vi "Main.vi"() -> ()   [LabVIEW 2013]
uses:
  MouseCarousel/Controls/TrainingProtocols.ctl
  MouseCarousel/States/DataAquisitionStates.ctl
  <vilib>/vision/Avi.llb/IMAQ AVI2 Refnum.ctl
  <vilib>/vision/Image Controls.llb/IMAQ Image.ctl
  MouseCarousel/Controls/sessionInfoAR.ctl
  MouseCarousel/Controls/dataInfo.ctl
  <vilib>/event_ctls.llb/eventsource.ctl
  Instruments/StepperController.lvclass
  D:/Labview Programs/PassiveRotationTask/trialData.ctl
  MouseCarousel/Checklists/SessionChecklist.ctl
  MouseCarousel/Checklists/OpenCarouselInitializationChecklist.ctl
  MouseCarousel/States/EventLoopStates.ctl
  MouseCarousel/States/MainProgramStates.ctl
  SecurityCamera/SecurityCameraStates.ctl
  PupilTracker/PupilTrackerStates.ctl
  RotationControl/StageLoggingStates.ctl
  MouseCarousel/States/RotationStageStates.ctl
  Utility/Load and Save Controls_LV2009.llb/RWC_Actions.ctl
  <vilib>/DAQmx/write.llb/DAQmx Write (Digital Bool 1Line 1Point).vi
  <vilib>/DAQmx/read.llb/DAQmx Read (Digital 2D U8 NChan NSamp).vi
  MouseCarousel/GlobalVariables.vi
  <vilib>/DAQmx/create/channels.llb/DAQmx Create Channel (DO-Digital Output).vi
  <vilib>/DAQmx/miscellaneous.llb/DAQmx Fill In Error Info.vi
  <vilib>/Utility/xml.llb/Write to XML File(string).vi
  <vilib>/DAQmx/create/channels.llb/DAQmx Create Channel (DI-Digital Input).vi
  <vilib>/DAQmx/configure/timing.llb/DAQmx Timing (Sample Clock).vi
  <vilib>/DAQmx/configure/task.llb/DAQmx Configure Logging (TDMS).vi
  <vilib>/Analysis/NI_AALBase.lvlib
  <vilib>/vision/NI_Vision_Development_Module.lvlib
  <resource>/objmgr/daqmx.rc
  <vilib>/DAQmx/configure/timing.llb/DAQmx Timing (Change Detection).vi
  <vilib>/DAQmx/configure/trigger.llb/DAQmx Start Trigger (Digital Edge).vi
  <vilib>/DAQmx/create/channels.llb/DAQmx Create Channel (AI-Voltage-Basic).vi
  <vilib>/DAQmx/read.llb/DAQmx Read (Counter U32 1Chan 1Samp).vi
  <vilib>/DAQmx/read.llb/DAQmx Read (Analog DBL 1Chan 1Samp).vi
  <vilib>/DAQmx/create/channels.llb/DAQmx Create Channel (CI-Position-Angular Encoder).vi
panel:
  in  "Show Mouse ROI":bool
  out "Security Camera":T1(plugin-control)
  in  "Select Mouse ROI":bool
  out "Lost Frames":bool
  out "Recording Security Video":bool caption="Recording"
  out "RecordingID":string
  out "Last Image number":u32
  out "mL Per Ms":dbl=1.25e-05
  out "trial data tdms fileref":refnum<k34>
  out "Last Count":u32
  out "Trial Distance":i32[][](array[numeric])
  in  "Is Setup Initialized":bool
  in  "Recording No":i32=1
  in  "Session Checklist":T2
  out "Trial Speeds":i32[][](array[numeric])
  in  "trialData":T3
  out "wall ref":bool
  out "Stage Moving?":bool caption="Moving?"
  out "Wall Moving?":bool caption="Moving?"
  in  "Reset":bool
  in  "Quit":bool
  in  "Print Screen":bool
  out "Stage Position":dbl caption="Position"
  out "StepperController.lvclass":refnum<class "StepperController.lvclass">
  out "Mask":T1
  out "Fitted Pupil Image 2":T1
  out "BIN Refnum - Body":refnum<file>
  out "FrameCount":dbl
  out "Refnum out (duplicate)":T1
  out "Recording Demo Video":bool=TRUE
  out "DemoVideo":T1(plugin-control)
  out "channel names":string[](array[string])=["Licks", "Beeps", "Water", "2P Frames", "LightOnOff", "Stage Position", "Stage Moving", "Wall Position", "Wall Moving", "Trial Counter", "Trial State", "Pupil Sample No"]
  out "Source":T4 items=["LabVIEW UI"=0, "ActiveX"=1, "User Event"=25]
  out "ImageSummaryPath":path
  out "Session Running":bool=TRUE
  out "Mouse entered arena":string
  out "Response Window":dbl
  out "security camera error":errorcluster
  in  "dataInfo":T5
  in  "Save Security Video":bool
  in  "Save Pupil Video":bool=TRUE
  in  "response window is open":bool=TRUE
  out "LostFrames":u32 caption="LostFrames Pupil Camera"
  out "Frame Rate Security Cam":dbl
  out "LostFrames Security Camera":u32
  out "arena_display":T1
  out "mouse":T1
  out "tmp_arena":T1
  out "tmp_mouse":T1
  out "arena":T1
  out "Paused Acquisition":bool=TRUE
  in  "ArenaState":T6={"Stage Position"=0.0, "Stage Moving?"=TRUE, "Wall Position"=0.0, "Wall Moving"=TRUE}
  in  "sessionInfo":T7
  out "GoogleDriveFolder":path
  out "RecordingFolder":path
  out "Log Stage Positions":bool=TRUE
  out "Stage Rotation Direction":bool caption="Moving?"
  in  "Block folder":path
  out "Processed Image":T1
  out "Cropped Image":T1
  out "Processed Image Display":T1
  out "Fitted Pupil Image":T1
  out "Stop Acquisition":bool=TRUE
  out "Vision Acquisition Error":errorcluster
  in  "Save Tracking Results":bool=TRUE
  out "Pupil Sample No":i32
  out "Last Image number SV":u32
  out "Mouse mask":T1
  out "AVI Refnum - Body":T8
  out "Trigger microscope":bool=TRUE
  out "2P TriggerLine":refnum<k21>
  out "SciScan RecordSignal":refnum<k21>
  out "Session Performance":i16[][](array[numeric])
  in  "PrevLickState":dbl format="%#_13g"
  out "tmpNCorrect":i32
  out "nCorrect":i32
  out "Correct?":bool
  out "Trial State":i32
  out "Recording Start Time":u32
  out "Saved Values":refnum<vi>[](array[refnum])
  out "tdms file performance":refnum<k34>
  out "Licked":bool=TRUE
  out "Response Timeout":bool=TRUE
  in  "Tab Control":T9(tab)
  out "Image Size":string
  out "Frames Lost":bool
  in  "Give Water 2":bool
  in  "Step+":bool
  in  "Step-":bool
  in  "Home":bool
  in  "Compress Avi":bool
  in  "Rotate Full":bool
  in  "Align Stage":bool
  in  "Start Protocol":bool
  in  "Selected Training Protocol":T10=enum."Rotations - Speed 45 deg/s"
  in  "Pause":bool
  in  "Open Checklist":bool
  in  "Abort Protocol":bool
  out "Image":T1(plugin-control)
  in  "Day":u16
  in  "Airpuff":bool
  in  "Mouse Entered":bool
  out "Lick Rates":i32[][](graph)
  out "Trial Performance":cluster{"D'prime":dbl, "pCorrect":dbl}(graph)
  out "Trial Outcomes":i16[](graph)
  out "Lick detection":cluster{dbl, dbl, dbl[][]}(graph)
  out "Trial Counter":i32
  out "NRewards":i32
  out "NGoTrials":i32
  out "% correct":dbl format="%#_2g"
  out "d'":dbl
  out "Last trial":i32=300
  out "SessionID":string
  in  "Give Water":bool
  in  "Lights On":bool
  in  "Mouse Number":i32
  out "Stage Position 2":T1(plugin-control)
  out "Pupil Info":T11(graph)
  out "Intertrial Interval":bool
  out "Time Delay":bool
  out "Response Window":bool
  out "Pre trial":bool
  out "Cue":bool
  out "Current trial":string caption="Trial Progression"
  out "mL given":dbl(slide) scale=0.0..1.0
  out "last response time (ms)":dbl
  out "Go Trial?":bool=TRUE
  out "NPunishments":i32
  in  "Experiment Name":string="PassiveRotationTask"
  in  "SS Crash Button":bool
  in  "MC Crash Button":bool
  out "stageStopPosition":dbl
  out "stageAcceleration":dbl
  out "Pupil marked":bool=TRUE
  out "Frame Rate Eyetracker":dbl caption="FPS"
  in  "xFactorStdThresholding":dbl=1.0 min=0.0 max=5.0 step=0.1
  in  "Automatic Threshold Update":bool
  out "Avg freq":dbl caption="Eyetracker - Mean \nprocessing frequency (Hz)" format="%0.2f"
  out "PupilCamera":T1(plugin-control)
  out "Tracking Pupil":bool
  out "Recording Pupil Video":bool=TRUE
  out "Processed":T1(plugin-control)
  in  "Manual Threshold":cluster{sgl, sgl}(slide)={196.0, 255.0} caption="Threshold Range" scale=0.0..255.0
  in  "Exposure Time":dbl(slide)=15144.329896907217 min=10.0 max=850000.0 scale=1000.0..16000.0
  in  "Gain":dbl(slide)=8.879999999999999 min=0.0 max=24.0 step=1.0 scale=0.0..24.0
  in  "Black Level":dbl(slide)=0.9896907216494839 min=-32.0 max=31.75 scale=-32.0..32.0
  in  "Track Pupil":bool
  in  "Rescan Image":bool
  in  "Acquisition Frame Rate":dbl=60.0 min=1.0 max=100000.0
  in  "Track Every Nth Frame":i32=2
  out "Auto Threshold":sgl[](array[numeric])
  out "Reset Lost Frames":bool
  in  "Select Pupil Area":bool
  in  "BtnStageSmallStep":bool
  in  "BtnWallSetHome":bool
  in  "BtnWallMoveHome":bool
  in  "Wall step size (deg)":dbl=90.0 min=-45.0 max=45.0 step=1.0
  in  "Wall Acceleration (deg2/s)":dbl=200.0 min=1.0 max=1000.0 step=1.0
  in  "Wall Speed (deg/s)":dbl=50.0 min=0.1 max=50.0 step=0.1
  in  "BtnWallStepCW":bool
  in  "BtnWallStepCCW":bool
  in  "BtnStage180CW":bool
  in  "BtnStage180CCW":bool
  in  "BtnStageMoveHome":bool
  in  "Stage step size (deg)":dbl=90.0
  in  "Stage Acceleration (deg2/s)":dbl=200.0
  in  "Stage Speed (deg/s)":dbl=50.0
  in  "BtnStageStepCW":bool
  in  "BtnStageStepCCW":bool
  in  "Move to ...":bool=TRUE
  in  "... Position":dbl
  out "Wall Position":dbl caption="Position" format="%#.2f"
  in  "BtnBothCW":bool
  in  "BtnBothCCW":bool
  in  "Save Trial Data":bool
  in  "Wall Speed Selection":dbl[](array[numeric])=[45.0, 90.0]
  in  "Stage Speed Selection":dbl[](array[numeric])=[45.0, 90.0, 135.0, 180.0]
  in  "DarkProbes":bool
  in  "Airpuff (ms)":u32=400
  in  "Always Puff":bool=TRUE
  in  "Intertrial interval (s)":i32=6
  in  "Punishment Period (s)":i32
  in  "Response Window (ms)":u32=2000
  in  "Go Trial Probability":dbl=0.5 min=0.0 max=1.0 step=0.1
  in  "nTrials":i32=100
  in  "Give water":bool
  in  "Delay (ms)":i32=500
  in  "LightsOnSession":bool=TRUE
  in  "Baseline Period (s)":i32=30
  in  "Wall-Stage delay (ms)":dbl=33.0
  in  "Wall max rotation":dbl=720.0
  in  "Wall physical step size (deg/step)":dbl=0.139
  in  "DAQmx step counter":tag="Dev1/ctr0"
  in  "DAQmx step terminal":tag="/Dev1/PFI8"
  in  "DAQmx step-dir line":tag="Dev1/port2/line1"
  in  "Save Pupil Video As...":enum16{"BIN", "PNG", "AVI"}(ring)
  in  "Save Security Video As...":enum16{"BIN", "AVI"}(ring)=enum."AVI"
  in  "DemoCamera Connected":bool caption="Demo Camera Connected"
  in  "Sampling - Labels,  Lines In":string[][](array[string])=[["Licks", "Dev1/port0/line3", "", ""], ["Airpuff", "Dev1/port0/line4", "", ""], ["Water", "Dev1/port0/line7", "", ""], ["2P Frames", "Dev1/port0/line2", "", ""], ["Light", "Dev1/port0/line0", "", ""], ["Wall Pos Reset", "Dev1/port0/line6", "Light", "Light"]]
  in  "Select Microscope":enum16{"Prairie", "SciScan"}(ring)=enum."SciScan"
  in  "Two Photon Connected":bool=TRUE caption="Two Photon Microscope"
  in  "Lick Port Connected":bool=TRUE caption="Lick Port"
  in  "Open Valve":bool
  in  "Sample Rate":dbl=5000.0 format="%#_13g"
  in  "Graph Update Rate (fps)":dbl=200.0 format="%#_13g"
  in  "Graph Length (s)":dbl=10.0 format="%#_13g"
  in  "Stage connected":bool=TRUE caption="Rotation Stage"
  in  "Calibrate Valve":bool
  in  "Valve opening time (ms)":u32=200
  in  "Number of drops to release":i32=100
  out "Valve opening time (last calibration) (ms)":u32
  out "Last Calibration Date":timestamp format="%<%H:%M:%S\n%x>T"
  out "mlPerDrop":dbl
  out "Start Data Logging":bool=TRUE
  out "Stop Data Logging":bool=TRUE
  out "Leave Acquisition Run State":T12=enum."Quit Data Acquisition"
  out "Logging Data":bool=TRUE
  in  "Security Camera Connected":bool=TRUE caption="Security Camera"
  in  "File Path for Mouse Mask":path=path "F:/RotationStageExperiments/MousePositionMask.bmp"
  in  "Select Rotation Stage":enum16{"PI", "Steinmeyer"}(ring)=enum."Steinmeyer"
  in  "Pupil Camera Connected":bool=TRUE caption="Pupil Camera"
  out "PIAxisID":string[](array[string])
  in  "Daily Summary Path":path=path "C:/Users/Eivind/Google Drive/Lab/Eivind Hennestad/Mouse Training/Round 5 - Training + imaging/DailySummaries"
  in  "Water Valve Line":tag="Dev1/port2/line3"
  in  "Airpuff Line":tag="Dev1/port2/line2"
  in  "Two-Photon trigger line":tag="Dev1/port2/line5"
  in  "SciScan Start/Stop":tag="Dev1/port1/line2"
  in  "Stage Position Limit":i32=720
  in  "Data Storage Folder":path=path "E:/NEW"
  out "Progress %":i32(slide) scale=0.0..100.0
  out "LickPerMin":i32[][](array[numeric])
  out "NLicks":i32[](array[numeric])
  in  "RoofLights":tag="Dev1/port1/line0"
  in  "Reward Punishment Ratio":u8=3
  in  "SaveDemoVideo":bool
  in  "Wall connected":bool=TRUE
  out "Stepper Prepared for Rotation":bool=TRUE
  out "Init Stepper Move":bool
  in  "Destretch Calibrate":bool
  in  "Release Air":bool
  out "Start Matlab Processing":bool
  out "Pandoras Box 2":bool
  out "Pressurized Air Supply  2":bool
  out "Encoder Splitter Power 2":bool
  in  "Startup Checklist":T13
  out "response time":u32
  out "Mouse Performance":i16[][](array[numeric])
  out "Correct Rejection":bool=TRUE
  out "Miss":bool=TRUE
  in  "Reward Green Light":bool=TRUE
  out "Reward Mode":enum16{"Reward on Cue", "Reward on Lick"}(ring)
  out "False Alarm":bool=TRUE
  out "Hit":bool=TRUE
  out "AllowReward":bool=TRUE
  out "Current Protocol":enum16{""}(ring)
  out "NDropsCalibration":i32
  out "Buffer Length":i32
  out "Samples to Read":i32
  in  "Exit Program":bool
  out "Response Times":dbl[](array[numeric])
  out "Waiting for lick":bool
  out "cue time":u32
  # "Training/Experiment"
  # "Session Info"
  # "Training Info"
  # "Hit"
  # "Correct Reject"
  # "Miss"
  # "False Alarm"
  # "Optimize Tracking"
  # "Set tracker to rescan entire image if pupil is not found within search area"
  # "Tracker Settings"
  # "Stage controls"
  # "NB! Is cable for roof light disconnected?"
  # "Wall controls"
  # "Move both"
  # "Training Parameters"
  # "Give water on \nevery go trial"
  # "Speed Modulation Sessions"
  # "Connection Settings"
  # "Equipment Selection"
  # "DAQ Connections"
  # "Settings"
  # "Acquisition"
  # "Graph Display"
  # "Data Storage Paths"
  # "Valve Calibration"
  # "Checklist Startup - Things to do before picking up mouse"
  # "Checklist Shutdown"
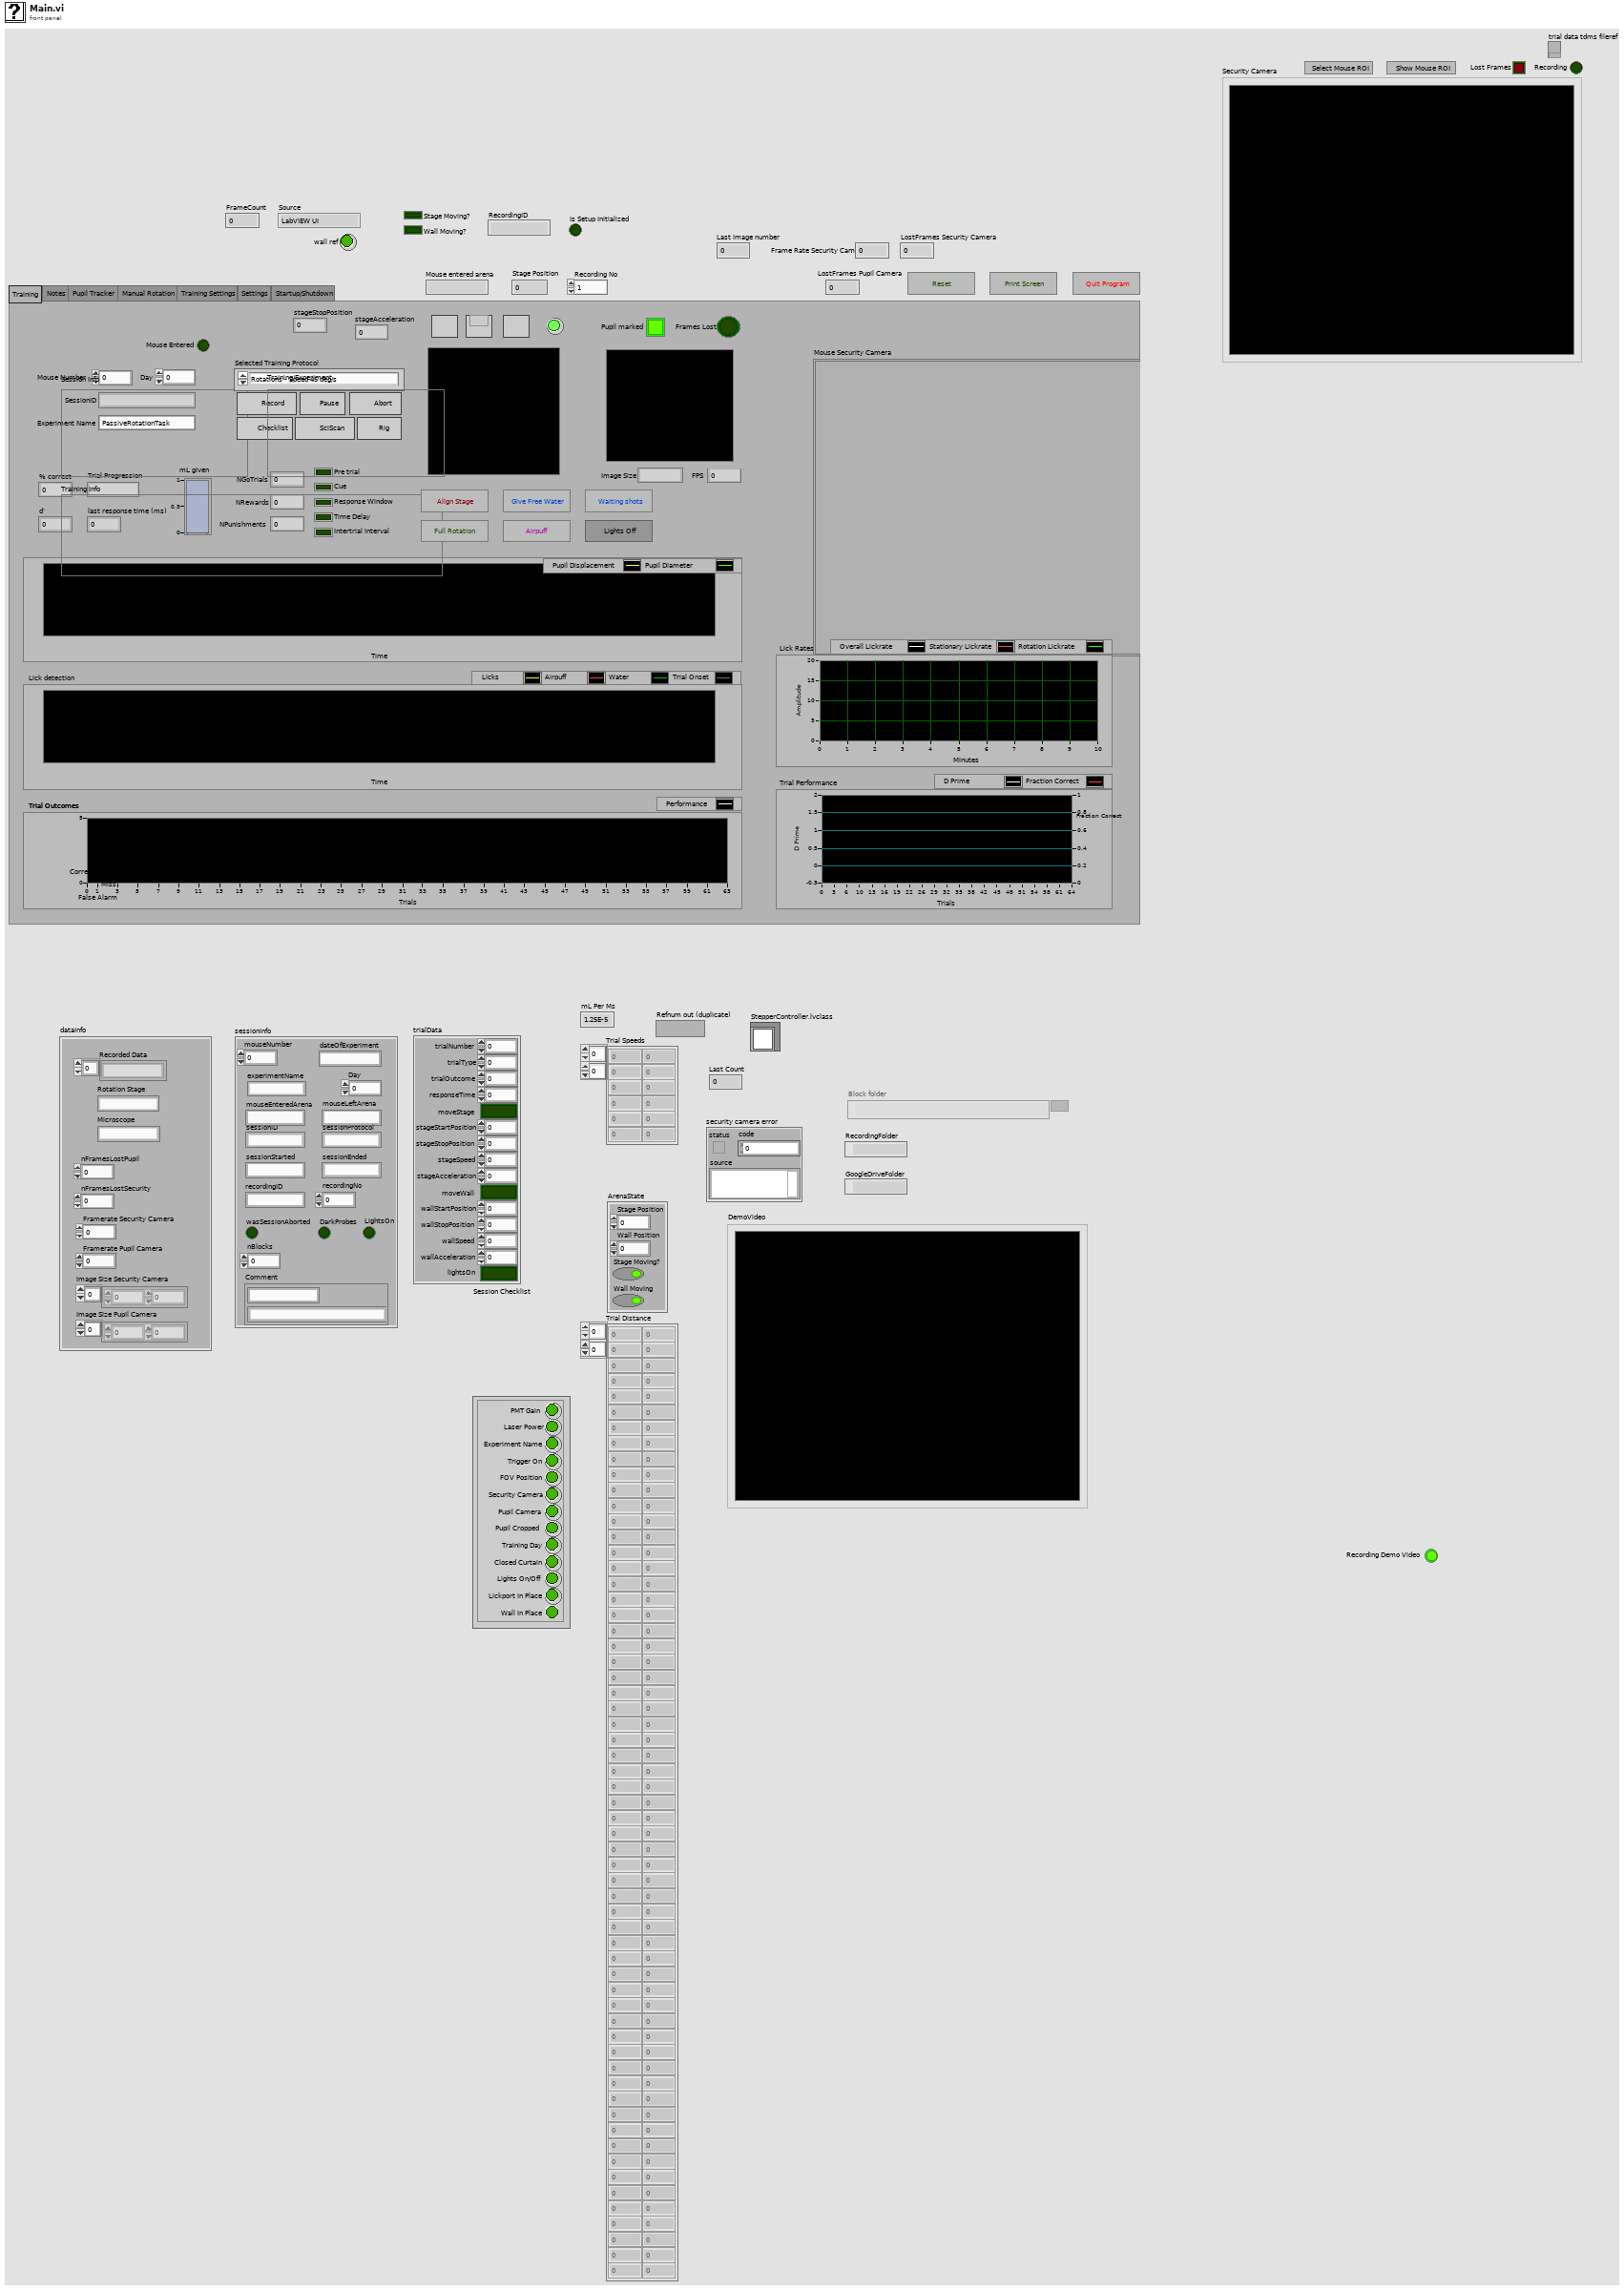
[diagram p1: front panel]
types:
  T1 = typedef "IMAQ Image.ctl" = refnum<image>
  T2 = typedef "SessionChecklist.ctl" = cluster{"PMT Gain":bool, "Laser Power":bool, "Experiment Name":bool, "Trigger On":bool, "FOV Position":bool, "Security Camera":bool, "Pupil Camera":bool, "Pupil Cropped":bool, "Training Day":bool, "Closed Curtain":bool, "Lights On/Off":bool, "Lickport In Place":bool, "Wall In Place":bool}
  T3 = typedef "trialData.ctl" = cluster{"trialNumber":i32, "trialType":i32, "trialOutcome":i32, "responseTime":i32, "moveStage":bool, "stageStartPosition":dbl, "stageStopPosition":dbl, "stageSpeed":dbl, "stageAcceleration":dbl, "moveWall":bool, "wallStartPosition":dbl, "wallStopPosition":dbl, "wallSpeed":dbl, "wallAcceleration":dbl, "lightsOn":bool}
  T4 = typedef "eventsource.ctl" = u32
  T5 = typedef "dataInfo.ctl" = cluster{"Recorded Data":string[], "Rotation Stage":string, "Microscope":string, "nFramesLostPupil":u32, "nFramesLostSecurity":u32, "Framerate Security Camera":dbl, "Framerate Pupil Camera":dbl, "Image Size Security Camera":i32[], "Image Size Pupil Camera":i32[]}
  T6 = cluster{"Stage Position":dbl, "Stage Moving?":bool, "Wall Position":dbl, "Wall Moving":bool}
  T7 = typedef "sessionInfoAR.ctl" = cluster{"mouseNumber":i32, "dateOfExperiment":string, "experimentName":string, "Day":u16, "mouseEnteredArena":string, "mouseLeftArena":string, "sessionID":string, "sessionProtocol":string, "sessionStarted":string, "sessionEnded":string, "recordingID":string, "recordingNo":i32, "wasSessionAborted":bool, "DarkProbes":bool, "LightsOn":bool, "nBlocks":i32, "Comment":cluster{"Title":string, "Comment":string}}
  T8 = typedef "IMAQ AVI2 Refnum.ctl" = refnum<k20>
  T9 = enum32{"Training", "Notes", "Pupil Tracker", "Manual Rotation", "Training Settings", "Settings", "Startup/Shutdown"}
  T10 = typedef "TrainingProtocols.ctl" = enum16{"Prerecording", "PRT Stage - 3Pos - 2Speeds", "PRT Wall - 3Pos - 2Speeds", "Rotations - Speed 45 deg/s", "Rotations - Speed 90 deg/s", "Wall Rotations - Speed 45deg/s", "Speed Modulation - Constant Duration", "Speed Modulation - Constant Distance", "Speed Modulation - Dark - Constant Distance", "Speed Modulation - Wall - Constant Distance", "Start-Stop", "Start-Stop-90", "4Accelerations", "Rotations - Random speeds", "Open Arena - Small Steps 2", "Open Arena - Small Steps", "Rotations - 240deg 60deg/s", "Free Water"}
  T11 = cluster{"Numeric":dbl, "Average of last N array elements":dbl}
  T12 = typedef "DataAquisitionStates.ctl" = enum16{"Init Data Acquisition", "Start Data Logging", "End Data Logging", "Run Data Acquisition", "Quit Data Acquisition"}
  T13 = typedef "OpenCarouselInitializationChecklist.ctl" = cluster{"Encoder Splitter Power":bool, "Pandoras Box":bool, "Water and Calibration":bool, "Vacuum Arena":bool, "Wall Power Supply":bool, "Wall Position Encoder":bool, "Stage Power Supply":bool}
  T14 = typedef "RotationStageStates.ctl" = enum16{"Connect Stage", "Get Stage Info", "Disconnect Stage"}
  T15 = typedef "StageLoggingStates.ctl" = enum16{"Initialize Arena State Logging", "Idle", "SteinmeyerV2", "Steinmeyer", "PI", "Logging Error"}
  T16 = typedef "PupilTrackerStates.ctl" = enum16{"Initialize Eyetracker", "Idle", "Run Acquisition", "Update Acquisition Parameters", "Camera Error", "Pupil Unmarked Error", "Quit Eyetracker"}
  T17 = typedef "SecurityCameraStates.ctl" = enum16{"Init Security Camera", "Idle", "Process Image", "Acquire Image", "Disconnect Camera", "Exit"}
  T18 = typedef "MainProgramStates.ctl" = enum16{"Init Main Program", "Load Modules", "Idle", "Reset Parameters", "Start Recording", "Init Training Protocol", "Baseline Period", "Trial Initialization", "Move Stage / Wall", "Cue", "Response Window", "Time Delay (Punishment)", "Intertrial Interval", "End Training Protocol", "End Recording", "Reset Session Data", "Pause", "Calibrate Water Valve", "Quit Main Program"}
  T19 = typedef "EventLoopStates.ctl" = enum16{"Init Event Loop", "Running", "Quit Event Loop"}
  T20 = typedef "Image Type" = u32
  T21 = cluster{"EOF Change Detection Task":refnum<k21>, "EOF Event":refnum<event-registration>}
  T22 = enum8{"Enabled", "Disabled", "Disabled and Grayed Out"}
  T23 = typedef "RWC_Actions.ctl" = enum16{"Read", "Write", "Read and Create"}
  T24 = enum16{"open", "open or create", "create or replace", "create", "open (read-only)"}
  T25 = enum16{"open", "replace", "create", "open or create", "replace or create", "replace or create with confirmation"}
  T26 = cluster{"Water Valve":refnum<k21>, "Airpuff":refnum<k21>, "Light Switch":refnum<k21>}
  T27 = enum32{"Invalid", "Standard", "Closed", "Hidden", "Minimized", "Maximized"}
  T28 = enum32{"Bad", "Idle", "Run top level", "Running"}
  T29 = typedef "IMAQ Rectangle" = cluster{"Left":i32, "Top":i32, "Right":i32, "Bottom":i32, "Rotation":dbl}
  T30 = cluster{"Numeric":dbl, "Average of last N array elements":dbl}[]
  T31 = typedef "TrackingParameters.ctl" = cluster{"Frame No":i32, "Circle time series":dbl[][], "Rectangle coordinates":i32[], "Annulus ROI":cluster{"ID":enum32{"External", "Internal"}, "Type":u32, i32[]}, "Initial Annulus":i32[], "Auto Threshold":sgl[], "Automatic Threshold Update":bool, "Initial Threshold":sgl[], "mFactorStd":dbl}
  T32 = cluster{"Pupil Displacement":dbl, "Average Pupil Diameter":dbl}
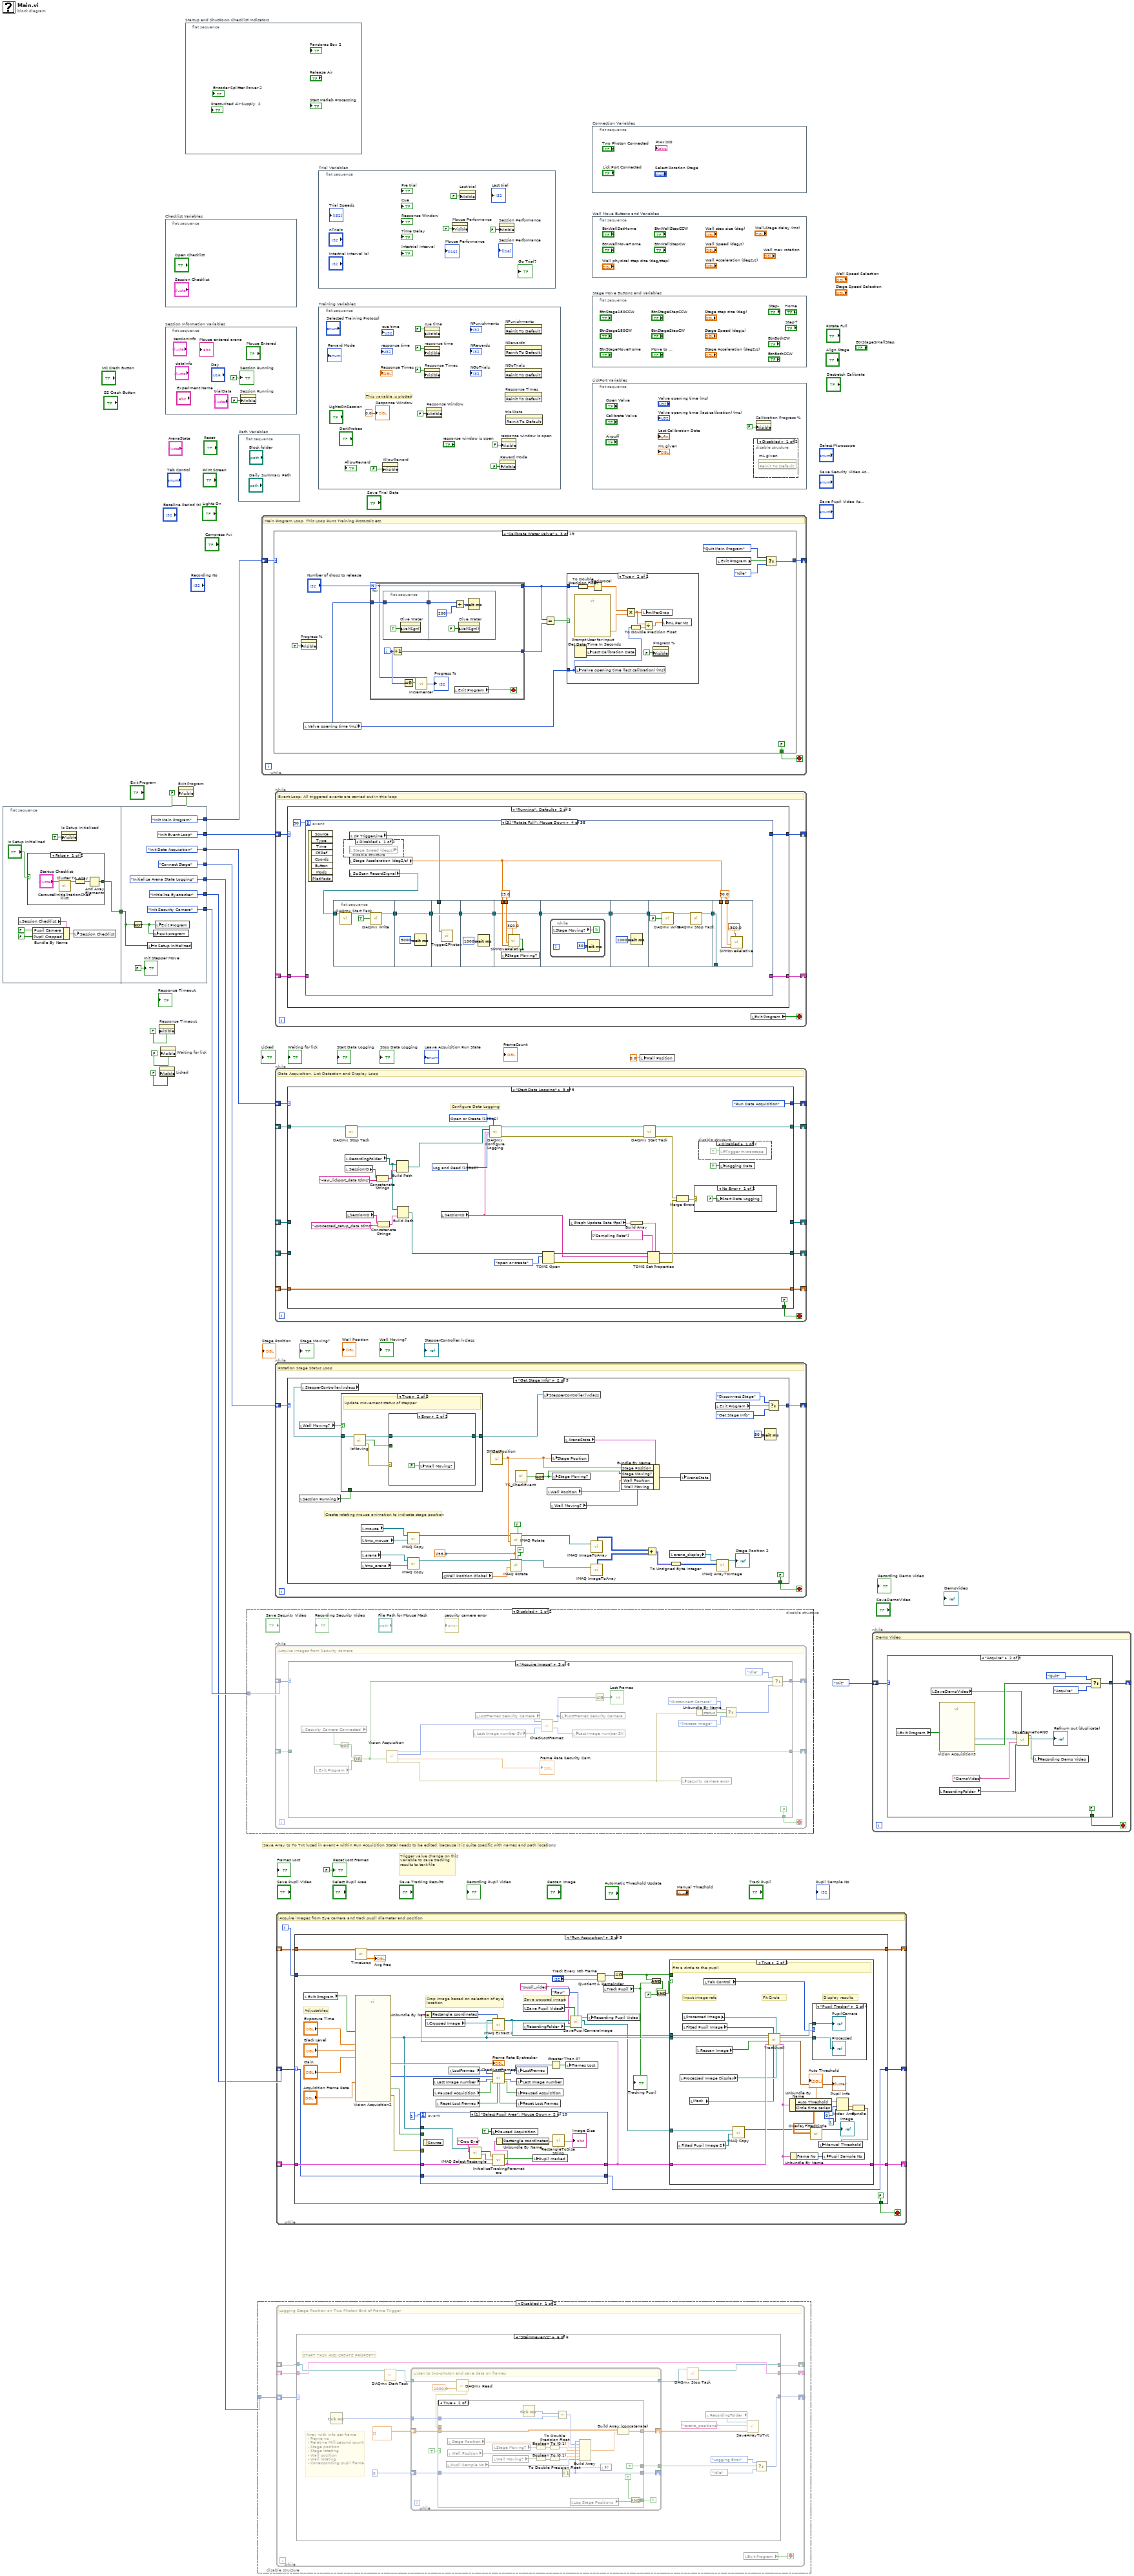
[diagram p0: block diagram]
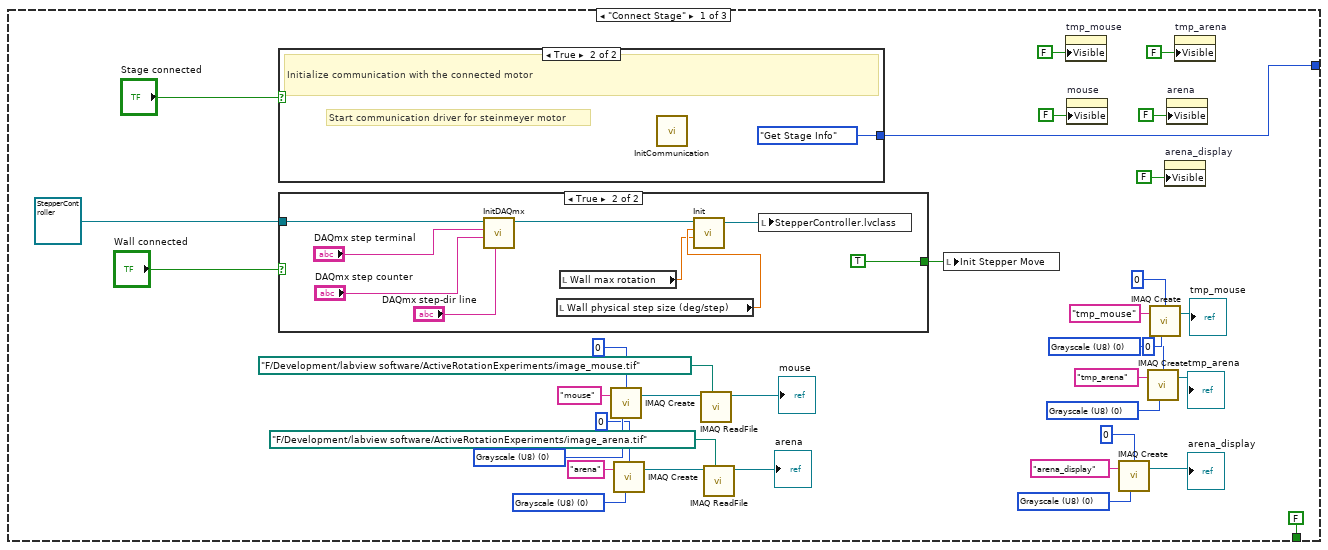
[diagram p2: hidden frame]
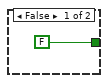
[diagram p3: hidden frame]
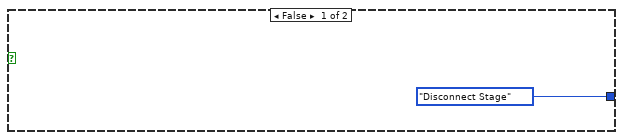
[diagram p4: hidden frame]
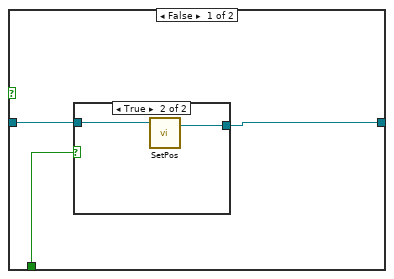
[diagram p5: hidden frame]
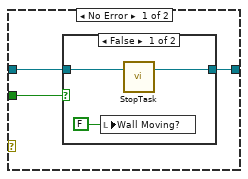
[diagram p7: hidden frame]
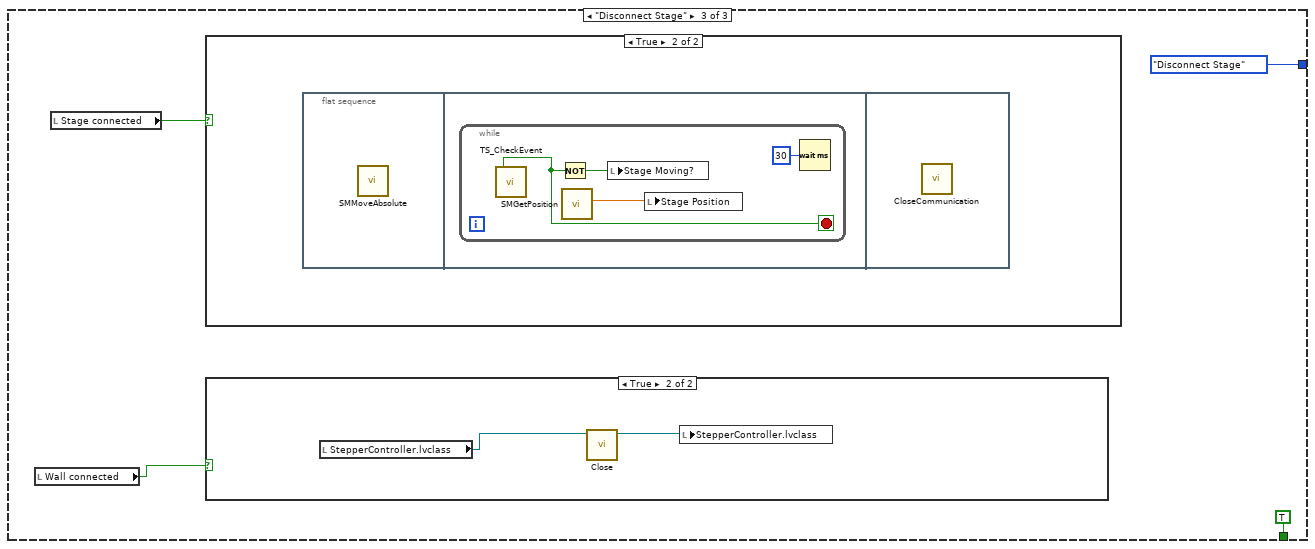
[diagram p9: hidden frame]
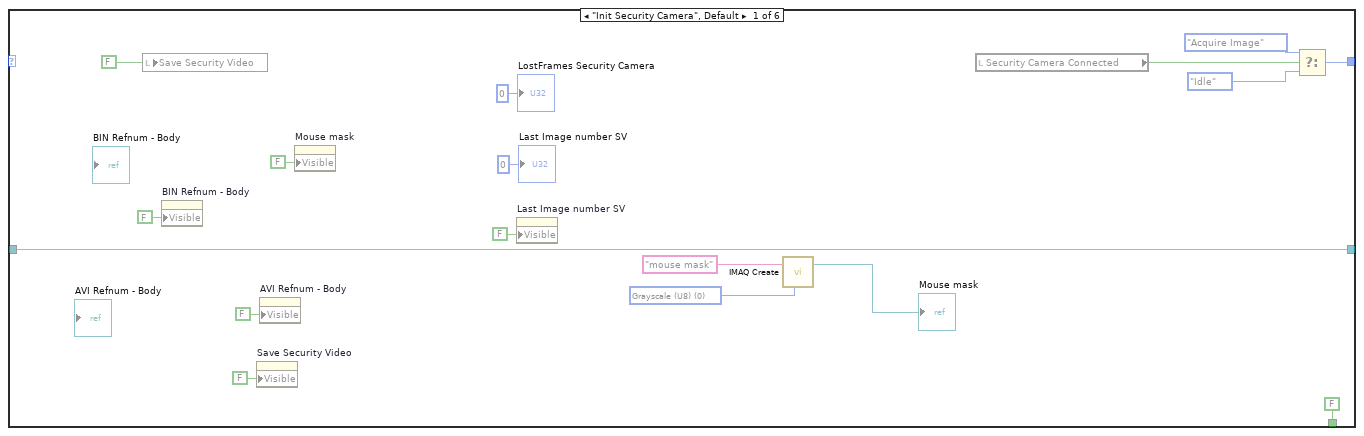
[diagram p12: hidden frame]
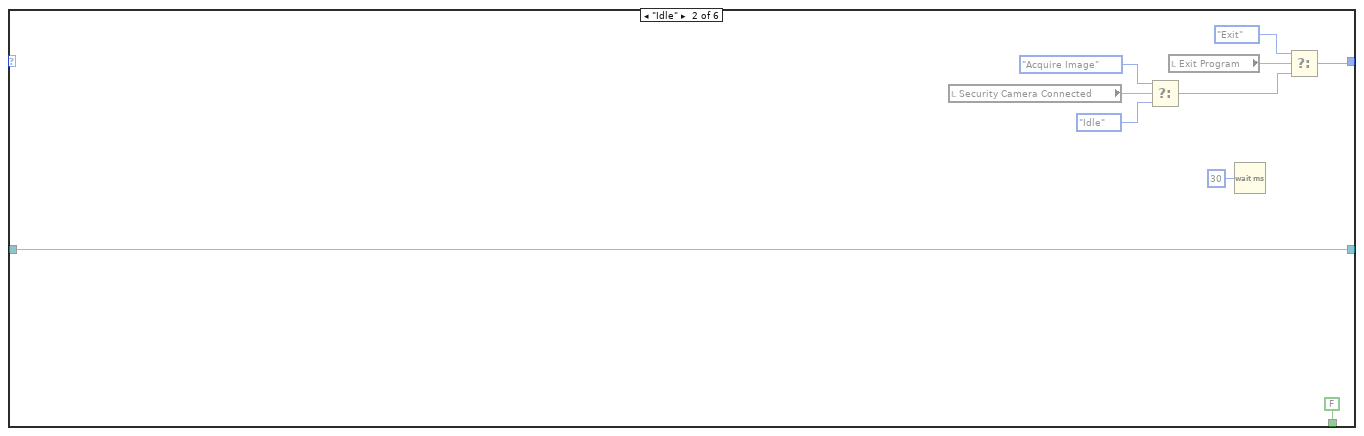
[diagram p13: hidden frame]
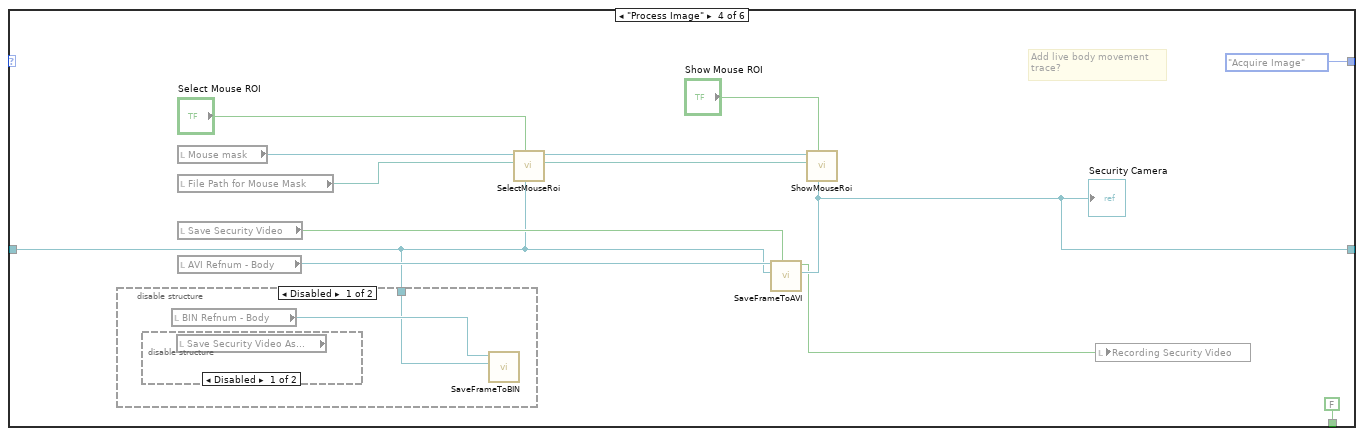
[diagram p14: hidden frame]
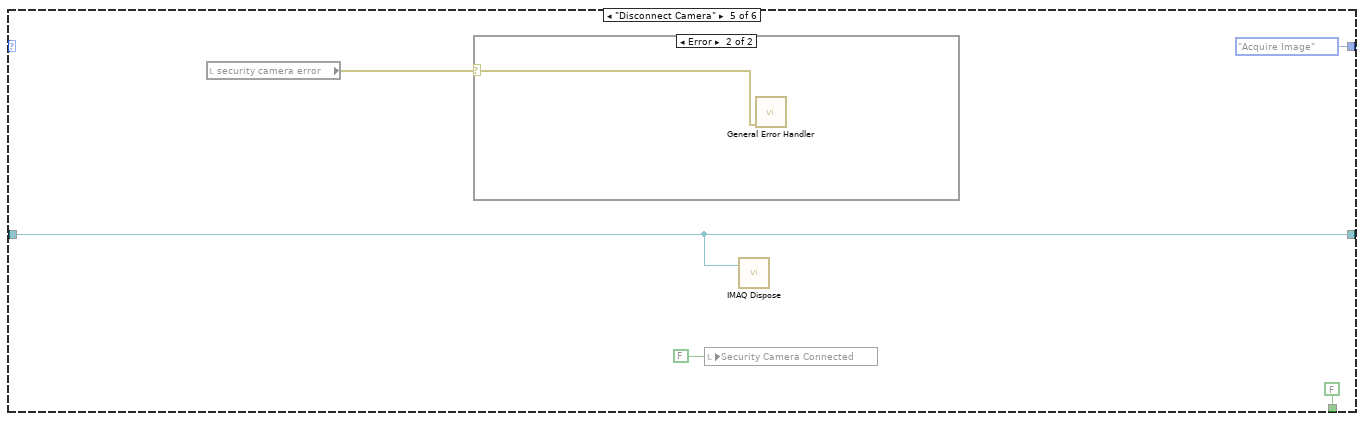
[diagram p17: hidden frame]
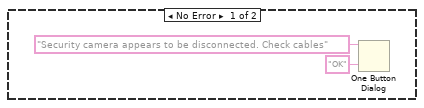
[diagram p18: hidden frame]
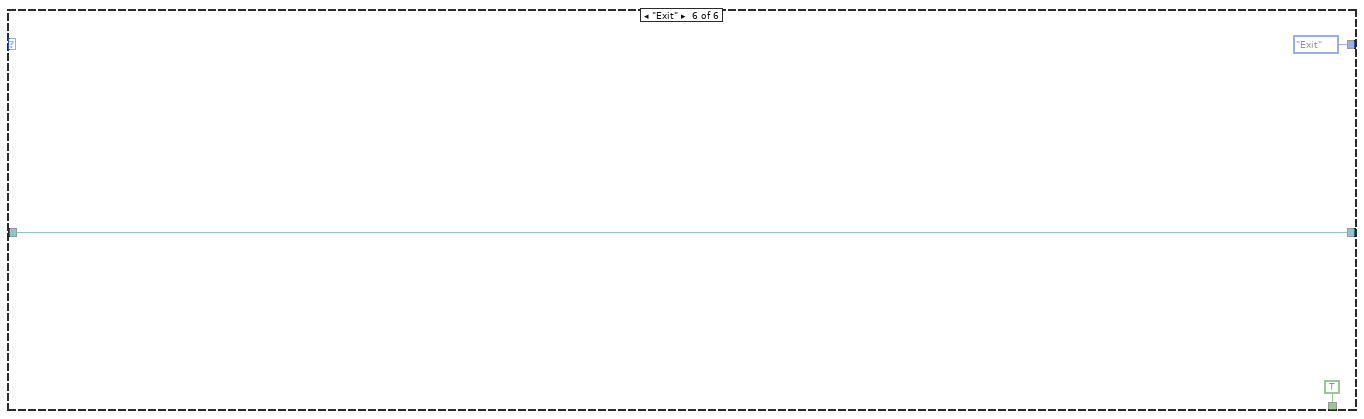
[diagram p19: hidden frame]
diagram:
  # "Save Array to To Txt (used in event 4 within Run Acquisition State) needs to be edited, because it is quite specific with names and path locations"
  # "Trigger value change on this variable to save tracking results to text file"
  n1 = flat-sequence {
    tunnel: [w21] -> w3
    tunnel: [EventLoopStates."Init Event Loop"] -> w15
    tunnel: [DataAquisitionStates."Init Data Acquisition"] -> w14
    tunnel: [MainProgramStates."Init Main Program"] -> w13
    tunnel: [SecurityCameraStates."Init Security Camera" ("States")] -> w8
    tunnel: [StageLoggingStates."Initialize Arena State Logging"] -> w7
    tunnel: [PupilTrackerStates."Initialize Eyetracker"] -> w6
    tunnel: w3 -> [w29]
    tunnel: [RotationStageStates."Connect Stage"] -> w2
    frame #0 {
      n2 = local read "Session Checklist"() -> (w19:T2)
      n3 = case shown="False" "Is Setup Initialized" {
        selector: "Is Setup Initialized" -> [_ w27]
        tunnel: [w25 w27] -> w21
        frame False {
          n4 = call "CarouselInitializationChecklist.vi"("Startup Checklist In"="Startup Checklist") -> ("Startup Checklist Out"=w23:T13)  [unwired: 10 in]
          n5 = Cluster To Array(cluster=w23) -> (array=w26:bool[])
          n6 = And Array Elements(Boolean array=w26) -> (logical AND=w25:bool)
        }
        frame True {
        }
      }
      n7 = Bundle By Name(cluster=w19, "Pupil Camera"=FALSE, "Pupil Cropped"=FALSE) -> (w18:T2)
      n8 = property on="Is Setup Initialized" class="Bool (strict)"("Visible"=TRUE) -> ()  [unwired: 2 in, 2 out]
      n9 = local write "Session Checklist"(w18) -> ()
    }
    frame #1 {
      n10 = Not(x=w29) -> (.not. x?=w28:bool)
      n11 = local write "Is Setup Initialized"(w29) -> ()
      n12 = global write "GlobalVariables.vi" "quit program"(w28) -> ()
      n13 = local write "Exit Program"(w28) -> ()
      "Init Stepper Move" <- FALSE ("Init Stepper Move")
    }
  }
  n14 = property on="Response Timeout" class="Bool (strict)"("Visible"=FALSE) -> ()  [unwired: 2 in, 2 out]
  n15 = property on="Licked" class="Bool (strict)"("Visible"=FALSE) -> ()  [unwired: 2 in, 2 out]
  n16 = property on="Waiting for lick" class="Bool (strict)"("Visible"=FALSE) -> ()  [unwired: 2 in, 2 out]
  n17 = flat-sequence "Checklist Variables" {
    frame #0 {
    }
  }
  n18 = flat-sequence "Session Information Variables" {
    frame #0 {
      n19 = property on="Session Running" class="Bool (strict)"("Visible"=FALSE) -> ()  [unwired: 2 in, 2 out]
      "Session Running" <- FALSE ("Session Running")
    }
  }
  n20 = property on="Exit Program" class="Bool (strict)"("Visible"=FALSE) -> ()  [unwired: 2 in, 2 out]
  n21 = flat-sequence "Startup and Shutdown Checklist Indicators" {
    frame #0 {
    }
  }
  n22 = flat-sequence "Path Variables" {
    frame #0 {
    }
  }
  n23 = disable-structure shown="Disabled" {
    disable-tunnel: w8 -> [w40 _]
    frame Disabled {
      n24 = while {
        shift-right: [w44] -> _
        shift-left: w40 -> [w45]
        shift-right: [w42] -> _
        shift-left: _ -> [w41]
        stop <- w43 stop-if-true
        # "Acquire images from Security camera"
        n25 = case shown="\"Acquire Image\"" w45 {
          tunnel: [w57 w66 w86 SecurityCameraStates."Acquire Image" ("States") SecurityCameraStates."Acquire Image" ("States") SecurityCameraStates."Exit" ("States")] -> w44
          tunnel: [FALSE FALSE FALSE FALSE FALSE TRUE] -> w43
          tunnel: [w49 w63 w77 w94 w106 w114] -> w42
          tunnel: w41 -> [w49 w63 _ w95 w106 w114]
          frame "Init Security Camera", Default {
            w52 = T20 0 items=["Grayscale (U8)", "Grayscale (I16)", "Grayscale (SGL)", "Complex (CSG)", "RGB (U32)", "HSL (U32)", "RGB (U64)", "Grayscale (U16)"] ("Image Type")
            n26 = local write "Save Security Video"(FALSE ("Save Block Video")) -> ()
            n27 = property on="BIN Refnum - Body" class="Ref (strict)"("Visible"=FALSE) -> ()  [unwired: 2 in, 2 out]
            n28 = property on="Save Security Video" class="Bool (strict)"("Visible"=FALSE) -> ()  [unwired: 2 in, 2 out]
            n29 = property on="AVI Refnum - Body" class="IMAQAVI (strict)"("Visible"=FALSE) -> ()  [unwired: 2 in, 2 out]
            n30 = property on="Mouse mask" class="IMAQImage (strict)"("Visible"=FALSE) -> ()  [unwired: 2 in, 2 out]
            n31 = property on="Last Image number SV" class="DigNum (strict)"("Visible"=FALSE) -> ()  [unwired: 2 in, 2 out]
            n32 = call "IMAQ Create"("Image Name"="mouse mask", "Image Type"=w52) -> ("New Image"=→"Mouse mask":T1)  [unwired: 3 in, 1 out]
            n33 = local read "Security Camera Connected"() -> (w46:bool)
            n34 = Select(t=SecurityCameraStates."Acquire Image" ("States"), s=w46, f=SecurityCameraStates."Idle" ("States")) -> (s? t:f=w57:T17)
            "LostFrames Security Camera" <- u32 0 ("LostFrames Security Camera")
            "Last Image number SV" <- u32 0 ("Last Image number SV")
          }
          frame "Idle" {
            n35 = local read "Security Camera Connected"() -> (w71:bool)
            n36 = Select(t=SecurityCameraStates."Acquire Image" ("States"), s=w71, f=SecurityCameraStates."Idle" ("States")) -> (s? t:f=w65:T17)
            n37 = local read "Exit Program"() -> (w67:bool)
            n38 = Wait (ms)(milliseconds to wait=u32 30) -> ()  [unwired: 1 out]
            n39 = Select(t=SecurityCameraStates."Exit" ("States"), s=w67, f=w65) -> (s? t:f=w66:T17)
          }
          frame "Acquire Image" {
            n40 = local read "Security Camera Connected"() -> (w75:bool)
            n41 = local read "Exit Program"() -> (w76:bool)
            n42 = Not(x=w75) -> (.not. x?=w74:bool)
            n43 = Or(x=w74, y=w76) -> (x .or. y?=w73:bool)
            n44 = call "Vision Acquisition"("Stop (F)"=w73) -> ("Image Out"=w77:T1, "Image Number"=w89:i32, "Frame Rate"=→"Frame Rate Security Cam":dbl, "error out"=w82:errorcluster)  [unwired: 21 in, 2 out]
            n45 = local read "Last Image number SV"() -> (w88:u32)
            n46 = local read "LostFrames Security Camera"() -> (w90:u32)
            n47 = call "CheckLostFrames.vi"("Last Image number"=w88, "Image Number"=w89, "LostFrames in"=w90) -> ("Last Image Number"=w91:u32, "LostFrames out"=w84:u32)  [unwired: 5 in, 2 out]
            n48 = local write "LostFrames Security Camera"(w84) -> ()
            n49 = local write "Last Image number SV"(w91) -> ()
            n50 = Not Equal To 0?(x=w84) -> (x != 0?=→"Lost Frames":bool)
            n51 = local write "security camera error"(w82) -> ()
            n52 = Unbundle By Name(w82) -> ("status"=w81:bool)
            n53 = Select(t=SecurityCameraStates."Disconnect Camera" ("States"), s=w81, f=SecurityCameraStates."Process Image" ("States")) -> (s? t:f=w78:T17)
            n54 = Select(t=SecurityCameraStates."Idle" ("States"), s=w73, f=w78) -> (s? t:f=w86:T17)
          }
          frame "Process Image" {
            # "Add live body movement\ntrace?"
            n55 = disable-structure shown="Disabled" {
              disable-tunnel: w95 -> [w104 _]
              frame Disabled {
                n56 = disable-structure shown="Disabled" {
                  frame Disabled {
                    n57 = local read "Save Security Video As..."() -> ()  [unwired: 1 out]
                  }
                  frame Enabled {
                  }
                }
                n58 = local read "BIN Refnum - Body"() -> (w105:refnum<file>)
                n59 = call "SaveFrameToBIN.vi"("IMAQ refnum in"=w104, "BIN Refnum in"=w105) -> ()  [unwired: 7 in, 3 out]
              }
              frame Enabled {
              }
            }
            n60 = local read "Mouse mask"() -> (w102:T1)
            n61 = local read "File Path for Mouse Mask"() -> (w103:path)
            n62 = local read "Save Security Video"() -> (w96:bool)
            n63 = local read "AVI Refnum - Body"() -> (w97:T8)
            n64 = call "SelectMouseRoi.vi"("Refnum in"=w95, "Select mouse"="Select Mouse ROI", "File Path for Mouse Mask"=w103, "MouseRoi"=w102) -> ()  [unwired: 7 in, 1 out]
            n65 = call "SaveFrameToAVI.vi"("Save Video"=w96, "IMAQ refnum in"=w95, "AVI Refnum in"=w97) -> ("Image Out (duplicate)"=w94:T1, "ImageSaved"=w93:bool)  [unwired: 7 in]
            "Security Camera" <- w94
            n66 = call "ShowMouseRoi.vi"("Refnum Image In"=w94, "Show mouse selection"="Show Mouse ROI", "File Path for Mouse Mask"=w103, "Refnum MouseROI"=w102) -> ()  [unwired: 7 in, 1 out]
            n67 = local write "Recording Security Video"(w93) -> ()
          }
          frame "Disconnect Camera" {
            n68 = local read "security camera error"() -> (w107:errorcluster)
            n69 = case shown="Error" w107 {
              selector: w107 -> [_ w113]
              frame No Error {
                n70 = One Button Dialog(message="Security camera appears to be disconnected. Check cables", button name ("OK")="OK") -> ()  [unwired: 1 out]
              }
              frame Error {
                n71 = call <vilib>:"General Error Handler.vi"("error in (no error)"=w113) -> ()  [unwired: 10 in, 5 out]
              }
            }
            n72 = local write "Security Camera Connected"(FALSE ("Eye Tracking Camera")) -> ()
            n73 = call "IMAQ Dispose"("Image"=w106) -> ()  [unwired: 5 in, 1 out]
          }
          frame "Exit" {
          }
        }
      }
    }
    frame Enabled {
    }
  }
  n74 = disable-structure shown="Disabled" {
    disable-tunnel: w7 -> [w117 _]
    frame Disabled {
      n75 = while {
        shift-right: [w123] -> _
        shift-left: w117 -> [w124]
        shift-right: [w121] -> _
        shift-left: _ -> [w120]
        shift-right: [w119] -> _
        shift-left: _ -> [w118]
        stop <- w122 stop-if-true
        # "Logging Stage Position on Two Photon End of Frame Trigger"
        n76 = case shown="\"SteinmeyerV2\"" w124 {
          selector: w124 -> [_ w149 _ w217 _ _]
          tunnel: [StageLoggingStates."Idle" w148 w159 w217 StageLoggingStates."Idle" w277] -> w123
          tunnel: [w136 w147 w165 w216 w270 w273] -> w121
          tunnel: w120 -> [_ w147 w164 w216 w270 w273]
          tunnel: [w135 w145 w155 w213 w267 w272] -> w119
          tunnel: w118 -> [_ w145 w155 w213 w267 w271]
          frame "Initialize Arena State Logging", Default {
            w129 = 10123 items=["Finite Samples"=10178, "Continuous Samples"=10123, "Hardware Timed Single Point"=12522] ("sample mode")
            w133 = T21 {"EOF Change Detection Task"="", "EOF Event"=refnum}  # Position Counting by Event reg
            w130 = tag "Dev1/port0/line7" ("lines")
            w134 = 12511 items=["Sample Complete Event"=12530, "Counter Output Event"=12494, "Change Detection Event"=12511, "Sample Clock"=12487] ("signalType")
            # "Register Event"
            # "Set up Change Detection task"
            # "Microscope EOF TTL line"
            n77 = disable-structure shown="Disabled" {
              disable-tunnel: [w138 _] -> w135
              frame Disabled {
                w139 = 10280 items=["Rising"=10280, "Falling"=10171] ("edge")
                n78 = property on="Log Stage Positions" class="Bool (strict)"("Visible"=FALSE) -> ()  [unwired: 2 in, 2 out]
                n79 = local write "Log Stage Positions"(FALSE ("Log Stage Positions")) -> ()
                n80 = call-poly <vilib>:"DAQmx Create Virtual Channel.vi"("physical channels"=tag "Dev1/ai5") -> ("task out"=w141:refnum<k21>)  [unwired: 13 in, 1 out]
                n81 = call-poly <vilib>:"DAQmx Trigger.vi"("task/channels in"=w141, "source"=tag "/Dev1/PFI12", "edge"=w139) -> ("task out"=w138:refnum<k21>)  [unwired: 11 in, 1 out]
              }
              frame Enabled {
              }
            }
            n82 = call-poly <vilib>:"DAQmx Create Virtual Channel.vi"("lines"=w130) -> ("task out"=w131:refnum<k21>)  [unwired: 13 in, 1 out]
            n83 = call-poly <vilib>:"DAQmx Timing.vi"("task/channels in"=w131, "sample mode"=w129, "rising edge physical channels"=w130) -> ("task out"=w128:refnum<k21>)  [unwired: 11 in, 1 out]
            n84 = call <vilib>:"DAQmx Configure Input Buffer.vi"("task/channels in"=w128, "buffer size (in samples per channel)"=u32 0) -> ("task out"=w126:refnum<k21>)  [unwired: 12 in, 1 out]
            n85 = register-events(w126, w134) -> (reference out=w132:refnum<event-registration>)  [unwired: 2 in, 1 out]
            n86 = Bundle By Name(cluster=w133, "EOF Change Detection Task"=w126, "EOF Event"=w132) -> (w136:T21)
            n87 = property on="Stage Rotation Direction" class="Bool (strict)"("Visible"=FALSE) -> ()  [unwired: 2 in, 2 out]
          }
          frame "Idle" {
            n88 = disable-structure shown="Disabled" {
              frame Disabled {
                n89 = local read "Select Rotation Stage"() -> (w152:enum16{"PI", "Steinmeyer"})
                n90 = case shown="\"Steinmeyer\"" w152 {
                  tunnel: [StageLoggingStates."PI" StageLoggingStates."Steinmeyer"] -> _
                  frame "PI", Default {
                  }
                  frame "Steinmeyer" {
                  }
                }
              }
              frame Enabled {
              }
            }
            n91 = local read "Log Stage Positions"() -> (w151:bool)
            n92 = Select(t=StageLoggingStates."Steinmeyer", s=w151, f=w149) -> (s? t:f=w148:T15)
            n93 = Wait (ms)(milliseconds to wait=u32 30) -> ()  [unwired: 1 out]
          }
          frame "Steinmeyer" {
            # "Array with info per frame\n - Frame no\n - Relative Millisecond count\n - Stage position\n - Stage rotating\n - Wall position\n - Wall rotating\n - Corresponding pupil frame"
            # "START TASK AND CREATE PROPERTY"
            n94 = Unbundle By Name(w164) -> ("EOF Change Detection Task"=w168:refnum<k21>, "EOF Event"=w171:refnum<event-registration>)
            n95 = Tick Count (ms)() -> (millisecond timer value=w160:u32)
            n96 = call <vilib>:"DAQmx Start Task.vi"("task/channels in"=w168) -> ("task out"=w166:refnum<k21>)  [unwired: 13 in, 1 out]
            n97 = while {
              shift-right: [w184] -> w161
              shift-left: dbl[][] [] -> [w183]
              shift-right: [w185] -> _
              shift-left: 0 -> [w187]
              tunnel: w166 -> [w181]
              tunnel: w171 -> [w180]
              tunnel: [w182] -> w169
              tunnel: [w181] -> w167
              tunnel: w160 -> [w179]
              tunnel: [w174] -> w156
              i -> [w175]
              stop <- w178 continue-if-true
              # "Listen to two-photon and save data on frames"
              n98 = event shown="[1] <task out>: Signal" {
                selector: w180 -> [_ _]
                dyn-events: [_ _] -> w182
                timeout: 20000 -> [_ _]
                tunnel: [w192 w211] -> w184
                tunnel: w187 -> [w193 w212]
                tunnel: [w193 w199] -> w185
                tunnel: w183 -> [w192 w209]
                tunnel: w179 -> [_ w198]
                tunnel: [FALSE TRUE] -> w176
                tunnel: w175 -> [w189 _]
                tunnel: [w188 FALSE] -> w174
                event Timeout {
                  n99 = event-data() -> ()  [unwired: 1 in, 1 out]
                  n100 = Equal To 0?(x=w189) -> (x = 0?=w188:bool)
                  n101 = local write "Log Stage Positions"(FALSE ("Log Stage Positions")) -> ()
                }
                event Signal {
                  n102 = event-data() -> ()  [unwired: 1 in, 1 out]
                  n103 = local read "Pupil Sample No"() -> (w200:i32)
                  n104 = local read "Stage Position"() -> (w208:dbl)
                  n105 = local read "Wall Position"() -> (w204:dbl)
                  n106 = local read "Stage Moving?"() -> (w206:bool)
                  n107 = local read "Wall Moving?"() -> (w202:bool)
                  n108 = Tick Count (ms)() -> (millisecond timer value=w197:u32)
                  n109 = Boolean To (0,1)(Boolean=w206) -> (0, 1=w207:i16)
                  n110 = Boolean To (0,1)(Boolean=w202) -> (0, 1=w203:i16)
                  n111 = To Double Precision Float(number=w207) -> (double precision float=w205:dbl)
                  n112 = To Double Precision Float(number=w203) -> (double precision float=w201:dbl)
                  n113 = Subtract(x=w197, y=w198) -> (x-y=w196:u32)
                  n114 = Increment(x=w212) -> (x+1=w199:i32)
                  n115 = Build Array(w199, w196, w208, w205, w204, w201, w200) -> (w210:dbl[])
                  n116 = local write item#-1(w199) -> ()
                  n117 = Build Array (concatenate)(w209, w210) -> (w211:dbl[][])
                }
              }
              n118 = local read "Log Stage Positions"() -> (w177:bool)
              n119 = And(x=w176, y=w177) -> (x .and. y?=w178:bool)
            }
            n120 = call <vilib>:"DAQmx Stop Task.vi"("task/channels in"=w167) -> ("task out"=w170:refnum<k21>)  [unwired: 13 in, 1 out]
            n121 = local read "RecordingFolder"() -> (w162:path)
            n122 = Bundle By Name(cluster=w164, "EOF Change Detection Task"=w170, "EOF Event"=w169) -> (w165:T21)
            n123 = call "SaveArrayToTxt.vi"("Input array"=w161, "Filename"="-arena_positions", "File path"=w162) -> ()  [unwired: 1 in, 1 out]
            n124 = Select(t=StageLoggingStates."Logging Error", s=w156, f=StageLoggingStates."Idle") -> (s? t:f=w159:T15)
          }
          frame "PI" {
            n125 = feedback #1() -> (w214:dbl[][])  [unwired: 1 in]
            n126 = disable-structure shown="Disabled" {
              disable-tunnel: [w226 _] -> _
              disable-tunnel: [w220 _] -> _
              disable-tunnel: w214 -> [_ _]
              disable-tunnel: [w218 _] -> w215
              frame Disabled {
                w218 = dbl[][] []
                # "Array with info per frame\n - Frame no\n - Millisecond count\n - Stage position\n - Stage rotating\n - Wall position\n - Wall rotating\n - Corresponding pupil frame\n - PI trigger count"
                # "Todo: Should be programmatically started before acquisition trigger"
                n127 = property class="DAQmx Channel"("CI.CountEdges.CountReset.ResetCnt"=u32 0) -> (reference out=w225:refnum<k21>, error out=w223:errorcluster)  [unwired: 2 in]
                n128 = call <vilib>:"DAQmx Start Task.vi"("task/channels in"=w225, "error in"=w223) -> ("task out"=w224:refnum<k21>, "error out"=w222:errorcluster)  [unwired: 12 in]
                n129 = while {
                  shift-right: [w255] -> w219
                  shift-left: w218 -> [w254]
                  shift-right: [w247] -> w229
                  shift-left: w224 -> [w252]
                  shift-right: [w230] -> _
                  shift-left: u32 0 -> [w249]
                  tunnel: w222 -> [w244]
                  tunnel: [w242] -> w221
                  i -> [w246]
                  stop <- w256 continue-if-true
                  # "Listen to two/photon and save data on frames"
                  n130 = local read "Stage Position"() -> (w250:dbl)
                  n131 = Increment(x=w246) -> (x+1=w245:i32)
                  n132 = call-poly <vilib>:"DAQmx Read.vi"("task/channels in"=w252, "error in"=w244) -> ("task out"=w247:refnum<k21>, "data"=w230:u32, "error out"=w241:errorcluster)  [unwired: 11 in]
                  n133 = Subtract(x=w249, y=w230) -> (x-y=w248:u32)
                  n134 = Equal To 0?(x=w248) -> (x = 0?=w251:bool)
                  n135 = local read "Pupil Sample No"() -> (w231:i32)
                  n136 = local read "Wall Position"() -> (w235:dbl)
                  n137 = case shown="No Error" w241 {
                    tunnel: [w257 u32 999999 ("millisecond timer value")] -> w238
                    frame No Error {
                      n138 = Tick Count (ms)() -> (millisecond timer value=w257:u32)
                    }
                    frame Error {
                    }
                  }
                  n139 = case shown="False" w251 {
                    tunnel: w250 -> [w263 w266]
                    tunnel: w248 -> [w265 _]
                    tunnel: [w262 w266] -> w237
                    frame False {
                      n140 = local read "Stage Rotation Direction"() -> (w264:bool)
                      n141 = call "CalculateStagePosition.vi"("Stage Position"=w263, "Numeric in"=w265, "Stage Rotation Direction"=w264) -> ("New Stage Position"=w262:dbl)  [unwired: 8 in]
                      n142 = local write "Stage Position"(w262) -> ()
                    }
                    frame True {
                    }
                  }
                  n143 = local read "Stage Moving?"() -> (w239:bool)
                  n144 = local read "Wall Moving?"() -> (w233:bool)
                  n145 = Boolean To (0,1)(Boolean=w239) -> (0, 1=w240:i16)
                  n146 = Boolean To (0,1)(Boolean=w233) -> (0, 1=w234:i16)
                  n147 = To Double Precision Float(number=w240) -> (double precision float=w236:dbl)
                  n148 = To Double Precision Float(number=w234) -> (double precision float=w232:dbl)
                  n149 = Unbundle By Name(w241) -> ("code"=w243:i32)
                  n150 = local read "Log Stage Positions"() -> (w256:bool)
                  n151 = Build Array(w245, w238, w237, w236, w235, w232, w231, w230) -> (w253:dbl[])
                  n152 = case shown="-200284" w243 {
                    tunnel: w241 -> [w259 w261]
                    tunnel: [w259 w260] -> w242
                    frame 0, Default {
                    }
                    frame -200284 {
                      n153 = call <vilib>:"Clear Errors.vi"("error in (no error)"=w261) -> ("error out"=w260:errorcluster)  [unwired: 6 in]
                    }
                  }
                  n154 = Build Array (concatenate)(w254, w253) -> (w255:dbl[][])
                }
                n155 = call <vilib>:"DAQmx Stop Task.vi"("task/channels in"=w229, "error in"=w221) -> ("task out"=w226:refnum<k21>, "error out"=w220:errorcluster)  [unwired: 12 in]
              }
              frame Enabled {
              }
            }
            n156 = feedback-in #1(w215) -> ()
          }
          frame "Logging Error" {
            n157 = call "Display Message to User"() -> ("OK"=w268:bool)  [unwired: 10 in, 1 out]
            n158 = local write item#-1(w268) -> ()
          }
          frame "SteinmeyerV2" {
            # "Array with info per frame\n - Frame no\n - Relative Millisecond count\n - Stage position\n - Stage rotating\n - Wall position\n - Wall rotating\n - Corresponding pupil frame"
            # "START TASK AND CREATE PROPERTY"
            n159 = Tick Count (ms)() -> (millisecond timer value=w278:u32)
            n160 = call <vilib>:"DAQmx Start Task.vi"("task/channels in"=w271) -> ("task out"=w282:refnum<k21>)  [unwired: 13 in, 1 out]
            n161 = while {
              shift-right: [w295] -> w279
              shift-left: dbl[][] [] -> [w294]
              shift-right: [w296] -> _
              shift-left: 0 -> [w297]
              tunnel: w282 -> [w289]
              tunnel: [w288] -> w283
              tunnel: w278 -> [w293]
              tunnel: [w291] -> w274
              stop <- w292 continue-if-true
              # "Listen to two-photon and save data on frames"
              n162 = call-poly <vilib>:"DAQmx Read.vi"("task/channels in"=w289, "timeout"=1000.0) -> ("task out"=w288:refnum<k21>, "error out"=w286:errorcluster)  [unwired: 11 in, 1 out]
              n163 = case shown="True" TRUE {
                selector: TRUE -> [w299 _]
                tunnel: w297 -> [w298 w321]
                tunnel: [w298 w320] -> w296
                tunnel: [w300 w319] -> w295
                tunnel: w294 -> [w300 w318]
                tunnel: w293 -> [_ w317]
                tunnel: [w299 w316] -> w292
                tunnel: [w299 FALSE] -> w291
                tunnel: w286 -> [_ _]
                frame False {
                }
                frame True {
                  n164 = local read "Pupil Sample No"() -> (w303:i32)
                  n165 = local read "Stage Position"() -> (w311:dbl)
                  n166 = local read "Wall Position"() -> (w307:dbl)
                  n167 = local read "Stage Moving?"() -> (w309:bool)
                  n168 = local read "Wall Moving?"() -> (w305:bool)
                  n169 = Tick Count (ms)() -> (millisecond timer value=w302:u32)
                  n170 = Boolean To (0,1)(Boolean=w309) -> (0, 1=w310:i16)
                  n171 = Boolean To (0,1)(Boolean=w305) -> (0, 1=w306:i16)
                  n172 = To Double Precision Float(number=w310) -> (double precision float=w308:dbl)
                  n173 = To Double Precision Float(number=w306) -> (double precision float=w304:dbl)
                  n174 = Subtract(x=w302, y=w317) -> (x-y=w301:u32)
                  n175 = Increment(x=w321) -> (x+1=w320:i32)
                  n176 = local read "Log Stage Positions"() -> (w315:bool)
                  n177 = Build Array(w320, w301, w311, w308, w307, w304, w303) -> (w312:dbl[])
                  n178 = local write item#-1(w320) -> ()
                  n179 = Build Array (concatenate)(w318, w312) -> (w319:dbl[][])
                  n180 = And(x=TRUE, y=w315) -> (x .and. y?=w316:bool)
                }
              }
            }
            n181 = call <vilib>:"DAQmx Stop Task.vi"("task/channels in"=w283) -> ("task out"=w272:refnum<k21>)  [unwired: 13 in, 1 out]
            n182 = local read "RecordingFolder"() -> (w280:path)
            n183 = call "SaveArrayToTxt.vi"("Input array"=w279, "Filename"="-arena_positions", "File path"=w280) -> ()  [unwired: 1 in, 1 out]
            n184 = Select(t=StageLoggingStates."Logging Error", s=w274, f=StageLoggingStates."Idle") -> (s? t:f=w277:T15)
          }
        }
        n185 = local read "Exit Program"() -> (w122:bool)
      }
    }
    frame Enabled {
    }
  }
  n186 = while {
    shift-right: [w322] -> _
    shift-left: w13 -> [w324]
    stop <- w323 stop-if-true
    # "Main Program Loop. This Loop Runs Training Protocols etc."
    n187 = case shown="\"Calibrate Water Valve\"" w324 {
      tunnel: [FALSE FALSE FALSE FALSE FALSE FALSE FALSE FALSE FALSE FALSE FALSE FALSE FALSE FALSE FALSE FALSE FALSE TRUE FALSE] -> w323
      tunnel: [MainProgramStates."Load Modules" w376 w438 MainProgramStates."Idle" ("Main Program States") w472 w659 w771 w796 w1033 w1081 w1113 w1165 w1217 MainProgramStates."End Recording" MainProgramStates."Reset Session Data" ("Main Program States") MainProgramStates."Idle" ("Main Program States") MainProgramStates."Trial Initialization" ("Main Program States") MainProgramStates."Quit Main Program" ("Main Program States") MainProgramStates."Idle" ("Main Program States")] -> w322
      frame "Init Main Program" {
        # "Set up DAQ channel for sending a trigger signal to SciScan"
        # "Set up DAQ channel for sending start/stop signal to SciScan"
        n188 = disable-structure shown="Disabled" {
          frame Disabled {
            n189 = local write "NRewards"(0 ("NRewards")) -> ()
          }
          frame Enabled {
          }
        }
        n190 = Tick Count (ms)() -> (millisecond timer value=→"Last Count":u32)
        n191 = property on="Current Protocol" class="Enum (strict)"("Visible"=FALSE) -> ()  [unwired: 2 in, 2 out]
        n192 = property on="Trial State" class="DigNum (strict)"("Visible"=FALSE) -> ()  [unwired: 2 in, 2 out]
        n193 = property on="Trial Counter" class="DigNum (strict)"("Visible"=FALSE) -> ()  [unwired: 2 in, 2 out]
        n194 = property on="NDropsCalibration" class="DigNum (strict)"("Visible"=FALSE) -> ()  [unwired: 2 in, 2 out]
        n195 = property on="mlPerDrop" class="DigNum (strict)"("Visible"=TRUE) -> ()  [unwired: 2 in, 2 out]
        n196 = local write "Start Protocol"(FALSE ("Start Protocol")) -> ()
        n197 = property on="Start Protocol" class="Bool (strict)"("DisabledEnum"=T22."Disabled and Grayed Out" ("Disabled")) -> ()  [unwired: 2 in, 2 out]
        n198 = call-poly <vilib>:"DAQmx Create Virtual Channel.vi"("lines"="SciScan Start/Stop") -> ("task out"=w332:refnum<k21>)  [unwired: 13 in, 1 out]
        n199 = call-poly <vilib>:"DAQmx Create Virtual Channel.vi"("lines"="Two-Photon trigger line") -> ("task out"=→"2P TriggerLine":refnum<k21>)  [unwired: 13 in, 1 out]
        n200 = call <vilib>:"DAQmx Start Task.vi"("task/channels in"=w332) -> ("task out"=w330:refnum<k21>)  [unwired: 13 in, 1 out]
        n201 = property on="Trigger microscope" class="Bool (strict)"("Visible"=FALSE) -> ()  [unwired: 2 in, 2 out]
        n202 = call-poly <vilib>:"DAQmx Write.vi"("task/channels in"=w330, "data"=FALSE) -> ("task out"=w329:refnum<k21>)  [unwired: 11 in, 2 out]
        n203 = property on="Abort Protocol" class="Bool (strict)"("DisabledEnum"=T22."Enabled" ("Disabled")) -> ()  [unwired: 2 in, 2 out]
        n204 = property on="2P TriggerLine" class="DAQmxName (strict)"("Visible"=FALSE) -> ()  [unwired: 2 in, 2 out]
        n205 = call <vilib>:"DAQmx Stop Task.vi"("task/channels in"=w329) -> ("task out"=→"SciScan RecordSignal":refnum<k21>)  [unwired: 13 in, 1 out]
        n206 = property on="SciScan RecordSignal" class="DAQmxName (strict)"("Visible"=FALSE) -> ()  [unwired: 2 in, 2 out]
        n207 = property on="Miss" class="Bool (strict)"("Visible"=FALSE) -> ()  [unwired: 2 in, 2 out]
        n208 = property on="Hit" class="Bool (strict)"("Visible"=FALSE) -> ()  [unwired: 2 in, 2 out]
        n209 = property on="nCorrect" class="DigNum (strict)"("Visible"=FALSE) -> ()  [unwired: 2 in, 2 out]
        n210 = property on="tmpNCorrect" class="DigNum (strict)"("Visible"=FALSE) -> ()  [unwired: 2 in, 2 out]
        n211 = property on="Correct?" class="Bool (strict)"("Visible"=FALSE) -> ()  [unwired: 2 in, 2 out]
        n212 = property on="False Alarm" class="Bool (strict)"("Visible"=FALSE) -> ()  [unwired: 2 in, 2 out]
        n213 = property on="Correct Rejection" class="Bool (strict)"("Visible"=FALSE) -> ()  [unwired: 2 in, 2 out]
        n214 = control-ref of="Last Calibration Date"() -> (w347:refnum<vi>)
        n215 = control-ref of="Valve opening time (last calibration) (ms)"() -> (w348:refnum<vi>)
        n216 = control-ref of="mlPerDrop"() -> (w364:refnum<vi>)
        n217 = property on="tdms file performance" class="Ref (strict)"("Visible"=FALSE) -> ()  [unwired: 2 in, 2 out]
        n218 = property on="Lights On" class="Bool (strict)"("Val(Sgnl)"=TRUE ("Value (Signaling)")) -> ()  [unwired: 2 in, 2 out]
        n219 = Build Array(w364, w348, w347) -> (w362:refnum<vi>[])
        "Saved Values" <- w362
        n220 = property on="Saved Values" class="Arr (strict)"("Visible"=FALSE) -> ()  [unwired: 2 in, 2 out]
        n221 = call "Read and Write Controls to Automatic Config File.vi"("Action"=RWC_Actions."Read", "Control References"=w362) -> ("error out"=w339:errorcluster)  [unwired: 9 in]
        n222 = disable-structure shown="Disabled" {
          disable-tunnel: w339 -> [w371 _]
          frame Disabled {
            n223 = case shown="No Error" w371 {
              frame No Error {
                n224 = local read "Valve opening time (last calibration) (ms)"() -> (w372:u32)
                n225 = local write "Valve opening time (ms)"(w372) -> ()
              }
              frame Error {
              }
            }
          }
          frame Enabled {
          }
        }
        "Trial Counter" <- 0 ("Trial Counter")
        "NDropsCalibration" <- 100 ("NDropsCalibration")
        "Hit" <- FALSE ("Hit")
        "False Alarm" <- FALSE ("False Alarm")
        "Miss" <- FALSE ("Miss")
        "Correct Rejection" <- FALSE ("Correct Rejection")
        "Trial State" <- 0 ("Trial State")
        "Correct?" <- FALSE ("Correct?")
      }
      frame "Idle", Default {
        n226 = event shown="[3] \"Start Protocol\": Mouse Down" {
          selector: _ -> [_ _ _ _ _]
          dyn-events: _ -> [_ _ _ _ _]
          timeout: 30 -> [_ _ _ _ _]
          tunnel: [MainProgramStates."Idle" ("Main Program States") MainProgramStates."End Training Protocol" ("Main Program States") MainProgramStates."Calibrate Water Valve" ("Main Program States") w408 MainProgramStates."Idle" ("Main Program States")] -> w374
          event Timeout {
            n227 = event-data() -> ()  [unwired: 1 in, 3 out]
            n228 = local read "Last Count"() -> (w380:u32)
            n229 = local read "Give Water 2"() -> (w386:bool)
            n230 = Tick Count (ms)() -> (millisecond timer value=w381:u32)
            n231 = disable-structure shown="Disabled" {
              frame Disabled {
                n232 = local read "Stage Position"() -> (w397:dbl)
                n233 = In Range and Coerce(upper limit=1.0, x=w397, lower limit=-1.0) -> (In Range?=w394:bool)  [unwired: 1 out]
                n234 = Not(x=w394) -> (.not. x?=w393:bool)
                n235 = case shown="True" w393 {
                  frame False {
                  }
                  frame True {
                    # "Move Home"
                    n236 = call "SMMoveAbsolute.vi"() -> ()  [unwired: 12 in]
                  }
                }
              }
              frame Enabled {
              }
            }
            n237 = local read "Mouse Entered"() -> (w387:bool)
            n238 = Subtract(x=w381, y=w380) -> (x-y=w384:u32)
            n239 = Greater?(x=w384, y=u32 10000) -> (0:w382:bool)
            n240 = And(x=w382, y=w386) -> (x .and. y?=w385:bool)
            n241 = case shown="True" w385 {
              tunnel: w381 -> [_ w390]
              frame False {
              }
              frame True {
                n242 = property on="Give Water" class="Bool (strict)"("Val(Sgnl)"=TRUE ("Value (Signaling)")) -> ()  [unwired: 2 in, 2 out]
                n243 = local write "Last Count"(w390) -> ()
              }
            }
            n244 = case shown="False" w387 {
              frame False {
                n245 = property on="Start Protocol" class="Bool (strict)"("DisabledEnum"=T22."Disabled and Grayed Out" ("Disabled")) -> ()  [unwired: 2 in, 2 out]
              }
              frame True {
                n246 = property on="Start Protocol" class="Bool (strict)"("DisabledEnum"=T22."Enabled" ("Disabled")) -> ()  [unwired: 2 in, 2 out]
              }
            }
          }
          event "Save Trial Data": Value Change {
            # "todo: write metadata to this file"
            n247 = event-data() -> ()  [unwired: 1 in, 6 out]
            n248 = local read "RecordingFolder"() -> (w400:path)
            n249 = local read "SessionID"() -> (w399:string)
            n250 = Concatenate Strings(w399, "-training_results.tdms" ("Data Type")) -> (w402:string)
            n251 = Build Path(base path=w400, name or relative path=w402) -> (appended path=w401:path)
            n252 = TDMS Open(10:T24."open or create" ("operation (0:open)"), 11:w401) -> (3:w398:refnum<k34>)  [unwired: 5 in, 1 out]
            n253 = local write "tdms file performance"(w398) -> ()
          }
          event "Calibrate Valve": Mouse Down {
            n254 = event-data() -> ()  [unwired: 1 in, 8 out]
          }
          event "Start Protocol": Mouse Down {
            # "Maybe handle different protocols differently??"
            n255 = event-data() -> ()  [unwired: 1 in, 8 out]
            n256 = case shown="True" TRUE {
              tunnel: [MainProgramStates."Idle" ("Main Program States") w420] -> w408
              frame False {
                n257 = call <vilib>:"General Error Handler.vi"("[user-defined codes]"=i32[] [5001], "[user-defined descriptions]"=string[] ["You forgot to indicate that the mouse is put into the arena"], "error in (no error)"=errorcluster {"status"=TRUE, "code"=5001, "source"="FrontPanel.vi"}) -> ("error?"=w409:bool)  [unwired: 8 in, 4 out]
                n258 = case shown="True" w409 {
                  frame False {
                  }
                  frame True {
                    n259 = local write "Start Protocol"(FALSE ("Start Protocol")) -> ()
                  }
                }
              }
              frame True {
                n260 = local read "Session Checklist"() -> (w418:T2)
                n261 = property on="Reset" class="Bool (strict)"("Val(Sgnl)"=TRUE ("Value (Signaling)")) -> ()  [unwired: 2 in, 2 out]
                n262 = call "checklist_popup.vi"("Session Checklist In"=w418) -> ("Session Checklist Out"=w416:T2)  [unwired: 10 in]
                n263 = Cluster To Array(cluster=w416) -> (array=w417:bool[])
                n264 = local write "Session Checklist"(w416) -> ()
                n265 = And Array Elements(Boolean array=w417) -> (logical AND=w415:bool)
                n266 = local write "Start Protocol"(w415) -> ()
                n267 = Select(t=MainProgramStates."Start Recording" ("Main Program States"), s=w415, f=MainProgramStates."Idle" ("Main Program States")) -> (s? t:f=w420:T18)
              }
            }
          }
          event "Open Checklist": Value Change {
            n268 = event-data() -> ("NewVal"=w424:bool)  [unwired: 1 in, 5 out]
            n269 = case shown="True" w424 {
              selector: w424 -> [w426 _]
              tunnel: [w426 FALSE] -> w423
              frame False {
              }
              frame True {
                n270 = local read "Session Checklist"() -> (w429:T2)
                n271 = call "checklist_popup.vi"("Session Checklist In"=w429) -> ("Session Checklist Out"=w428:T2)  [unwired: 10 in]
                n272 = local write "Session Checklist"(w428) -> ()
              }
            }
            n273 = local write "Open Checklist"(w423) -> ()
          }
        }
        n274 = local read "Exit Program"() -> (w378:bool)
        n275 = Select(t=MainProgramStates."Quit Main Program" ("Main Program States"), s=w378, f=w374) -> (s? t:f=w376:T18)
      }
      frame "Calibrate Water Valve" {
        n276 = property on="Progress %" class="Slide (strict)"("Visible"=TRUE) -> ()  [unwired: 2 in, 2 out]
        n277 = local read "Valve opening time (ms)"() -> (w433:u32)
        n278 = for {
          N: "Number of drops to release" -> [w441]
          tunnel: [w447] -> w435
          tunnel: w433 -> [w445]
          tunnel: [w441] -> w431
          i -> [w442]
          stop <- w448 stop-if-true
          n279 = flat-sequence {
            tunnel: [w449] -> w446
            tunnel: w445 -> [w449]
            tunnel: w446 -> [w453]
            frame #0 {
              n280 = property on="Give Water" class="Bool (strict)"("Val(Sgnl)"=TRUE ("Value (Signaling)")) -> ()  [unwired: 2 in, 2 out]
            }
            frame #1 {
              n281 = Add(x=w453, y=u32 200) -> (x+y=w452:u32)
              n282 = property on="Give Water" class="Bool (strict)"("Val(Sgnl)"=FALSE ("Value (Signaling)")) -> ()  [unwired: 2 in, 2 out]
              n283 = Wait (ms)(milliseconds to wait=w452) -> ()  [unwired: 1 out]
            }
          }
          n284 = Increment(x=w442) -> (x+1=w447:i32)
          n285 = Equal To 0?(x=w442) -> (x = 0?=w443:bool)
          n286 = call "Incrementer.vi"("N"=w441, "reset"=w443) -> ("Count"=→"Progress %":i32)  [unwired: 13 in]
          n287 = local read "Exit Program"() -> (w448:bool)
        }
        n288 = Equal?(x=w431, y=w435) -> (x = y?=w434:bool)
        n289 = case shown="True" w434 {
          tunnel: w433 -> [_ w455]
          tunnel: w431 -> [_ w463]
          frame False {
          }
          frame True {
            n290 = call "Prompt User for Input"() -> ("milliliters"=w460:dbl)  [unwired: 17 in, 2 out]
            n291 = Get Date/Time In Seconds() -> (seconds since 1Jan1904=w464:timestamp)
            n292 = local write "Valve opening time (last calibration) (ms)"(w455) -> ()
            n293 = To Double Precision Float(number=w463) -> (double precision float=w462:dbl)
            n294 = local write "Last Calibration Date"(w464) -> ()
            n295 = Reciprocal(x=w462) -> (1/x=w461:dbl)
            n296 = Multiply(x=w461, y=w460) -> (x*y=w458:dbl)
            n297 = To Double Precision Float(number=w455) -> (double precision float=w456:dbl)
            n298 = local write "mlPerDrop"(w458) -> ()
            n299 = Divide(x=w458, y=w456) -> (x/y=w457:dbl)
            n300 = property on="Progress %" class="Slide (strict)"("Visible"=FALSE) -> ()  [unwired: 2 in, 2 out]
            n301 = local write "mL Per Ms"(w457) -> ()
          }
        }
        n302 = local read "Exit Program"() -> (w437:bool)
        n303 = Select(t=MainProgramStates."Quit Main Program" ("Main Program States"), s=w437, f=MainProgramStates."Idle" ("Main Program States")) -> (s? t:f=w438:T18)
      }
      frame "Reset Parameters" {
        # "This is currently not used, but could be used before recording starts to reset all parameters."
        n304 = disable-structure shown="Disabled" {
          frame Disabled {
            n305 = flat-sequence {
              frame #0 {
                n306 = invoke on="Mouse Performance" class="Arr (strict)" method="Reinit To Default"() -> ()  [unwired: 3 in, 3 out]
              }
              frame #1 {
                n307 = local read "Mouse Performance"() -> (w470:i16[][])
                n308 = invoke on="Trial Performance" class="WFChart (strict)" method="Reinit To Default"() -> ()  [unwired: 3 in, 3 out]
                n309 = Index Array(array=w470, index (col)=1 ("disabled index (col)")) -> (element=w469:i16[])  [unwired: 1 in]
                n310 = local write "Trial Outcomes"(w469) -> ()
                n311 = property on="Trial Performance" class="WFChart (strict)"("History Data"=dbl[] []) -> ()  [unwired: 2 in, 2 out]
              }
            }
          }
          frame Enabled {
          }
        }
      }
      frame "Start Recording" {
        # "Start SciScan recording and initialize and start data acquisition from lickport"
        n312 = stacked-sequence {
          frame #0 {
            # "Set the next state of lick port recording state machine"
            # "Create Recording Folders"
            n313 = Get Date/Time In Seconds() -> (seconds since 1Jan1904=w492:timestamp)
            n314 = Format Date/Time String(time format string (%c)="%Y_%m_%d", seconds (now)=w492) -> (date/time string=w490:string)  [unwired: 1 in]
            n315 = local read "Mouse Number"() -> (w498:i32)
            n316 = local read "SessionID"() -> (w497:string)
            n317 = Build Path(base path="Data Storage Folder", name or relative path=w490) -> (appended path=w495:path)
            n318 = Build Path(base path=path "C:/Users/Eivind/Google Drive/Lab/Eivind Hennestad/LabviewData/PassiveRotationTask" ("GoogleDrive"), name or relative path=w490) -> (appended path=w491:path)
            n319 = call "MakeFolderIfNeed.vi"("folder path"=w495) -> ("dup folder path"=w494:path)  [unwired: 10 in]
            n320 = call "MakeFolderIfNeed.vi"("folder path"=w491) -> ("dup folder path"=w489:path)  [unwired: 10 in]
            n321 = call "CreateRecordingFolder.vi"("Data folder"=w494, "mouseNumber"=w498, "sessionID"=w497, "Google Drive"=FALSE) -> ("Recording Path"=w476:path)  [unwired: 1 in]
            "RecordingFolder" <- w476
            n322 = call "CreateRecordingFolder.vi"("Data folder"=w489, "mouseNumber"=w498, "sessionID"=w497, "Google Drive"=TRUE) -> ("Recording Path"=→"GoogleDriveFolder":path)  [unwired: 1 in]
            n323 = global write "GlobalVariables.vi" "Recording Folder"(w476) -> ()
            n324 = local read "Day"() -> (w485:u16)
            n325 = Format Into String(format string="-%02d", initial string="_DAY", w485) -> (resulting string=w486:string)  [unwired: 1 in, 1 out]
            n326 = local read "Daily Summary Path"() -> (w478:path)
            n327 = local read "SessionID"() -> (w482:string)
            n328 = Concatenate Strings("training-summary_" ("string"), w482, w486, ".png" ("string")) -> (w481:string)
            n329 = local write "Leave Acquisition Run State"(DataAquisitionStates."Start Data Logging") -> ()
            n330 = Build Path(base path=w478, name or relative path=w481) -> (appended path=→"ImageSummaryPath":path)
            n331 = property on="ImageSummaryPath" class="Path"("Visible"=FALSE) -> ()  [unwired: 2 in, 2 out]
          }
          frame #1 {
            # "create string array for data being recorded"
            n332 = local read "Security Camera Connected"() -> (w528:bool)
            n333 = local read "Pupil Camera Connected"() -> (w525:bool)
            n334 = local read "Lick Port Connected"() -> (w521:bool)
            n335 = local read "Two Photon Connected"() -> (w520:bool)
            n336 = case shown="True" w528 {
              tunnel: string[] [] -> [w549 w552]
              tunnel: [w549 w550] -> w526
              frame False {
              }
              frame True {
                n337 = Build Array (concatenate)(w552, "Security Video") -> (w550:string[])
              }
            }
            n338 = case shown="True" w525 {
              tunnel: [w545 w547] -> w524
              tunnel: w526 -> [w545 w546]
              frame False {
              }
              frame True {
                n339 = Build Array (concatenate)(w546, "Pupil Video") -> (w547:string[])
              }
            }
            n340 = case shown="True" w521 {
              tunnel: [w541 w543] -> w523
              tunnel: w524 -> [w541 w542]
              frame False {
              }
              frame True {
                n341 = Build Array (concatenate)(w542, "Lick Port") -> (w543:string[])
              }
            }
            n342 = case shown="True" w520 {
              tunnel: [w537 w539] -> w522
              tunnel: w523 -> [w537 w538]
              frame False {
              }
              frame True {
                n343 = Build Array (concatenate)(w538, "Two Photon Recording") -> (w539:string[])
              }
            }
            n344 = local read "Cropped Image"() -> (w511:T1)
            n345 = local read "Stage connected"() -> (w519:bool)
            n346 = property on="Select Rotation Stage" class="Enum (strict)"() -> ("RingText.Text"=w517:string)  [unwired: 2 in, 2 out]
            n347 = call "IMAQ GetImageSize"("Image"=w511) -> ("Y Resolution"=w512:i32, "X Resolution"=w510:i32)  [unwired: 3 in, 1 out]
            n348 = case shown="True" w519 {
              tunnel: [w533 w535] -> w504
              tunnel: w522 -> [w533 w534]
              frame False {
              }
              frame True {
                n349 = Build Array (concatenate)(w534, "Stage Positions") -> (w535:string[])
              }
            }
            n350 = local read "Acquisition Frame Rate"() -> (w513:dbl)
            n351 = Build Array(w510, w512) -> (w509:i32[])
            n352 = property on="Select Microscope" class="Enum (strict)"() -> ("RingText.Text"=w516:string)  [unwired: 2 in, 2 out]
            n353 = local read "Wall connected"() -> (w505:bool)
            n354 = local read "dataInfo"() -> (w518:T5)
            n355 = Build Array(624, 480 ("element")) -> (w506:i32[])
            n356 = case shown="True" w505 {
              tunnel: [w529 w531] -> w503
              tunnel: w504 -> [w529 w530]
              frame False {
              }
              frame True {
                n357 = Build Array (concatenate)(w530, "Wall Positions") -> (w531:string[])
              }
            }
            n358 = Bundle By Name(cluster=w518, "Recorded Data"=w503, "Rotation Stage"=w517, "Microscope"=w516, "Framerate Security Camera"=25.0, "Framerate Pupil Camera"=w513, "Image Size Security Camera"=w506, "Image Size Pupil Camera"=w509) -> (w515:T5)
            n359 = local write "dataInfo"(w515) -> ()
          }
          frame #2 {
            # "todo: write metadata to this file"
            # "Create Fileref for Security Video File and data streaming file (TDMS)"
            n360 = local read "RecordingFolder"() -> (w555:path)
            n361 = local read "SessionID"() -> (w554:string)
            n362 = disable-structure shown="Disabled" {
              disable-tunnel: w555 -> [w563 _]
              disable-tunnel: w554 -> [w562 _]
              frame Disabled {
                n363 = local read "Save Security Video As..."() -> (w561:enum16{"BIN", "AVI"})
                n364 = local read "Security Camera Connected"() -> (w564:bool)
                n365 = case shown="True" w564 {
                  tunnel: w563 -> [_ w568]
                  tunnel: w562 -> [_ w567]
                  tunnel: w561 -> [_ w566]
                  frame False {
                  }
                  frame True {
                    n366 = local read "Mouse mask"() -> (w570:T1)
                    n367 = local read "File Path for Mouse Mask"() -> (w569:path)
                    n368 = case shown="\"AVI\"" w566 {
                      tunnel: w568 -> [w575 w583]
                      tunnel: w567 -> [w574 w582]
                      tunnel: "-security_video" ("string") -> [w573 w580]
                      frame "BIN", Default {
                        n369 = Concatenate Strings(w574, w573, ".raw" ("string")) -> (w571:string)
                        n370 = Build Path(base path=w575, name or relative path=w571) -> (appended path=w576:path)
                        n371 = Open/Create/Replace File(file path (use dialog)=w576, operation (0:open)=T25."create", access (0:read/write)=enum16{"read/write", "read-only", "write-only"}."write-only") -> (refnum out=w577:refnum<file>)  [unwired: 3 in, 2 out]
                        n372 = local write "BIN Refnum - Body"(w577) -> ()
                      }
                      frame "AVI" {
                        n373 = call "CreateAviRef.vi"("sessionID"=w582, "Framerate"=u32 25 ("number"), "Filename prefix"=w580, "Block folder"=w583) -> ("Refnum out"=w581:T8)  [unwired: 7 in]
                        n374 = local write "AVI Refnum - Body"(w581) -> ()
                      }
                    }
                    n375 = call "SaveMouseROI.vi"("BlockFolderPath"=w568, "File Path for Mouse Mask"=w569, "sessionID"=w567, "MouseRoi Refnum in"=w570) -> ()  [unwired: 8 in]
                  }
                }
              }
              frame Enabled {
              }
            }
            n376 = Concatenate Strings(w554, "-training_results.tdms" ("Data Type")) -> (w557:string)
            n377 = Build Path(base path=w555, name or relative path=w557) -> (appended path=w556:path)
            n378 = TDMS Open(10:T24."open or create" ("operation (0:open)"), 11:w556) -> (3:→"tdms file performance":refnum<k34>)  [unwired: 5 in, 1 out]
            n379 = global write "GlobalVariables.vi" "prepare recording"(TRUE ("prepare recording")) -> ()
          }
          frame #3 {
            # "todo: write metadata to this file"
            n380 = local read "RecordingFolder"() -> (w586:path)
            n381 = local read "SessionID"() -> (w585:string)
            n382 = Concatenate Strings(w585, "-trial_data.tdms" ("Data Type")) -> (w588:string)
            n383 = Build Path(base path=w586, name or relative path=w588) -> (appended path=w587:path)
            n384 = TDMS Open(10:T24."open or create" ("operation (0:open)"), 11:w587) -> (3:→"trial data tdms fileref":refnum<k34>)  [unwired: 5 in, 1 out]
          }
          frame #4 {
            # "Fill out session Info"
            # "Collect metadata"
            n385 = control-ref of="Selected Training Protocol"() -> (w611:refnum<vi>)
            n386 = local read "sessionInfo"() -> (w602:T7)
            n387 = property class="Enum (strict)"(reference=w611) -> ("RingText.Text"=w600:string)  [unwired: 1 in, 2 out]
            n388 = Get Date/Time In Seconds() -> (seconds since 1Jan1904=w605:timestamp)
            n389 = local read "RecordingID"() -> (w610:string)
            n390 = local read "LightsOnSession"() -> (w593:bool)
            n391 = local read "DarkProbes"() -> (w597:bool)
            n392 = Format Date/Time String(time format string (%c)="%d.%m.%Y", seconds (now)=w605) -> (date/time string=w607:string)  [unwired: 1 in]
            n393 = Format Date/Time String(time format string (%c)="%H:%M:%S", seconds (now)=w605) -> (date/time string=w608:string)  [unwired: 1 in]
            n394 = local read "SessionID"() -> (w596:string)
            n395 = local read "Experiment Name"() -> (w598:string)
            n396 = local read "Mouse entered arena"() -> (w603:string)
            n397 = local read "Mouse Number"() -> (w609:i32)
            n398 = local read "Recording No"() -> (w599:i32)
            n399 = local read "Day"() -> (w595:u16)
            n400 = Bundle By Name(cluster=w602, "experimentName"=w598, "sessionID"=w596, "mouseNumber"=w609, "dateOfExperiment"=w607, "sessionStarted"=w608, "mouseEnteredArena"=w603, "recordingID"=w610, "recordingNo"=w599, "sessionProtocol"=w600, "DarkProbes"=w597, "LightsOn"=w593, "nBlocks"=1, "Day"=w595, "wasSessionAborted"=TRUE) -> (w601:T7)
            n401 = local write "sessionInfo"(w601) -> ()
          }
          frame #5 {
            # "Save prerecording metadata"
            n402 = local read "RecordingFolder"() -> (w624:path)
            n403 = local read "GoogleDriveFolder"() -> (w626:path)
            n404 = local read "sessionInfo"() -> (w625:T7)
            n405 = local read "dataInfo"() -> (w622:T5)
            n406 = Flatten To XML(anything=w622) -> (xml string=w621:string)
            n407 = Flatten To XML(anything=w625) -> (xml string=w628:string)
            n408 = Strip Path(path=w624) -> (stripped path=w615:path)  [unwired: 1 out]
            n409 = Strip Path(path=w626) -> (stripped path=w614:path)  [unwired: 1 out]
            n410 = local read "SessionID"() -> (w629:string)
            n411 = local read "SessionID"() -> (w620:string)
            n412 = Concatenate Strings("sessioninfo-" ("string"), w629, ".xml" ("string")) -> (w627:string)
            n413 = Concatenate Strings(w620, "-recording_metadata" ("string"), ".xml" ("string")) -> (w616:string)
            n414 = Build Path(base path=w615, name or relative path=w616) -> (appended path=w613:path)
            n415 = Build Path(base path=w614, name or relative path=w616) -> (appended path=w612:path)
            n416 = Build Path(base path=w615, name or relative path=w627) -> (appended path=w618:path)
            n417 = Build Path(base path=w614, name or relative path=w627) -> (appended path=w617:path)
            n418 = call-poly <vilib>:"Write to XML File.vi"("XML Input"=w621, "XML File Path"=w612) -> ()  [unwired: 7 in, 3 out]
            n419 = call-poly <vilib>:"Write to XML File.vi"("XML Input"=w628, "XML File Path"=w617) -> ()  [unwired: 7 in, 3 out]
            n420 = call-poly <vilib>:"Write to XML File.vi"("XML Input"=w621, "XML File Path"=w613) -> ()  [unwired: 7 in, 3 out]
            n421 = call-poly <vilib>:"Write to XML File.vi"("XML Input"=w628, "XML File Path"=w618) -> ()  [unwired: 7 in, 3 out]
          }
          frame #6 {
            # "Prepare SciScan"
            n422 = local read "Two Photon Connected"() -> (w632:bool)
            n423 = case shown="True" w632 {
              frame False {
              }
              frame True {
                n424 = local read "SciScan RecordSignal"() -> (w634:refnum<k21>)
                n425 = call <vilib>:"DAQmx Start Task.vi"("task/channels in"=w634) -> ("task out"=w635:refnum<k21>)  [unwired: 13 in, 1 out]
                n426 = call-poly <vilib>:"DAQmx Write.vi"("task/channels in"=w635, "data"=TRUE) -> ()  [unwired: 11 in, 3 out]
              }
            }
          }
          frame #7 {
            # "Wait for SciScan to finish preparing"
            n427 = local read "Two Photon Connected"() -> (w636:bool)
            n428 = case shown="True" w636 {
              frame False {
              }
              frame True {
                n429 = Wait (ms)(milliseconds to wait=u32 5000) -> ()  [unwired: 1 out]
              }
            }
          }
          frame #8 {
            # "Start lick detection data logging"
            n430 = Tick Count (ms)() -> (millisecond timer value=→"Recording Start Time":u32)
            n431 = property on="Recording Start Time" class="DigNum (strict)"("Visible"=FALSE) -> ()  [unwired: 2 in, 2 out]
            n432 = local write "Start Data Logging"(TRUE ("Start Data Logging")) -> ()
          }
          frame #9 {
            # "Wait for lick detection data logging to start"
            n433 = while {
              stop <- w642 continue-if-true
              n434 = local read "Start Data Logging"() -> (w642:bool)
              n435 = Wait (ms)(milliseconds to wait=u32 30) -> ()  [unwired: 1 out]
            }
          }
          frame #10 {
            # "This frame and the next is disabled because I am not using a separate loop for logging stage positions"
            # "Start logging stage positions"
            n436 = disable-structure shown="Disabled" {
              frame Disabled {
                n437 = local write "Log Stage Positions"(TRUE ("Log Stage Positions")) -> ()
              }
              frame Enabled {
              }
            }
          }
          frame #11 {
            # "Wait to be sure that logging state is entered before triggering microscope"
            n438 = Wait (ms)(milliseconds to wait=u32 500) -> ()  [unwired: 1 out]
          }
          frame #12 {
            # "Start 2p imaging, pupiltracker and securitycam"
            n439 = local read "Two Photon Connected"() -> (w647:bool)
            n440 = global write "GlobalVariables.vi" "prepare recording"(FALSE ("prepare recording")) -> ()
            n441 = local write "Session Running"(TRUE ("Session Running")) -> ()
            n442 = case shown="True" w647 {
              frame False {
              }
              frame True {
                n443 = local read "2P TriggerLine"() -> (w652:refnum<k21>)
                n444 = call "Trigger2Photon.vi"("Refnum in"=w652) -> ()  [unwired: 9 in, 2 out]
              }
            }
            n445 = local read "Security Camera Connected"() -> (w649:bool)
            n446 = local read "DemoCamera Connected"() -> (w646:bool)
            n447 = local read "Pupil Camera Connected"() -> (w650:bool)
            n448 = case shown="True" w650 {
              frame False {
              }
              frame True {
                w655 = TRUE ("Start / Stop Tracking")
                n449 = local write "Save Pupil Video"(TRUE ("Save Images")) -> ()
                n450 = local write "Track Pupil"(w655) -> ()
                n451 = property on="Track Pupil" class="Bool (strict)"("Val(Sgnl)"=w655) -> ()  [unwired: 2 in, 2 out]
              }
            }
            n452 = case shown="True" w649 {
              frame False {
              }
              frame True {
                n453 = global write "GlobalVariables.vi" "save data"(TRUE ("Save Images")) -> ()
              }
            }
            n454 = case shown="True" w646 {
              frame False {
              }
              frame True {
                n455 = local write "SaveDemoVideo"(TRUE ("Save Images")) -> ()
              }
            }
          }
        }
        n456 = local read "Abort Protocol"() -> (w474:bool)
        n457 = Select(t=MainProgramStates."End Training Protocol", s=w474, f=MainProgramStates."Init Training Protocol" ("Main Program States")) -> (s? t:f=w472:T18)
      }
      frame "Init Training Protocol" {
        # "Todo: Fill out trial data more holistic...."
        n458 = local read "trialData"() -> (w657:T3)
        n459 = flat-sequence {
          tunnel: w657 -> [w664]
          tunnel: [w663] -> w656
          tunnel: w656 -> [w767]
          frame #0 {
            # "Fill out protocol specific fields of trial data"
            n460 = local read "Selected Training Protocol"() -> (w665:T10)
            n461 = case shown="\"Speed Modulation - Constant Distance\", \"Speed Modulation - Dark - Constant Distance\"" w665 {
              selector: w665 -> [_ _ _ _ _ _ _ w697 _ _ _ _ _ _ _ _ _]
              tunnel: w664 -> [w667 w675 w680 w684 w686 w689 w693 w698 w709 w725 w731 w741 w751 w753 w755 w757 w760]
              tunnel: [w666 w674 w679 w684 w686 w688 w693 w698 w709 w724 w730 w740 w751 w753 w755 w757 w760] -> w663
              frame "Prerecording" {
                n462 = Bundle By Name(cluster=w667, "stageSpeed"=0.0 ("Wall Trial Speed"), "stageAcceleration"=0.0 ("Stage Trial Speed")) -> (w666:T3)
              }
              frame "Rotations - Speed 45 deg/s" {
                n463 = Bundle By Name(cluster=w675, "stageSpeed"=45.0 ("Wall Trial Speed"), "stageAcceleration"=200.0 ("Stage Trial Speed")) -> (w674:T3)
                n464 = local write "Reward Mode"(enum16{"Reward on Cue", "Reward on Lick"}."Reward on Cue" ("Reward Mode")) -> ()
                n465 = local write "Response Window (ms)"(u32 2000 ("Response Window (ms)")) -> ()
                n466 = local write "Intertrial interval (s)"(6 ("Intertrial interval (s)")) -> ()
                n467 = local write "Delay (ms)"(500 ("Delay (ms)")) -> ()
                n468 = local write "nTrials"(100 ("nTrials")) -> ()
              }
              frame "Rotations - Speed 90 deg/s" {
                n469 = Bundle By Name(cluster=w680, "stageSpeed"=90.0 ("Wall Trial Speed"), "stageAcceleration"=200.0 ("Stage Trial Speed")) -> (w679:T3)
                n470 = local write "Reward Mode"(enum16{"Reward on Cue", "Reward on Lick"}."Reward on Cue" ("Reward Mode")) -> ()
              }
              frame "PRT Stage - 3Pos - 2Speeds" {
                n471 = local write "Reward Mode"(enum16{"Reward on Cue", "Reward on Lick"}."Reward on Cue" ("Reward Mode")) -> ()
              }
              frame "PRT Wall - 3Pos - 2Speeds" {
                n472 = local write "Reward Mode"(enum16{"Reward on Cue", "Reward on Lick"}."Reward on Cue" ("Reward Mode")) -> ()
              }
              frame "Wall Rotations - Speed 45deg/s" {
                n473 = Bundle By Name(cluster=w689, "wallSpeed"=45.0 ("Wall Trial Speed"), "wallAcceleration"=200.0 ("Stage Trial Speed")) -> (w688:T3)
                n474 = local write "Reward Mode"(enum16{"Reward on Cue", "Reward on Lick"}."Reward on Cue" ("Reward Mode")) -> ()
              }
              frame "Speed Modulation - Constant Duration" {
              }
              frame "Speed Modulation - Constant Distance", "Speed Modulation - Dark - Constant Distance" {
                w700 = 64 ("Number of trials")
                n475 = case shown="\"Speed Modulation - Dark - Constant Distance\"" w697 {
                  frame "Speed Modulation - Dark - Constant Distance" {
                    w703 = FALSE ("Lights On")
                    n476 = local write "LightsOnSession"(w703) -> ()
                    n477 = property on="Lights On" class="Bool (strict)"("Val(Sgnl)"=w703) -> ()  [unwired: 2 in, 2 out]
                  }
                  frame "Speed Modulation - Constant Distance", Default {
                    w704 = TRUE ("Lights On")
                    n478 = local write "LightsOnSession"(w704) -> ()
                    n479 = local write "Lights On"(w704) -> ()
                  }
                }
                n480 = local read "Stage Speed Selection"() -> (w701:dbl[])
                n481 = local write "nTrials"(w700) -> ()
                n482 = local write "Reward Mode"(enum16{"Reward on Cue", "Reward on Lick"}."Reward on Cue" ("Reward Mode")) -> ()
                n483 = call "DealTrialSpeeds.vi"("Speed Selections"=w701, "Number of trials"=w700) -> ("Trial Speeds"=w699:i32[][])  [unwired: 9 in]
                n484 = local write "Trial Speeds"(w699) -> ()
                n485 = local write "Response Window (ms)"(u32 1500 ("Response Window (ms)")) -> ()
                n486 = local write "Intertrial interval (s)"(4 ("Intertrial interval (s)")) -> ()
                n487 = local write "Delay (ms)"(2500 ("Delay (ms)")) -> ()
              }
              frame "Speed Modulation - Wall - Constant Distance" {
                w705 = TRUE ("Lights On")
                w711 = 64 ("Number of trials")
                n488 = disable-structure shown="Disabled" {
                  frame Disabled {
                    n489 = local write "Response Window (ms)"(u32 0 ("Response Window (ms)")) -> ()
                    n490 = local write "Intertrial interval (s)"(1 ("Intertrial interval (s)")) -> ()
                    n491 = local write "Delay (ms)"(0 ("Delay (ms)")) -> ()
                  }
                  frame Enabled {
                  }
                }
                n492 = local read "Stage Speed Selection"() -> (w712:dbl[])
                n493 = local write "nTrials"(w711) -> ()
                n494 = local write "Reward Mode"(enum16{"Reward on Cue", "Reward on Lick"}."Reward on Cue" ("Reward Mode")) -> ()
                n495 = call "DealTrialSpeeds.vi"("Speed Selections"=w712, "Number of trials"=w711) -> ("Trial Speeds"=w710:i32[][])  [unwired: 9 in]
                n496 = local write "Trial Speeds"(w710) -> ()
                n497 = local write "Response Window (ms)"(u32 1500 ("Response Window (ms)")) -> ()
                n498 = local write "Intertrial interval (s)"(4 ("Intertrial interval (s)")) -> ()
                n499 = local write "LightsOnSession"(w705) -> ()
                n500 = local write "Delay (ms)"(2500 ("Delay (ms)")) -> ()
                n501 = local write "Lights On"(w705) -> ()
                n502 = property on="Lights On" class="Bool (strict)"("Val(Sgnl)"=w705) -> ()  [unwired: 2 in, 2 out]
              }
              frame "Start-Stop" {
                w721 = 120 ("nTrials")
                # "Aim: Same acceleration and velocity but different rotation lengths"
                n503 = call "DealTrialDistance.vi"("Number of trials"=w721) -> ("Trial Distance"=→"Trial Distance":i32[][])  [unwired: 10 in]
                n504 = local write "Intertrial interval (s)"(8 ("Intertrial interval (s)")) -> ()
                n505 = Bundle By Name(cluster=w725, "stageSpeed"=45.0 ("Wall Trial Speed"), "stageAcceleration"=800.0 ("Stage Trial Speed")) -> (w724:T3)
                n506 = local write "Delay (ms)"(4000 ("Delay (ms)")) -> ()
                n507 = local write "Reward Mode"(enum16{"Reward on Cue", "Reward on Lick"}."Reward on Cue" ("Reward Mode")) -> ()
                n508 = local write "LightsOnSession"(FALSE ("LightsOnSession")) -> ()
                n509 = local write "nTrials"(w721) -> ()
                n510 = local write "Lights On"(FALSE ("Lights On")) -> ()
              }
              frame "Start-Stop-90" {
                w736 = 128 ("nTrials")
                # "Aim: Same acceleration and velocity but different rotation lengths"
                n511 = call "DealTrialDistance.vi"("Distance Selection"=i32[] [45, 90, 180, 360], "Number of trials"=w736) -> ("Trial Distance"=w728:i32[][])  [unwired: 9 in]
                n512 = local write "Intertrial interval (s)"(8 ("Intertrial interval (s)")) -> ()
                n513 = Bundle By Name(cluster=w731, "stageSpeed"=90.0 ("Wall Trial Speed"), "stageAcceleration"=800.0 ("Stage Trial Speed")) -> (w730:T3)
                n514 = local write "Trial Distance"(w728) -> ()
                n515 = local write "Delay (ms)"(4000 ("Delay (ms)")) -> ()
                n516 = local write "Reward Mode"(enum16{"Reward on Cue", "Reward on Lick"}."Reward on Cue" ("Reward Mode")) -> ()
                n517 = local write "nTrials"(w736) -> ()
                n518 = local write "LightsOnSession"(FALSE ("LightsOnSession")) -> ()
                n519 = local write "Lights On"(FALSE ("Lights On")) -> ()
              }
              frame "4Accelerations" {
                w748 = 128 ("nTrials")
                # "Aim: Vary the acceleration"
                n520 = call "DealTrialSpeeds.vi"("Speed Selections"=i32[] [100, 200, 400, 800] ("Distance Selection"), "Number of trials"=w748) -> ("Trial Speeds"=w742:i32[][])  [unwired: 9 in]
                n521 = local write "Intertrial interval (s)"(8 ("Intertrial interval (s)")) -> ()
                n522 = local write "Trial Speeds"(w742) -> ()
                n523 = Bundle By Name(cluster=w741, "stageSpeed"=90.0 ("Wall Trial Speed")) -> (w740:T3)
                n524 = local write "Delay (ms)"(4000 ("Delay (ms)")) -> ()
                n525 = local write "Reward Mode"(enum16{"Reward on Cue", "Reward on Lick"}."Reward on Cue" ("Reward Mode")) -> ()
                n526 = local write "nTrials"(w748) -> ()
                n527 = local write "LightsOnSession"(FALSE ("LightsOnSession")) -> ()
                n528 = local write "Lights On"(FALSE ("Lights On")) -> ()
              }
              frame "Free Water" {
                n529 = local write "Reward Mode"(enum16{"Reward on Cue", "Reward on Lick"}."Reward on Lick" ("Reward Mode")) -> ()
              }
              frame "Rotations - Random speeds" {
                n530 = local write "Reward Mode"(enum16{"Reward on Cue", "Reward on Lick"}."Reward on Cue" ("Reward Mode")) -> ()
              }
              frame "Rotations - 240deg 60deg/s" {
                n531 = local write "Reward Mode"(enum16{"Reward on Cue", "Reward on Lick"}."Reward on Cue" ("Reward Mode")) -> ()
              }
              frame "Open Arena - Small Steps" {
                n532 = local write "Reward Mode"(enum16{"Reward on Cue", "Reward on Lick"}."Reward on Cue" ("Reward Mode")) -> ()
              }
              frame "Open Arena - Small Steps 2" {
                n533 = local write "Response Window (ms)"(u32 1000 ("Response Window (ms)")) -> ()
                n534 = local write "Intertrial interval (s)"(4 ("Intertrial interval (s)")) -> ()
                n535 = local write "Reward Mode"(enum16{"Reward on Cue", "Reward on Lick"}."Reward on Cue" ("Reward Mode")) -> ()
                n536 = One Button Dialog(message="This protocol has been edited. Make sure you test it before use") -> ()  [unwired: 1 in, 1 out]
              }
            }
          }
          frame #1 {
            # "Fill out general fields of trial data"
            n537 = local read "Lights On"() -> (w766:bool)
            n538 = property on="nTrials" class="DigNum (strict)"() -> ("Value"=w768:i32)  [unwired: 2 in, 2 out]
            n539 = local write "Baseline Period (s)"(30 ("Baseline Period (s)")) -> ()
            n540 = Bundle By Name(cluster=w767, "lightsOn"=w766) -> (w765:T3)
            n541 = property on="nTrials" class="DigNum (strict)"("Val(Sgnl)"=w768) -> ()  [unwired: 2 in, 2 out]
            n542 = local write "trialData"(w765) -> ()
          }
        }
        n543 = local read "Abort Protocol"() -> (w660:bool)
        n544 = Select(t=MainProgramStates."End Training Protocol", s=w660, f=MainProgramStates."Baseline Period") -> (s? t:f=w659:T18)
      }
      frame "Baseline Period" {
        # "\"Baseline\" period"
        n545 = local read "Two Photon Connected"() -> (w770:bool)
        n546 = case shown="True" w770 {
          frame False {
          }
          frame True {
            n547 = local read "Baseline Period (s)"() -> (w775:i32)
            n548 = for {
              N: w775 -> [_]
              stop <- w777 stop-if-true
              n549 = local read "Abort Protocol"() -> (w777:bool)
              n550 = Wait (ms)(milliseconds to wait=u32 1000) -> ()  [unwired: 1 out]
            }
          }
        }
        n551 = local read "Abort Protocol"() -> (w772:bool)
        n552 = Select(t=MainProgramStates."End Training Protocol", s=w772, f=MainProgramStates."Trial Initialization") -> (s? t:f=w771:T18)
      }
      frame "Trial Initialization" {
        n553 = local read "Trial Counter"() -> (w799:i32)
        n554 = local read "Selected Training Protocol"() -> (w794:T10)
        n555 = local write "Pre trial"(TRUE ("Pre trial")) -> ()
        n556 = local write "Intertrial Interval"(FALSE ("Intertrial Interval")) -> ()
        n557 = local read "DarkProbes"() -> (w781:bool)
        n558 = Increment(x=w799) -> (x+1=w779:i32)
        n559 = local write "Trial Counter"(w779) -> ()
        n560 = case shown="True" w781 {
          frame False {
          }
          frame True {
            n561 = Random Number (0-1)() -> (number: 0 to 1=w804:dbl)
            n562 = Greater Or Equal?(x=w804, y=0.5) -> (x >= y?=w800:bool)
            n563 = property on="Lights On" class="Bool (strict)"("Val(Sgnl)"=w800) -> ()  [unwired: 2 in, 2 out]
            n564 = local read "trialData"() -> (w801:T3)
            n565 = Bundle By Name(cluster=w801, "lightsOn"=w800) -> (w802:T3)
            n566 = local write "trialData"(w802) -> ()
          }
        }
        n567 = local read "nTrials"() -> (w783:i32)
        n568 = local write "Trial State"(1 ("Trial State")) -> ()
        n569 = Number To Decimal String(number=w779) -> (decimal integer string=w788:string)  [unwired: 1 in]
        n570 = Number To Decimal String(number=w783) -> (decimal integer string=w786:string)  [unwired: 1 in]
        n571 = Concatenate Strings("Trial " ("string"), w788, "/" ("string"), w786) -> (→"Current trial":string)
        n572 = local read "trialData"() -> (w780:T3)
        n573 = Bundle By Name(cluster=w780, "trialNumber"=w779) -> (w778:T3)
        n574 = local write "trialData"(w778) -> ()
        n575 = local read "Delay (ms)"() -> (w782:i32)
        n576 = case shown="\"Speed Modulation - Constant Distance\", \"Speed Modulation - Dark - Constant Distance\"" w794 {
          tunnel: "Go Trial Probability" -> [w814 w827 w841 w852 _ _ _ _ _ _ _ _ _ _ _]
          tunnel: w779 -> [_ _ _ _ w873 _ w881 w895 _ _ _ _ _ w959 _]
          tunnel: w782 -> [_ _ _ _ _ _ _ _ _ _ _ _ _ _ _]
          frame "Rotations - Speed 45 deg/s", "Rotations - Speed 90 deg/s" {
            # "Select Target Stage Position"
            n577 = local read "Mouse Performance"() -> (w813:i16[][])
            n578 = local read "Stage Position"() -> (w806:dbl)
            n579 = call "DetermineGoNogoTrial.vi"("Go Trial Probability"=w814, "Mouse Performance"=w813) -> ("Go_Nogo"=w810:bool)  [unwired: 1 in]
            n580 = call "DetermineNextPosition.vi"("GoTrial"=w810) -> ("New Stage Position"=w812:i32)  [unwired: 2 in]
            n581 = local write "Go Trial?"(w810) -> ()
            n582 = call "SelectStageTrajectory.vi"("Stage Position Limit"="Stage Position Limit", "New Stage Position"=w812, "Current Stage Position"=w806) -> ("Target Position"=w805:dbl)  [unwired: 8 in]
            n583 = local read "trialData"() -> (w809:T3)
            n584 = Bundle By Name(cluster=w809, "moveStage"=TRUE ("moveWall"), "stageStartPosition"=w806, "stageStopPosition"=w805) -> (w808:T3)
            n585 = local write "trialData"(w808) -> ()
          }
          frame "PRT Stage - 3Pos - 2Speeds" {
            # "Randomly select new position"
            # "Randomly select speed"
            n586 = local read "Mouse Performance"() -> (w826:i16[][])
            n587 = call "DetermineGoNogoTrial.vi"("Go Trial Probability"=w827, "Mouse Performance"=w826) -> ("Go_Nogo"=w824:bool)  [unwired: 1 in]
            n588 = local read "Stage Position"() -> (w818:dbl)
            n589 = local write "Go Trial?"(w824) -> ()
            n590 = call "DetermineNextPosition.vi"("GoTrial"=w824) -> ("New Stage Position"=w825:i32)  [unwired: 2 in]
            n591 = call "RandSelectSpeed.vi"("Array"=dbl[] [45.0, 90.0]) -> ("Numeric"=w816:dbl)  [unwired: 10 in]
            n592 = local read "Stage Position Limit"() -> (w822:i32)
            n593 = call "SelectStageTrajectory.vi"("Stage Position Limit"=w822, "New Stage Position"=w825, "Current Stage Position"=w818) -> ("Target Position"=w817:dbl)  [unwired: 8 in]
            n594 = local read "trialData"() -> (w819:T3)
            n595 = Bundle By Name(cluster=w819, "moveStage"=TRUE ("moveWall"), "stageStartPosition"=w818, "stageStopPosition"=w817, "stageSpeed"=w816, "stageAcceleration"=400.0) -> (w820:T3)
            n596 = local write "trialData"(w820) -> ()
          }
          frame "PRT Wall - 3Pos - 2Speeds" {
            n597 = local read "Mouse Performance"() -> (w840:i16[][])
            n598 = call "DetermineGoNogoTrial.vi"("Go Trial Probability"=w841, "Mouse Performance"=w840) -> ("Go_Nogo"=w835:bool)  [unwired: 1 in]
            n599 = local write "Go Trial?"(w835) -> ()
            n600 = call "DetermineNextPosition.vi"("GoTrial"=w835) -> ("New Stage Position"=w836:i32)  [unwired: 2 in]
            n601 = local read "Wall max rotation"() -> (w834:dbl)
            n602 = local read "Wall Position"() -> (w828:dbl)
            n603 = call "RandSelectSpeed.vi"("Array"=dbl[] [45.0, 90.0]) -> ("Numeric"=w832:dbl)  [unwired: 10 in]
            n604 = call "SelectWallTrajectory.vi"("Wall Position Limit"=w834, "New Wall Position"=w836, "Current Wall Position"=w828) -> ("StepSize"=w830:i32)  [unwired: 8 in]
            n605 = Add(x=w828, y=w830) -> (x+y=w829:dbl)
            n606 = local read "Wall Acceleration (deg2/s)"() -> (w831:dbl)
            n607 = local read "trialData"() -> (w839:T3)
            n608 = Bundle By Name(cluster=w839, "moveWall"=TRUE, "wallStartPosition"=w828, "wallStopPosition"=w829, "wallSpeed"=w832, "wallAcceleration"=w831) -> (w838:T3)
            n609 = local write "trialData"(w838) -> ()
          }
          frame "Wall Rotations - Speed 45deg/s" {
            n610 = local read "Mouse Performance"() -> (w851:i16[][])
            n611 = call "DetermineGoNogoTrial.vi"("Go Trial Probability"=w852, "Mouse Performance"=w851) -> ("Go_Nogo"=w849:bool)  [unwired: 1 in]
            n612 = local write "Go Trial?"(w849) -> ()
            n613 = call "DetermineNextPosition.vi"("GoTrial"=w849) -> ("New Stage Position"=w850:i32)  [unwired: 2 in]
            n614 = local read "Wall max rotation"() -> (w848:dbl)
            n615 = local read "Wall Position"() -> (w842:dbl)
            n616 = call "SelectWallTrajectory.vi"("Wall Position Limit"=w848, "New Wall Position"=w850, "Current Wall Position"=w842) -> ("StepSize"=w843:i32)  [unwired: 8 in]
            n617 = Add(x=w842, y=w843) -> (x+y=w844:dbl)
            n618 = local read "trialData"() -> (w847:T3)
            n619 = Bundle By Name(cluster=w847, "moveWall"=TRUE, "wallStartPosition"=w842, "wallStopPosition"=w844) -> (w846:T3)
            n620 = local write "trialData"(w846) -> ()
          }
          frame "Speed Modulation - Constant Distance", "Speed Modulation - Dark - Constant Distance" {
            # "Add + or - 180 degree to position. \nNegate because the Steinmeyer definition of positive is opposite from mine"
            # "Odd trials CW, Even trials CCW"
            n621 = local read "Trial Speeds"() -> (w870:i32[][])
            n622 = Decrement(x=w873) -> (x-1=w868:i32)
            n623 = Quotient & Remainder(x=w868, y=2) -> (x-y*floor(x/y)=w869:i32, floor(x/y)=w871:i32)
            n624 = Equal To 0?(x=w869) -> (x = 0?=w863:bool)
            n625 = Index Array(array=w870, index (row)=w871, index (col)=w869) -> (element=w867:i32)
            n626 = To Double Precision Float(number=w867) -> (double precision float=w856:dbl)
            n627 = To Long Integer(number=w856) -> (32bit integer=w855:i32)
            n628 = case shown="45, Default" w855 {
              tunnel: [200.0 ("Acceleration") 300.0 ("Acceleration") 400.0 ("Acceleration") 500.0 ("Acceleration")] -> w854
              frame 45, Default {
              }
              frame 90 {
              }
              frame 135 {
              }
              frame 180 {
              }
            }
            n629 = local read "Stage Position"() -> (w859:dbl)
            n630 = Select(t=-180.0 ("Stage step size (deg)"), s=w863, f=180.0 ("Stage step size (deg)")) -> (s? t:f=w860:dbl)
            n631 = Add(x=w859, y=w860) -> (x+y=w858:dbl)
            n632 = Negate(x=w858) -> (-x=w857:dbl)
            n633 = local read "trialData"() -> (w864:T3)
            n634 = Bundle By Name(cluster=w864, "moveStage"=TRUE ("moveWall"), "stageStartPosition"=w859, "stageStopPosition"=w857, "stageSpeed"=w856, "stageAcceleration"=w854) -> (w865:T3)
            n635 = local write "Go Trial?"(TRUE ("Go Trial?")) -> ()
            n636 = local write "trialData"(w865) -> ()
          }
          frame "Speed Modulation - Constant Duration" {
            # "Determine direction (opposite from last or random?)\nDetermine speed (and stepsize) (Randomize)\n\nUse three different speeds 30, 75, 120?\n\nCheck that position wil not exceed +- 720 degrees\n\nSave speed per trial"
          }
          frame "Start-Stop", "Start-Stop-90" {
            # "Add trial distance to startposition.\nNegate because the Steinmeyer definition of positive is opposite from mine"
            # "Odd trials CW, Even trials CCW"
            n637 = local read "Trial Distance"() -> (w880:i32[][])
            n638 = Decrement(x=w881) -> (x-1=w889:i32)
            n639 = Quotient & Remainder(x=w889, y=2) -> (x-y*floor(x/y)=w890:i32, floor(x/y)=w891:i32)
            n640 = Equal To 0?(x=w890) -> ()  [unwired: 1 out]
            n641 = Index Array(array=w880, index (row)=w891, index (col)=w890) -> (element=w888:i32)
            n642 = To Double Precision Float(number=w888) -> (double precision float=w879:dbl)
            n643 = local write "Go Trial?"(TRUE ("Go Trial?")) -> ()
            n644 = local read "Stage Position"() -> (w884:dbl)
            n645 = Add(x=w884, y=w879) -> (x+y=w883:dbl)
            n646 = Negate(x=w883) -> (-x=w882:dbl)
            n647 = local read "trialData"() -> (w885:T3)
            n648 = Bundle By Name(cluster=w885, "moveStage"=TRUE ("moveWall"), "stageStartPosition"=w884, "stageStopPosition"=w882) -> (w886:T3)
            n649 = local write "trialData"(w886) -> ()
          }
          frame "4Accelerations" {
            # "Add + or - 180 degree to position. \nNegate because the Steinmeyer definition of positive is opposite from mine"
            # "Odd trials CW, Even trials CCW"
            n650 = local read "Trial Speeds"() -> (w909:i32[][])
            n651 = Decrement(x=w895) -> (x-1=w907:i32)
            n652 = Quotient & Remainder(x=w907, y=2) -> (x-y*floor(x/y)=w908:i32, floor(x/y)=w910:i32)
            n653 = Equal To 0?(x=w908) -> (x = 0?=w902:bool)
            n654 = Index Array(array=w909, index (row)=w910, index (col)=w908) -> (element=w906:i32)
            n655 = To Double Precision Float(number=w906) -> (double precision float=w894:dbl)
            n656 = local write "Go Trial?"(TRUE ("Go Trial?")) -> ()
            n657 = local read "Stage Position"() -> (w898:dbl)
            n658 = Select(t=-180.0 ("Stage step size (deg)"), s=w902, f=180.0 ("Stage step size (deg)")) -> (s? t:f=w899:dbl)
            n659 = Add(x=w898, y=w899) -> (x+y=w897:dbl)
            n660 = Negate(x=w897) -> (-x=w896:dbl)
            n661 = local read "trialData"() -> (w903:T3)
            n662 = Bundle By Name(cluster=w903, "moveStage"=TRUE ("moveWall"), "stageStartPosition"=w898, "stageStopPosition"=w896, "stageAcceleration"=w894) -> (w904:T3)
            n663 = local write "trialData"(w904) -> ()
          }
          frame "Prerecording" {
            n664 = while {
              stop <- w912 stop-if-true
              n665 = local read "Abort Protocol"() -> (w912:bool)
              n666 = Wait (ms)(milliseconds to wait=u32 50) -> ()  [unwired: 1 out]
            }
          }
          frame "Open Arena - Small Steps" {
            w924 = dbl[] [45.0, 90.0] ("Speed Selection")
            # "Randomly select speed"
            # "Select trajectory and \nget new position"
            # "Randomly select new position"
            n667 = local read "Mouse Performance"() -> (w935:i16[][])
            n668 = Divide(x=5.0, y=12.0) -> (x/y=w923:dbl)
            n669 = call "DetermineGoNogoTrial.vi"("Go Trial Probability"=w923, "Mouse Performance"=w935) -> ("Go_Nogo"=w931:bool)  [unwired: 1 in]
            n670 = call "DetermineNextPosition.vi"("Nogo Positions"=i32[] [0, 180, 210, 240, 270, 300, 330] ("Go Positions"), "GoTrial"=w931, "Go Positions"=i32[] [30, 60, 90, 120, 150]) -> ("New Stage Position"=w932:i32)
            n671 = local write "Go Trial?"(w931) -> ()
            n672 = local read "Stage Position Limit"() -> (w930:i32)
            n673 = local read "Stage Position"() -> (w914:dbl)
            n674 = Random Number (0-1)() -> (number: 0 to 1=w929:dbl)
            n675 = call "SelectStageTrajectory.vi"("Stage Position Limit"=w930, "New Stage Position"=w932, "Current Stage Position"=w914) -> ("Target Position"=w915:dbl)  [unwired: 8 in]
            n676 = Array Size(array=w924) -> (size(s)=w925:i32)
            n677 = Multiply(x=w929, y=w925) -> (x*y=w928:dbl)
            n678 = Round Toward -Infinity(1:w928) -> (0:w926:dbl)
            n679 = To Long Integer(number=w926) -> (32bit integer=w927:i32)
            n680 = Index Array(array=w924, index=w927) -> (element=w916:dbl)
            n681 = local read "trialData"() -> (w920:T3)
            n682 = Bundle By Name(cluster=w920, "moveStage"=TRUE ("moveWall"), "stageStartPosition"=w914, "stageStopPosition"=w915, "stageSpeed"=w916, "stageAcceleration"=400.0 ("Acceleration")) -> (w919:T3)
            n683 = local write "trialData"(w919) -> ()
          }
          frame "Rotations - Random speeds" {
            # "Not implemented"
          }
          frame "Rotations - 240deg 60deg/s" {
            # "Not updated - fix before using"
            n684 = disable-structure shown="Disabled" {
              frame Disabled {
                n685 = local read "Stage Position"() -> (w939:dbl)
                n686 = Random Number (0-1)() -> (number: 0 to 1=w944:dbl)
                n687 = Greater Or Equal?(x=w944, y=0.5) -> (x >= y?=w942:bool)
                n688 = Select(t=-240.0, s=w942, f=240.0) -> (s? t:f=w938:dbl)
                n689 = Add(x=w939, y=w938) -> (x+y=w937:dbl)
                n690 = call "SelectStageTrajectory2.vi"("Stage Position Limit"=1080, "Stage Speed"=60.0, "New Stage Position"=w937, "Stage Position"=w939) -> ()  [unwired: 8 in]
              }
              frame Enabled {
              }
            }
          }
          frame "Free Water" {
            n691 = local write "AllowReward"(TRUE ("AllowLick")) -> ()
            n692 = property on="Reward Green Light" class="Bool (strict)"("Val(Sgnl)"=TRUE ("Value (Signaling)")) -> ()  [unwired: 2 in, 2 out]
          }
          frame "Speed Modulation - Wall - Constant Distance" {
            # "Added 0.3 as correction 18.08.2020"
            # "Ref page in small notebook on rig computer from 29/11/2019\nThe wall position is inaccurate and it is speed direction dependent"
            # "% Note, this will be opposite for \nspeed-mod mouse rot"
            # "Get speed for current trial"
            # "CCW rotation is positive"
            # "Randomly select wall speed."
            # "Odd trials CCW, Even trials CW"
            n693 = Decrement(x=w959) -> (x-1=w958:i32)
            n694 = Quotient & Remainder(x=w958, y=2) -> (x-y*floor(x/y)=w970:i32, floor(x/y)=w972:i32)
            n695 = Not Equal To 0?(x=w970) -> (x != 0?=w951:bool)
            n696 = local read "Trial Speeds"() -> (w971:i32[][])
            n697 = Not(x=w951) -> (.not. x?=w952:bool)
            n698 = case shown="False" w951 {
              selector: w951 -> [w975 w977]
              tunnel: [w975 w977] -> w954
              tunnel: [w974 w976] -> w953
              frame False {
                w974 = 0.0
                n699 = local write "Wall Position"(w974) -> ()
              }
              frame True {
                n700 = local read "Wall Position"() -> (w976:dbl)
              }
            }
            n701 = Index Array(array=w971, index (row)=w972, index (col)=w970) -> (element=w969:i32)
            n702 = To Double Precision Float(number=w969) -> (double precision float=w961:dbl)
            n703 = global write "GlobalVariables.vi" "Wall Position Reset Global"(w952) -> ()
            n704 = To Long Integer(number=w961) -> (32bit integer=w962:i32)
            n705 = case shown="45, Default" w962 {
              tunnel: [200.0 ("Acceleration") 300.0 ("Acceleration") 400.0 ("Acceleration") 500.0 ("Acceleration")] -> w960
              tunnel: [0.66 1.07 1.2 1.4] -> w949
              frame 45, Default {
              }
              frame 90 {
              }
              frame 135 {
              }
              frame 180 {
              }
            }
            n706 = Subtract(x=w949, y=0.7) -> (x-y=w948:dbl)
            n707 = Add(x=w948, y=-180.0 ("t")) -> (x+y=w955:dbl)
            n708 = Select(t=w955, s=w954, f=180.0) -> (s? t:f=w963:dbl)
            n709 = Add(x=w953, y=w963) -> (x+y=w964:dbl)
            n710 = local read "trialData"() -> (w968:T3)
            n711 = Bundle By Name(cluster=w968, "moveWall"=TRUE, "wallStartPosition"=w953, "wallStopPosition"=w964, "wallSpeed"=w961, "wallAcceleration"=w960) -> (w967:T3)
            n712 = local write "Go Trial?"(TRUE ("Go Trial?")) -> ()
            n713 = local write "trialData"(w967) -> ()
            n714 = disable-structure shown="Disabled" {
              frame Disabled {
                n715 = call "RandSelectSpeed.vi"() -> ()  [unwired: 11 in, 1 out]
              }
              frame Enabled {
              }
            }
          }
          frame "Open Arena - Small Steps 2" {
            w1009 = dbl[] [45.0, 90.0, 135.0] ("Speed Selection")
            # "The previous implementation just sent the displacement to move stage relative"
            # "Please test before using, specifically, \nis it correct to add displacement to current pos"
            n716 = local write "Go Trial?"(TRUE ("Go Trial?")) -> ()
            n717 = Random Number (0-1)() -> (number: 0 to 1=w1008:dbl)
            n718 = local read "Stage Position Limit"() -> (w1000:i32)
            n719 = Random Number (0-1)() -> (number: 0 to 1=w1003:dbl)
            n720 = Multiply(x=w1008, y=6.0) -> (x*y=w1006:dbl)
            n721 = local read "Stage Position"() -> (w1001:dbl)
            n722 = Round Toward +Infinity(x=w1006) -> (ceil(x): smallest int >= x=w1005:dbl)
            n723 = Array Size(array=w1009) -> (size(s)=w1010:i32)
            n724 = Greater?(x=w1003, y=0.5) -> (0:w998:bool)
            n725 = Multiply(x=w1005, y=30.0) -> (x*y=w997:dbl)
            n726 = Random Number (0-1)() -> (number: 0 to 1=w1014:dbl)
            n727 = Negate(x=w1001) -> (-x=w990:dbl)
            n728 = Multiply(x=w1014, y=w1010) -> (x*y=w1013:dbl)
            n729 = case shown="False" w998 {
              tunnel: w997 -> [w1015 w1017]
              tunnel: [w1015 w1016] -> w996
              frame False {
              }
              frame True {
                n730 = Negate(x=w1017) -> (-x=w1016:dbl)
              }
            }
            n731 = call "LimitMovementAmount.vi"("Max rotation"=w1000, "Current position"=w990, "Direction"=w998, "Move amount in"=w997) -> ("Movement allowed"=w999:bool)  [unwired: 6 in, 1 out]
            n732 = Round Toward -Infinity(1:w1013) -> (0:w1011:dbl)
            n733 = To Long Integer(number=w1011) -> (32bit integer=w1012:i32)
            n734 = Index Array(array=w1009, index=w1012) -> (element=w986:dbl)
            n735 = case shown="True" w999 {
              tunnel: w996 -> [w1019 w1020]
              tunnel: [w1018 w1020] -> w989
              frame False {
                n736 = Negate(x=w1019) -> (-x=w1018:dbl)
              }
              frame True {
              }
            }
            n737 = Add(x=w990, y=w989) -> (x+y=w988:dbl)
            n738 = local read "trialData"() -> (w991:T3)
            n739 = Bundle By Name(cluster=w991, "moveStage"=TRUE ("moveWall"), "stageStartPosition"=w990, "stageStopPosition"=w988, "stageSpeed"=w986, "stageAcceleration"=400.0 ("Acceleration")) -> (w992:T3)
            n740 = local write "Delay (ms)"(1000 ("Delay (ms)")) -> ()
            n741 = local write "trialData"(w992) -> ()
          }
        }
        n742 = local read "Abort Protocol"() -> (w795:bool)
        n743 = Select(t=MainProgramStates."End Training Protocol", s=w795, f=MainProgramStates."Move Stage / Wall") -> (s? t:f=w796:T18)
      }
      frame "Move Stage / Wall" {
        # "Wait till stage and/or \nwall stops"
        # "Wait 100 ms to make sure stage has\nstarted to move before proceeding \nto wait for stage/wall to stop"
        n744 = local read "trialData"() -> (w1032:T3)
        n745 = Unbundle By Name(w1032) -> ("moveStage"=w1037:bool, "moveWall"=w1036:bool)
        n746 = case shown="True" w1037 {
          selector: w1037 -> [w1068 w1069]
          tunnel: w1032 -> [_ w1073]
          tunnel: [w1068 w1069] -> w1029
          frame False {
          }
          frame True {
            # "Move Stage to New Absolute Position"
            n747 = Unbundle By Name(w1073) -> ("stageStopPosition"=w1072:dbl, "stageSpeed"=w1071:dbl, "stageAcceleration"=w1070:dbl)
            "stageStopPosition" <- w1072
            "stageAcceleration" <- w1070
            n748 = call "SMMoveAbsolute.vi"("Acceleration"=w1070, "Speed"=w1071, "Displacement"=w1072) -> ()  [unwired: 9 in]
          }
        }
        n749 = case shown="True" w1036 {
          selector: w1036 -> [w1053 w1057]
          tunnel: w1032 -> [_ w1067]
          tunnel: [w1053 w1057] -> w1028
          frame False {
          }
          frame True {
            # "Move Wall to New Absolute Position"
            n750 = local read "StepperController.lvclass"() -> (w1066:refnum<class "StepperController.lvclass">)
            n751 = Unbundle By Name(w1067) -> ("wallStopPosition"=w1065:dbl, "wallStartPosition"=w1064:dbl, "wallSpeed"=w1063:dbl, "wallAcceleration"=w1062:dbl)
            n752 = Subtract(x=w1065, y=w1064) -> (x-y=w1056:dbl)
            n753 = Absolute Value(x=w1056) -> (abs(x)=w1055:dbl)
            n754 = call-dynamic "PrepareRotation.vi"("Rotate amount"=w1055, "Acceleration (deg2/s)"=w1062, "Speed (deg/s)"=w1063, "StepperController in"=w1066) -> ("StepperController out"=w1059:refnum<class "StepperController.lvclass">)  [unwired: 5 in, 2 out]
            n755 = Less Than 0?(x=w1056) -> (x < 0?=w1058:bool)
            n756 = call "Rotate.vi"("Direction"=w1058, "StepperController in"=w1059) -> ("NewPosition"=w1061:dbl, "DidMove"=w1054:bool, "StepperController out"=w1060:refnum<class "StepperController.lvclass">)  [unwired: 5 in, 2 out]
            n757 = local write "StepperController.lvclass"(w1060) -> ()
            n758 = local write "Wall Moving?"(w1054) -> ()
            n759 = local write "Wall Position"(w1061) -> ()
          }
        }
        n760 = Or(x=w1029, y=w1028) -> (x .or. y?=w1030:bool)
        n761 = case shown="True" w1030 {
          selector: w1030 -> [w1046 w1047]
          tunnel: w1029 -> [_ w1048]
          tunnel: [w1046 w1047] -> w1027
          frame False {
          }
          frame True {
            n762 = local write "Stage Moving?"(w1048) -> ()
            n763 = Wait (ms)(milliseconds to wait=u32 100) -> ()  [unwired: 1 out]
          }
        }
        n764 = case shown="True" w1027 {
          tunnel: [FALSE ("Stage Moving?") w1041] -> w1026
          tunnel: [FALSE ("Wall Moving?") w1040] -> w1025
          frame False {
          }
          frame True {
            n765 = while {
              tunnel: [w1044] -> w1041
              stop <- w1044 continue-if-true
              n766 = local read "Stage Moving?"() -> (w1044:bool)
              n767 = Wait (ms)(milliseconds to wait=u32 30) -> ()  [unwired: 1 out]
            }
            n768 = while {
              tunnel: [w1042] -> w1040
              stop <- w1042 continue-if-true
              n769 = local read "Wall Moving?"() -> (w1042:bool)
              n770 = Wait (ms)(milliseconds to wait=u32 30) -> ()  [unwired: 1 out]
            }
          }
        }
        n771 = Not(x=w1026) -> (.not. x?=w1023:bool)
        n772 = Not(x=w1025) -> (.not. x?=w1022:bool)
        n773 = And(x=w1023, y=w1022) -> (x .and. y?=w1024:bool)
        n774 = case shown="True" w1024 {
          tunnel: [FALSE ("Abort Protocol") w1051] -> w1021
          frame False {
          }
          frame True {
            n775 = local read "Abort Protocol"() -> (w1051:bool)
            n776 = Wait (ms)(milliseconds to wait="Delay (ms)") -> ()  [unwired: 1 out]
          }
        }
        n777 = Select(t=MainProgramStates."End Training Protocol", s=w1021, f=MainProgramStates."Cue") -> (s? t:f=w1033:T18)
      }
      frame "Cue" {
        n778 = local write "Cue"(TRUE ("Pre trial")) -> ()
        n779 = local write "Pre trial"(FALSE ("Intertrial Interval")) -> ()
        n780 = local read "Reward Mode"() -> (w1080:enum16{"Reward on Cue", "Reward on Lick"})
        n781 = local write "Trial State"(2 ("Trial State")) -> ()
        n782 = case shown="\"Reward on Cue\", Default" w1080 {
          tunnel: [u32 350 ("milliseconds to wait") u32 200 ("milliseconds to wait")] -> w1076
          tunnel: [w1090 FALSE ("f")] -> w1074
          frame "Reward on Cue", Default {
            n783 = local read "NGoTrials"() -> (w1093:i32)
            n784 = local read "Go Trial?"() -> (w1098:bool)
            n785 = Select(t=1, s=w1098, f=0) -> (s? t:f=w1094:i32)
            n786 = Select(t=TRUE, s=w1098, f=FALSE) -> (s? t:f=w1090:bool)
            n787 = Add(x=w1094, y=w1093) -> (x+y=w1095:i32)
            n788 = local write "AllowReward"(w1090) -> ()
            n789 = local write "NGoTrials"(w1095) -> ()
            n790 = property on="Reward Green Light" class="Bool (strict)"("Val(Sgnl)"=TRUE ("Value (Signaling)")) -> ()  [unwired: 2 in, 2 out]
            n791 = local write "Response Window"(1.0 ("Response Window")) -> ()
          }
          frame "Reward on Lick" {
            n792 = local read "Stage Position"() -> (w1106:dbl)
            n793 = In Range and Coerce(upper limit=5.0, x=w1106, lower limit=-5.0) -> (In Range?=w1103:bool)  [unwired: 1 out]
            n794 = local write "AllowReward"(w1103) -> ()
            n795 = property on="Reward Green Light" class="Bool (strict)"("Val(Sgnl)"=TRUE ("Value (Signaling)")) -> ()  [unwired: 2 in, 2 out]
          }
        }
        n796 = flat-sequence {
          tunnel: w1076 -> [w1085]
          tunnel: w1074 -> [w1087]
          frame #0 {
            n797 = Wait (ms)(milliseconds to wait=w1085) -> ()  [unwired: 1 out]
          }
          frame #1 {
            n798 = And(x="Give water", y=w1087) -> (x .and. y?=w1088:bool)
            n799 = case shown="True" w1088 {
              frame False {
              }
              frame True {
                n800 = property on="Give Water" class="Bool (strict)"("Val(Sgnl)"=TRUE ("Value (Signaling)")) -> ()  [unwired: 2 in, 2 out]
              }
            }
          }
        }
        n801 = local read "Abort Protocol"() -> (w1082:bool)
        n802 = Select(t=MainProgramStates."End Training Protocol", s=w1082, f=MainProgramStates."Response Window") -> (s? t:f=w1081:T18)
      }
      frame "Response Window" {
        n803 = local write "Response Window"(TRUE ("Pre trial")) -> ()
        n804 = local write "Cue"(FALSE ("Intertrial Interval")) -> ()
        n805 = flat-sequence {
          frame #0 {
            n806 = while {
              stop <- w1117 continue-if-true
              n807 = local read "response window is open"() -> (w1117:bool)
              n808 = Wait (ms)(milliseconds to wait=u32 30) -> ()  [unwired: 1 out]
            }
          }
          frame #1 {
            n809 = local read "last response time (ms)"() -> (w1139:dbl)
            n810 = local read "Session Performance"() -> (w1131:i16[][])
            n811 = local read "Mouse Performance"() -> (w1132:i16[][])
            n812 = local read "Trial Counter"() -> (w1143:i32)
            n813 = local read "Hit"() -> (w1135:bool)
            n814 = local read "Correct Rejection"() -> (w1136:bool)
            n815 = local read "Miss"() -> (w1159:bool)
            n816 = local read "False Alarm"() -> (w1158:bool)
            n817 = local read "Go Trial?"() -> (w1144:bool)
            n818 = local read "trialData"() -> (w1125:T3)
            n819 = Unbundle By Name(w1125) -> ("stageSpeed"=w1124:dbl, "wallSpeed"=w1123:dbl, "stageAcceleration"=w1122:dbl, "wallAcceleration"=w1121:dbl)
            n820 = Boolean To (0,1)(Boolean=w1135) -> (0, 1=w1157:i16)
            n821 = Boolean To (0,1)(Boolean=w1136) -> (0, 1=w1156:i16)
            n822 = Boolean To (0,1)(Boolean=w1159) -> (0, 1=w1155:i16)
            n823 = Boolean To (0,1)(Boolean=w1158) -> (0, 1=w1154:i16)
            n824 = To Word Integer(number=w1139) -> (16bit integer=w1138:i16)
            n825 = Multiply(x=w1157, y=i16 4) -> (x*y=w1149:i16)
            n826 = Multiply(x=w1156, y=i16 3) -> (x*y=w1148:i16)
            n827 = Multiply(x=w1155, y=i16 2) -> (x*y=w1147:i16)
            n828 = Multiply(x=w1154, y=i16 1) -> (x*y=w1146:i16)
            n829 = To Word Integer(number=w1122) -> (16bit integer=w1120:i16)
            n830 = To Word Integer(number=w1121) -> (16bit integer=w1119:i16)
            n831 = To Word Integer(number=w1124) -> (16bit integer=w1127:i16)
            n832 = To Word Integer(number=w1123) -> (16bit integer=w1126:i16)
            n833 = Boolean To (0,1)(Boolean=w1144) -> (0, 1=w1133:i16)
            n834 = To Word Integer(number=w1143) -> (16bit integer=w1142:i16)
            n835 = Compound Arithmetic op=ADD(w1149, w1148, w1147, w1146) -> (w1145:i16)
            n836 = Build Array(w1142, w1145, w1133, w1138, w1127, w1126, w1120, w1119) -> (w1129:i16[])
            n837 = Build Array (concatenate)(w1131, w1129) -> (w1130:i16[][])
            n838 = Build Array (concatenate)(w1132, w1129) -> (w1137:i16[][])
            n839 = Or(x=w1136, y=w1135) -> (x .or. y?=w1134:bool)
            n840 = local write "Session Performance"(w1130) -> ()
            n841 = local write "Mouse Performance"(w1137) -> ()
            n842 = Index Array(array=w1137, index (col)=1 ("disabled index (col)")) -> (element=→"Trial Outcomes":i16[])  [unwired: 1 in]
            n843 = local write "Correct?"(w1134) -> ()
            n844 = local write "Response Window"(0.0 ("Response Window")) -> ()
          }
        }
        n845 = local write "Trial State"(3 ("Trial State")) -> ()
        n846 = local read "Abort Protocol"() -> (w1114:bool)
        n847 = Select(t=MainProgramStates."End Training Protocol", s=w1114, f=MainProgramStates."Time Delay (Punishment)") -> (s? t:f=w1113:T18)
      }
      frame "Time Delay (Punishment)" {
        n848 = local write "Time Delay"(TRUE ("Pre trial")) -> ()
        n849 = local write "Response Window"(FALSE ("Intertrial Interval")) -> ()
        n850 = local read "False Alarm"() -> (w1164:bool)
        n851 = local write "Trial State"(4 ("Trial State")) -> ()
        n852 = case shown="True" w1164 {
          frame False {
          }
          frame True {
            n853 = for {
              N: "Punishment Period (s)" -> [_]
              stop <- w1170 stop-if-true
              n854 = local read "Abort Protocol"() -> (w1170:bool)
              n855 = Wait (ms)(milliseconds to wait=u32 1000) -> ()  [unwired: 1 out]
            }
          }
        }
        n856 = local read "Abort Protocol"() -> (w1166:bool)
        n857 = Select(t=MainProgramStates."End Training Protocol", s=w1166, f=MainProgramStates."Intertrial Interval") -> (s? t:f=w1165:T18)
      }
      frame "Intertrial Interval" {
        w1188 = 20 ("y")
        # "Todo: Save trial data here."
        n858 = property on="trialData" class="Clust (strict)"() -> ("Controls[]"=w1181:refnum<vi>[])  [unwired: 2 in, 2 out]
        n859 = local write "Trial State"(5 ("Trial State")) -> ()
        n860 = local write "Time Delay"(FALSE ("Intertrial Interval")) -> ()
        n861 = local write "Intertrial Interval"(TRUE ("Pre trial")) -> ()
        n862 = for {
          tunnel: w1181 -> [w1224] mode=indexing
          tunnel: [w1223] -> w1179 mode=indexing
          tunnel: [w1222] -> w1177 mode=indexing
          n863 = property class="Ctl"(reference=w1224) -> (error out=w1220:errorcluster, "Label.Text"=w1223:string, "Value"=w1221:variant)  [unwired: 1 in, 1 out]
          n864 = while {
            tunnel: [w1226] -> w1222
            tunnel: w1221 -> [w1230]
            tunnel: w1220 -> [w1229]
            i -> [w1227]
            stop <- w1228 continue-if-true
            n865 = case shown="2" w1227 {
              tunnel: w1230 -> [w1236 w1241 w1246]
              tunnel: w1229 -> [w1235 w1240 w1245]
              tunnel: [w1234 w1239 w1244] -> w1228
              tunnel: [w1231 w1237 w1242] -> w1225
              frame 0, Default {
                n866 = Variant To Data(error in=w1235, type=TRUE, Variant=w1236) -> (data=w1232:bool, error out=w1234:errorcluster)
                n867 = Boolean To (0,1)(Boolean=w1232) -> (0, 1=w1231:i16)
              }
              frame 1 {
                n868 = Variant To Data(error in=w1240, type=0, Variant=w1241) -> (data=w1237:i32, error out=w1239:errorcluster)
              }
              frame 2 {
                n869 = Variant To Data(error in=w1245, type=0.0, Variant=w1246) -> (data=w1242:dbl, error out=w1244:errorcluster)
              }
            }
            n870 = To Double Precision Float(number=w1225) -> (double precision float=w1226:dbl)
          }
        }
        n871 = local read "Mouse Performance"() -> (w1194:i16[][])
        n872 = local read "Selected Training Protocol"() -> (w1216:T10)
        n873 = local read "Intertrial interval (s)"() -> (w1182:i32)
        n874 = call "CountTrialOutcomes.vi"("Mouse Performance in"=w1194) -> ("nFalseAlarms"=w1196:i32, "nMiss"=w1197:i32, "nCorrect Rejections"=w1198:i32, "nHits"=w1199:i32, "nGoTrials"=w1195:i16, "nTrials"=w1190:i32)  [unwired: 5 in]
        n875 = Array Size(array=w1194) -> (size(s)=w1193:i32[])
        n876 = case shown="\"Rotations - Speed 45 deg/s\", Default" w1216 {
          tunnel: w1182 -> [w1261 _]
          frame "Rotations - Speed 45 deg/s", Default {
            n877 = for {
              N: w1261 -> [_]
              stop <- w1262 stop-if-true
              n878 = local read "Abort Protocol"() -> (w1262:bool)
              n879 = Wait (ms)(milliseconds to wait=u32 1000) -> ()  [unwired: 1 out]
            }
          }
          frame "Prerecording" {
          }
        }
        n880 = Index Array(array=w1193, index=0) -> (element=w1189:i32)
        n881 = call "CalculateTrialPerformance.vi"("nGoTrials"=w1195, "nTrials"=w1190, "nFalseAlarms"=w1196, "nMiss"=w1197, "nCorrect Rejections"=w1198, "nHits"=w1199) -> ("pCorrect"=w1186:dbl, "D'prime"=→"d'":dbl)  [unwired: 4 in]
        n882 = Multiply(x=w1186, y=100.0) -> (x*y=→"% correct":dbl)
        n883 = Greater Or Equal?(x=w1189, y=w1188) -> (x >= y?=w1187:bool)
        n884 = local read "trial data tdms fileref"() -> (w1172:refnum<k34>)
        n885 = local read "SessionID"() -> (w1173:string)
        n886 = case shown="True" w1187 {
          tunnel: w1194 -> [_ w1260]
          tunnel: w1189 -> [_ w1251]
          tunnel: w1188 -> [_ w1250]
          frame False {
          }
          frame True {
            n887 = Subtract(x=w1251, y=w1250) -> (x-y=w1259:i32)
            n888 = Array Subset(array=w1260, index (row)=w1259) -> (w1256:i16[][])  [unwired: 3 in]
            n889 = call "CountTrialOutcomes.vi"("Mouse Performance in"=w1256) -> ("nFalseAlarms"=w1257:i32, "nMiss"=w1253:i32, "nCorrect Rejections"=w1254:i32, "nHits"=w1255:i32, "nGoTrials"=w1258:i16, "nTrials"=w1252:i32)  [unwired: 5 in]
            n890 = call "CalculateTrialPerformance.vi"("nGoTrials"=w1258, "nTrials"=w1252, "nFalseAlarms"=w1257, "nMiss"=w1253, "nCorrect Rejections"=w1254, "nHits"=w1255) -> ("pCorrect"=w1248:dbl, "D'prime"=w1249:dbl)  [unwired: 4 in]
            n891 = Bundle("D'prime"=w1249, "pCorrect"=w1248) -> (→"Trial Performance":cluster{"D'prime":dbl, "pCorrect":dbl})  [unwired: 1 in]
          }
        }
        n892 = Array Size(array=w1177) -> (size(s)=w1175:i32)
        n893 = Reshape Array(w1177, 1 ("dimension size"), w1175) -> (w1174:dbl[][])
        n894 = TDMS Write(0:w1172, 1:enum16{"decimated", "interleaved"}."interleaved" ("data layout (0:decimated)"), 5:w1173, 7:w1179, 9:w1174) -> (4:w1178:refnum<k34>)  [unwired: 1 in, 3 out]
        n895 = local write "trial data tdms fileref"(w1178) -> ()
        n896 = local read "Trial Counter"() -> (w1219:i32)
        n897 = local read "nTrials"() -> (w1183:i32)
        n898 = local read "Abort Protocol"() -> (w1209:bool)
        n899 = Greater Or Equal?(x=w1219, y=w1183) -> (x >= y?=w1208:bool)
        n900 = local read "Pause"() -> (w1203:bool)
        n901 = local write "Hit"(FALSE ("Hit")) -> ()
        n902 = local write "Miss"(FALSE ("Miss")) -> ()
        n903 = local write "False Alarm"(FALSE ("False Alarm")) -> ()
        n904 = local write "Correct Rejection"(FALSE ("Correct Rejection")) -> ()
        n905 = local write "Go Trial?"(FALSE ("Go Trial?")) -> ()
        n906 = Or(x=w1208, y=w1209) -> (x .or. y?=w1210:bool)
        n907 = Select(t=MainProgramStates."Pause", s=w1203, f=MainProgramStates."Trial Initialization") -> (s? t:f=w1200:T18)
        n908 = Select(t=MainProgramStates."End Training Protocol", s=w1210, f=w1200) -> (s? t:f=w1217:T18)
      }
      frame "End Training Protocol" {
        w1287 = "Trial Performance"
        # "Writing To Channels"
        n909 = local read "Recording Start Time"() -> (w1278:u32)
        n910 = Tick Count (ms)() -> (millisecond timer value=w1279:u32)
        n911 = local read "tdms file performance"() -> (w1295:refnum<k34>)
        n912 = local read "Session Performance"() -> (w1304:i16[][])
        n913 = local read "SessionID"() -> (w1294:string)
        n914 = local write "Pre trial"(FALSE ("Pre trial")) -> ()
        n915 = local write "Cue"(FALSE ("Cue")) -> ()
        n916 = local write "Response Window"(FALSE ("Response Window")) -> ()
        n917 = local write "Time Delay"(FALSE ("Time Delay")) -> ()
        n918 = local write "Intertrial Interval"(FALSE ("Intertrial Interval")) -> ()
        n919 = local read "% correct"() -> (w1275:dbl)
        n920 = Subtract(x=w1279, y=w1278) -> (x-y=w1277:u32)
        n921 = Transpose 2D Array(2D array=w1304) -> (transposed array=w1303:i16[][])
        n922 = local write "Trial State"(0 ("Trial State")) -> ()
        n923 = property on="Selected Training Protocol" class="Enum (strict)"() -> ("RingText.Text"=w1297:string)  [unwired: 2 in, 2 out]
        n924 = local read "Go Trial Probability"() -> (w1286:dbl)
        n925 = local read "mL given"() -> (w1284:dbl)
        n926 = local read "NRewards"() -> (w1283:i32)
        n927 = local read "Trial Counter"() -> (w1282:i32)
        n928 = local read "Punishment Period (s)"() -> (w1281:i32)
        n929 = local read "Response Window (ms)"() -> (w1280:u32)
        n930 = local read "Airpuff (ms)"() -> (w1269:u32)
        n931 = call "TDMSFormatGroupProperties.vi"("mL given"=w1284, "Go Trial Probability"=w1286, "RingText.Text"=w1297, "NRewards"=w1283, "Session Performance"=w1275, "Trial Counter"=w1282, "Training Duration (ms)"=w1277, "Punishment Period (s)"=w1281, "Airpuff (ms)"=w1269, "Response Window (ms)"=w1280) -> ("Property Values"=w1296:string[], "Property names"=w1298:string[])  [unwired: 4 in]
        n932 = TDMS Set Properties(5:w1296, 7:w1298, 10:w1294, 11:w1295) -> (2:w1292:string, 3:w1293:refnum<k34>)  [unwired: 2 in, 2 out]
        n933 = Build Array(4.0 ("element"), 3.0 ("element"), 2.0 ("element"), 1.0 ("element")) -> (w1308:dbl[])
        n934 = TDMS Set Properties(5:w1308, 7:string[] ["Hit", "Correct Rejection", "Miss", "False Alarm"] ("property names"), 9:w1287, 10:w1292, 11:w1293) -> (2:w1290:string, 3:w1291:refnum<k34>)  [unwired: 1 in, 2 out]
        n935 = local read "LostFrames Security Camera"() -> (w1272:u32)
        n936 = local read "LostFrames"() -> (w1271:u32)
        n937 = local write "Response Window"(0.0 ("Response Window")) -> ()
        n938 = local read "dataInfo"() -> (w1274:T5)
        n939 = Bundle By Name(cluster=w1274, "nFramesLostPupil"=w1271, "nFramesLostSecurity"=w1272) -> (w1273:T5)
        n940 = local write "Hit"(FALSE ("Hit")) -> ()
        n941 = local write "Miss"(FALSE ("Miss")) -> ()
        n942 = local write "False Alarm"(FALSE ("False Alarm")) -> ()
        n943 = local write "Correct Rejection"(FALSE ("Correct Rejection")) -> ()
        n944 = local read "trial data tdms fileref"() -> (w1264:refnum<k34>)
        n945 = Build Array("Trial No" ("element"), w1287, "Trial Type" ("element"), "Response Time" ("element"), "Stage Speed" ("element"), "Wall Speed" ("element"), "Stage Acceleration" ("element"), "Wall Acceleration" ("element")) -> (w1307:string[])
        n946 = local write "Go Trial?"(FALSE ("Go Trial?")) -> ()
        n947 = TDMS Write(0:w1291, 5:w1290, 7:w1307, 9:w1303) -> (4:w1289:refnum<k34>, 15:w1288:errorcluster)  [unwired: 2 in, 2 out]
        n948 = local write "dataInfo"(w1273) -> ()
        n949 = TDMS Close(11:w1264) -> ()  [unwired: 1 in, 2 out]
        n950 = TDMS Close(8:w1288, 11:w1289) -> ()  [unwired: 2 out]
      }
      frame "End Recording" {
        # "Stop eye tracking and data logging"
        n951 = flat-sequence {
          tunnel: [TRUE ("Value (Signaling)")] -> w1327
          frame #0 {
            n952 = local write "Leave Acquisition Run State"(DataAquisitionStates."End Data Logging") -> ()
            n953 = local write "Stop Data Logging"(TRUE ("Start Data Logging")) -> ()
          }
          frame #1 {
            n954 = while {
              stop <- w1370 continue-if-true
              n955 = local read "Stop Data Logging"() -> (w1370:bool)
              n956 = Wait (ms)(milliseconds to wait=u32 30) -> ()  [unwired: 1 out]
            }
          }
        }
        n957 = local read "SciScan RecordSignal"() -> (w1357:refnum<k21>)
        n958 = local read "RecordingFolder"() -> (w1330:path)
        n959 = local read "GoogleDriveFolder"() -> (w1341:path)
        n960 = local read "dataInfo"() -> (w1337:T5)
        n961 = call-poly <vilib>:"DAQmx Write.vi"("task/channels in"=w1357, "data"=FALSE) -> ("task out"=w1358:refnum<k21>)  [unwired: 11 in, 2 out]
        n962 = Flatten To XML(anything=w1337) -> (xml string=w1336:string)
        n963 = Strip Path(path=w1330) -> (stripped path=w1329:path)  [unwired: 1 out]
        n964 = Strip Path(path=w1341) -> (stripped path=w1340:path)  [unwired: 1 out]
        n965 = local read "SessionID"() -> (w1335:string)
        n966 = call <vilib>:"DAQmx Stop Task.vi"("task/channels in"=w1358) -> ("task out"=w1360:refnum<k21>)  [unwired: 13 in, 1 out]
        n967 = local write "SciScan RecordSignal"(w1360) -> ()
        n968 = Concatenate Strings(w1335, "-recording_metadata" ("string"), ".xml" ("string")) -> (w1333:string)
        n969 = Build Path(base path=w1329, name or relative path=w1333) -> (appended path=w1332:path)
        n970 = Build Path(base path=w1329, name or relative path=w1333) -> (appended path=w1331:path)
        n971 = call-poly <vilib>:"Write to XML File.vi"("XML Input"=w1336, "XML File Path"=w1331) -> ()  [unwired: 7 in, 3 out]
        n972 = call-poly <vilib>:"Write to XML File.vi"("XML Input"=w1336, "XML File Path"=w1332) -> ()  [unwired: 7 in, 3 out]
        n973 = property on="Print Screen" class="Bool (strict)"("Val(Sgnl)"=w1327) -> ()  [unwired: 2 in, 2 out]
        n974 = local read "Abort Protocol"() -> (w1322:bool)
        n975 = local read "LightsOnSession"() -> (w1324:bool)
        n976 = local read "sessionInfo"() -> (w1351:T7)
        n977 = Get Date/Time In Seconds() -> (seconds since 1Jan1904=w1353:timestamp)
        n978 = local read "Security Camera Connected"() -> (w1339:bool)
        n979 = local read "DemoCamera Connected"() -> (w1325:bool)
        n980 = local read "Pupil Camera Connected"() -> (w1354:bool)
        n981 = Get Date/Time String(seconds (now)=w1353, want seconds? (F)=TRUE) -> (time string=w1350:string)  [unwired: 1 in, 1 out]
        n982 = Bundle By Name(cluster=w1351, "sessionEnded"=w1350, "LightsOn"=w1324, "wasSessionAborted"=w1322) -> (w1346:T7)
        n983 = case shown="True" w1339 {
          frame False {
          }
          frame True {
            n984 = global write "GlobalVariables.vi" "save data"(FALSE ("Save Images")) -> ()
          }
        }
        n985 = case shown="True" w1354 {
          frame False {
          }
          frame True {
            n986 = local write "Save Pupil Video"(FALSE ("Save Images")) -> ()
            n987 = property on="Save Tracking Results" class="Bool (strict)"("Val(Sgnl)"=TRUE ("Value (Signaling)")) -> ()  [unwired: 2 in, 2 out]
            n988 = local write "Track Pupil"(FALSE ("Start / Stop Tracking")) -> ()
          }
        }
        n989 = case shown="True" w1325 {
          frame False {
          }
          frame True {
            n990 = local write "SaveDemoVideo"(FALSE ("Save Images")) -> ()
          }
        }
        n991 = local write "sessionInfo"(w1346) -> ()
        n992 = Flatten To XML(anything=w1346) -> (xml string=w1345:string)
        n993 = local read "SessionID"() -> (w1347:string)
        n994 = Concatenate Strings("sessioninfo-" ("string"), w1347, ".xml" ("string")) -> (w1344:string)
        n995 = Build Path(base path=w1329, name or relative path=w1344) -> (appended path=w1343:path)
        n996 = Build Path(base path=w1340, name or relative path=w1344) -> (appended path=w1342:path)
        n997 = local write "Session Running"(FALSE ("Session Running")) -> ()
        n998 = local write "Start Protocol"(FALSE ("Start Protocol")) -> ()
        n999 = property on="Lights On" class="Bool (strict)"("Val(Sgnl)"=TRUE ("Value (Signaling)")) -> ()  [unwired: 2 in, 2 out]
        n1000 = call-poly <vilib>:"Write to XML File.vi"("XML Input"=w1345, "XML File Path"=w1343) -> ()  [unwired: 7 in, 3 out]
        n1001 = call-poly <vilib>:"Write to XML File.vi"("XML Input"=w1345, "XML File Path"=w1342) -> ()  [unwired: 7 in, 3 out]
      }
      frame "Reset Session Data" {
        # "Prepare Recording Name for Next Session"
        n1002 = local read "Abort Protocol"() -> (w1372:bool)
        n1003 = local read "Recording No"() -> (w1374:i32)
        n1004 = disable-structure shown="Disabled" {
          frame Disabled {
            n1005 = flat-sequence {
              frame #0 {
                # "Wait for video recordings to finish"
                n1006 = local read "Security Camera Connected"() -> (w1397:bool)
                n1007 = local read "Pupil Camera Connected"() -> (w1398:bool)
                n1008 = local read "DemoCamera Connected"() -> (w1396:bool)
                n1009 = while {
                  tunnel: w1398 -> [w1409]
                  tunnel: w1397 -> [w1408]
                  tunnel: w1396 -> [w1403]
                  stop <- w1399 continue-if-true
                  w1405 = FALSE ("f")
                  n1010 = local read "Recording Pupil Video"() -> (w1407:bool)
                  n1011 = local read "Recording Security Video"() -> (w1406:bool)
                  n1012 = local read "Recording Demo Video"() -> (w1404:bool)
                  n1013 = Select(t=w1407, s=w1409, f=w1405) -> (s? t:f=w1400:bool)
                  n1014 = Select(t=w1406, s=w1408, f=w1405) -> (s? t:f=w1401:bool)
                  n1015 = Select(t=w1404, s=w1403, f=w1405) -> (s? t:f=w1402:bool)
                  n1016 = Compound Arithmetic op=OR(w1400, w1401, w1402) -> (w1399:bool)
                  n1017 = Wait (ms)(milliseconds to wait=u32 10) -> ()  [unwired: 1 out]
                }
              }
              frame #1 {
                n1018 = local read "Security Camera Connected"() -> (w1411:bool)
                n1019 = case shown="True" w1411 {
                  frame False {
                  }
                  frame True {
                    n1020 = local read "AVI Refnum - Body"() -> (w1412:T8)
                    n1021 = call "IMAQ AVI2 Close"("AVI Refnum"=w1412) -> ()  [unwired: 10 in, 1 out]
                  }
                }
              }
            }
          }
          frame Enabled {
          }
        }
        n1022 = Increment(x=w1374) -> (x+1=w1373:i32)
        n1023 = case shown="True" w1372 {
          frame False {
          }
          frame True {
            n1024 = property on="Abort Protocol" class="Bool (strict)"("DisabledEnum"=T22."Enabled" ("Disabled")) -> ()  [unwired: 2 in, 2 out]
            n1025 = local write "Abort Protocol"(FALSE ("Abort Protocol")) -> ()
          }
        }
        n1026 = property on="Recording No" class="DigNum (strict)"("Val(Sgnl)"=w1373) -> ()  [unwired: 2 in, 2 out]
        n1027 = disable-structure shown="Disabled" {
          frame Disabled {
            n1028 = local write "Trial Counter"(0 ("Trial Counter")) -> ()
            n1029 = local write "NGoTrials"(0 ("NGoTrials")) -> ()
            n1030 = local write "NRewards"(0 ("NRewards")) -> ()
            n1031 = local write "nCorrect"(0 ("nCorrect")) -> ()
          }
          frame Enabled {
          }
        }
        n1032 = local write "Reset Lost Frames"(TRUE ("Reset Lost Frames")) -> ()
        n1033 = invoke on="Session Performance" class="Arr (strict)" method="Reinit To Default"() -> ()  [unwired: 3 in, 3 out]
        n1034 = invoke on="sessionInfo" class="Clust (strict)" method="Reinit To Default"() -> ()  [unwired: 3 in, 3 out]
        n1035 = local read "Session Checklist"() -> (w1377:T2)
        n1036 = invoke on="trialData" class="Clust (strict)" method="Reinit To Default"() -> ()  [unwired: 3 in, 3 out]
        n1037 = Bundle By Name(cluster=w1377, "Experiment Name"=FALSE ("Security Camera"), "Trigger On"=FALSE ("Lickport In Place"), "FOV Position"=FALSE ("Pupil Camera"), "Closed Curtain"=FALSE ("Pupil Cropped")) -> (w1378:T2)
        n1038 = local write "Session Checklist"(w1378) -> ()
        n1039 = local read "Wall Position"() -> (w1381:dbl)
        n1040 = local read "Stage Position"() -> (w1390:dbl)
        n1041 = In Range and Coerce(upper limit=1.0, x=w1390, lower limit=-1.0) -> (In Range?=w1387:bool)  [unwired: 1 out]
        n1042 = In Range and Coerce(upper limit=1.0, x=w1381, lower limit=-1.0) -> (In Range?=w1384:bool)  [unwired: 1 out]
        n1043 = Not(x=w1387) -> (.not. x?=w1386:bool)
        n1044 = Not(x=w1384) -> (.not. x?=w1385:bool)
        n1045 = case shown="True" w1386 {
          frame False {
          }
          frame True {
            # "Move Home"
            n1046 = call "SMMoveAbsolute.vi"() -> ()  [unwired: 12 in]
          }
        }
        n1047 = case shown="True" w1385 {
          frame False {
          }
          frame True {
            n1048 = property on="BtnWallMoveHome" class="Bool (strict)"("Val(Sgnl)"=TRUE ("Value (Signaling)")) -> ()  [unwired: 2 in, 2 out]
          }
        }
      }
      frame "Pause" {
        n1049 = while {
          stop <- "Pause" continue-if-true
          n1050 = Wait (ms)(milliseconds to wait=u32 30) -> ()  [unwired: 1 out]
        }
      }
      frame "Quit Main Program" {
        n1051 = local read "Saved Values"() -> (w1422:refnum<vi>[])
        n1052 = global write "GlobalVariables.vi" "quit program"(TRUE ("quit program")) -> ()
        n1053 = call "Read and Write Controls to Automatic Config File.vi"("Action"=RWC_Actions."Write", "Control References"=w1422) -> ()  [unwired: 9 in, 1 out]
      }
      frame "Load Modules" {
        n1054 = local read "Wall connected"() -> (w1426:bool)
        n1055 = case shown="True" "Security Camera Connected" {
          selector: "Security Camera Connected" -> [_ w1431]
          frame False {
          }
          frame True {
            n1056 = property on="Security Camera Connected" class="Bool (strict)"("Val(Sgnl)"=w1431) -> ()  [unwired: 2 in, 2 out]
          }
        }
        n1057 = case shown="True" w1426 {
          selector: w1426 -> [_ w1430]
          frame False {
          }
          frame True {
            n1058 = property on="Wall connected" class="Bool (strict)"("Val(Sgnl)"=w1430) -> ()  [unwired: 2 in, 2 out]
          }
        }
      }
    }
  }
  n1059 = while {
    shift-right: [w1435] -> _
    shift-left: w15 -> [w1436]
    shift-right: [w1433] -> _
    shift-left: _ -> [w1432]
    stop <- w1434 stop-if-true
    # "Event Loop. All triggered events are carried out in this loop"
    n1060 = case shown="\"Running\", Default" w1436 {
      tunnel: [EventLoopStates."Running" w1452 EventLoopStates."Quit Event Loop"] -> w1435
      tunnel: [w1437 w1450 w2121] -> w1433
      tunnel: w1432 -> [_ w1451 w2121]
      frame "Init Event Loop" {
        # "Status Indicators"
        # "Event Buttons"
        # "Beeper TTL Output"
        # "Water Valve (Solenoid) TTL Output"
        n1061 = property on="Reward Green Light" class="Bool (strict)"("Visible"=FALSE) -> ()  [unwired: 2 in, 2 out]
        n1062 = property on="RecordingID" class="Str"("Visible"=TRUE) -> ()  [unwired: 2 in, 2 out]
        n1063 = property on="Recording No" class="DigNum (strict)"("Visible"=TRUE) -> ()  [unwired: 2 in, 2 out]
        n1064 = call-poly <vilib>:"DAQmx Create Virtual Channel.vi"("lines"="RoofLights") -> ("task out"=w1438:refnum<k21>)  [unwired: 13 in, 1 out]
        n1065 = call-poly <vilib>:"DAQmx Create Virtual Channel.vi"("lines"="Water Valve Line") -> ("task out"=w1440:refnum<k21>)  [unwired: 13 in, 1 out]
        n1066 = call-poly <vilib>:"DAQmx Create Virtual Channel.vi"("lines"="Airpuff Line") -> ("task out"=w1439:refnum<k21>)  [unwired: 13 in, 1 out]
        n1067 = Bundle By Name(cluster=T26 {"Water Valve"="", "Airpuff"="", "Light Switch"=""} ("input cluster"), "Water Valve"=w1440, "Airpuff"=w1439, "Light Switch"=w1438) -> (w1437:T26)
        "Stepper Prepared for Rotation" <- FALSE ("Stepper Prepared for Rotation")
      }
      frame "Running", Default {
        n1068 = event shown="[3] \"Rotate Full\": Mouse Down" {
          selector: _ -> [_ _ _ _ _ _ _ _ _ _ _ _ _ _ _ _ _ _ _ _ _ _ _ _ _ _ _ _ _ _ _ _ _ _ _ _ _ _]
          dyn-events: _ -> [_ _ _ _ _ _ _ _ _ _ _ _ _ _ _ _ _ _ _ _ _ _ _ _ _ _ _ _ _ _ _ _ _ _ _ _ _ _]
          timeout: 30 -> [_ _ _ _ _ _ _ _ _ _ _ _ _ _ _ _ _ _ _ _ _ _ _ _ _ _ _ _ _ _ _ _ _ _ _ _ _ _]
          tunnel: [EventLoopStates."Running" _ _ _ EventLoopStates."Running" _ _ _ EventLoopStates."Running" EventLoopStates."Running" EventLoopStates."Running" EventLoopStates."Running" EventLoopStates."Running" EventLoopStates."Running" EventLoopStates."Running" EventLoopStates."Running" EventLoopStates."Running" EventLoopStates."Running" EventLoopStates."Running" EventLoopStates."Running" _ _ EventLoopStates."Running" _ EventLoopStates."Running" EventLoopStates."Running" EventLoopStates."Running" EventLoopStates."Running" EventLoopStates."Running" EventLoopStates."Running" EventLoopStates."Running" EventLoopStates."Running" EventLoopStates."Running" EventLoopStates."Running" EventLoopStates."Running" EventLoopStates."Running" EventLoopStates."Running" EventLoopStates."Quit Event Loop"] -> w1452
          tunnel: w1451 -> [w1454 _ _ _ w1602 _ _ w1659 w1682 w1687 w1707 w1716 w1721 w1726 w1746 w1766 w1786 w1806 w1825 w1835 _ _ w1905 _ w1942 w1947 w1970 w1987 w1996 w2001 w2020 w2033 w2039 w2047 w2057 w2065 w2111 w2115]
          tunnel: [w1454 _ _ _ w1602 _ _ w1659 w1681 w1687 w1707 w1716 w1721 w1726 w1746 w1766 w1786 w1806 w1825 w1834 _ _ w1905 _ w1942 w1947 w1970 w1987 w1996 w2001 w2018 w2032 w2039 w2047 w2055 w2064 w2111 w2115] -> w1450
          event Timeout {
            n1069 = event-data() -> ()  [unwired: 1 in, 3 out]
            n1070 = local read "Stepper Prepared for Rotation"() -> (w1456:bool)
            n1071 = Tick Count (ms)() -> (millisecond timer value=w1466:u32)
            n1072 = local read "cue time"() -> (w1465:u32)
            n1073 = local read "Waiting for lick"() -> (w1463:bool)
            n1074 = Subtract(x=w1466, y=w1465) -> (x-y=w1464:u32)
            n1075 = local read "Init Stepper Move"() -> (w1457:bool)
            n1076 = Greater?(x=w1464, y="Response Window (ms)") -> (0:w1462:bool)
            n1077 = Not(x=w1456) -> (.not. x?=w1455:bool)
            n1078 = And(x=w1463, y=w1462) -> (x .and. y?=w1461:bool)
            n1079 = case shown="True" w1461 {
              frame False {
              }
              frame True {
                n1080 = property on="Response Timeout" class="Bool (strict)"("Val(Sgnl)"=TRUE ("Value (Signaling)")) -> ()  [unwired: 2 in, 2 out]
              }
            }
            n1081 = And(x=w1455, y=w1457) -> (x .and. y?=w1458:bool)
            n1082 = case shown="True" w1458 {
              frame False {
              }
              frame True {
                n1083 = local write "Stepper Prepared for Rotation"(TRUE ("Stepper Prepared for Rotation")) -> ()
                n1084 = property on="Wall Speed (deg/s)" class="DigNum (strict)"() -> (error out=w1469:errorcluster, "Value"=w1468:dbl)  [unwired: 2 in, 1 out]
                n1085 = property on="Wall Speed (deg/s)" class="DigNum (strict)"(error in=w1469, "Val(Sgnl)"=w1468) -> ()  [unwired: 1 in, 2 out]
              }
            }
          }
          event "Align Stage": Mouse Down {
            n1086 = event-data() -> ()  [unwired: 1 in, 8 out]
            n1087 = flat-sequence {
              tunnel: w1478 -> [w1492]
              tunnel: [w1490] -> w1488
              tunnel: [w1495] -> w1483
              tunnel: w1488 -> [w1495]
              tunnel: w1483 -> [w1499]
              tunnel: [w1499] -> w1481
              tunnel: w1482 -> [w1498]
              tunnel: w1481 -> [w1501]
              tunnel: [w1501] -> w1480
              tunnel: w1484 -> [w1506]
              tunnel: w1485 -> [w1505]
              tunnel: w1480 -> [w1503]
              tunnel: [w1503] -> w1477
              tunnel: w1477 -> [w1507]
              tunnel: [w1507] -> w1476
              tunnel: [w1510] -> w1487
              tunnel: w1476 -> [w1510]
              tunnel: w1487 -> [w1513]
              tunnel: [w1512] -> w1486
              tunnel: w1486 -> [w1516]
              tunnel: w1485 -> [w1518]
              tunnel: w1484 -> [w1517]
              tunnel: [w1516] -> w1479
              frame #0 {
                n1088 = call <vilib>:"DAQmx Start Task.vi"("task/channels in"=w1492) -> ("task out"=w1491:refnum<k21>)  [unwired: 13 in, 1 out]
                n1089 = call-poly <vilib>:"DAQmx Write.vi"("task/channels in"=w1491, "data"=TRUE) -> ("task out"=w1490:refnum<k21>)  [unwired: 11 in, 2 out]
              }
              frame #1 {
                n1090 = while {
                  stop <- w1497 continue-if-true
                  n1091 = local read "Stage Moving?"() -> (w1497:bool)
                  n1092 = Wait (ms)(milliseconds to wait=u32 30) -> ()  [unwired: 1 out]
                }
                n1093 = Wait (ms)(milliseconds to wait=u32 5000) -> ()  [unwired: 1 out]
              }
              frame #2 {
                n1094 = call "Trigger2Photon.vi"("Refnum in"=w1498) -> ()  [unwired: 9 in, 2 out]
              }
              frame #3 {
                n1095 = Wait (ms)(milliseconds to wait=u32 5000) -> ()  [unwired: 1 out]
              }
              frame #4 {
                n1096 = call "SMMoveRelative.vi"("Displacement"=180.0, "Acceleration"=w1506, "Speed"=w1505) -> ("Move success"=w1502:bool)  [unwired: 8 in]
                n1097 = local write "Stage Moving?"(w1502) -> ()
              }
              frame #5 {
                n1098 = while {
                  stop <- w1509 continue-if-true
                  n1099 = local read "Stage Moving?"() -> (w1509:bool)
                  n1100 = Wait (ms)(milliseconds to wait=u32 30) -> ()  [unwired: 1 out]
                }
              }
              frame #6 {
                n1101 = Wait (ms)(milliseconds to wait=u32 5000) -> ()  [unwired: 1 out]
              }
              frame #7 {
                n1102 = call-poly <vilib>:"DAQmx Write.vi"("task/channels in"=w1513, "data"=FALSE) -> ("task out"=w1514:refnum<k21>)  [unwired: 11 in, 2 out]
                n1103 = call <vilib>:"DAQmx Stop Task.vi"("task/channels in"=w1514) -> ("task out"=w1512:refnum<k21>)  [unwired: 13 in, 1 out]
              }
              frame #8 {
                n1104 = call "SMMoveRelative.vi"("Displacement"=-180.0, "Acceleration"=w1517, "Speed"=w1518) -> ()  [unwired: 8 in, 1 out]
              }
            }
            n1105 = local read "SciScan RecordSignal"() -> (w1478:refnum<k21>)
            n1106 = local read "2P TriggerLine"() -> (w1482:refnum<k21>)
            n1107 = local read "Stage Position"() -> (w1473:dbl)
            n1108 = In Range and Coerce(upper limit=1.0, x=w1473, lower limit=-1.0) -> (In Range?=w1471:bool)  [unwired: 1 out]
            n1109 = Not(x=w1471) -> (.not. x?=w1472:bool)
            n1110 = local read "Stage Acceleration (deg2/s)"() -> (w1484:dbl)
            n1111 = case shown="True" w1472 {
              selector: w1472 -> [_ w1489]
              frame False {
              }
              frame True {
                # "Move Home"
                n1112 = call "SMMoveAbsolute.vi"() -> ()  [unwired: 12 in]
                n1113 = local write "Stage Moving?"(w1489) -> ()
              }
            }
            n1114 = local read "Stage Speed (deg/s)"() -> (w1485:dbl)
            n1115 = local write "SciScan RecordSignal"(w1479) -> ()
          }
          event "Destretch Calibrate": Mouse Down {
            n1116 = event-data() -> ()  [unwired: 1 in, 8 out]
            n1117 = flat-sequence {
              tunnel: w1522 -> [w1535]
              tunnel: [w1533] -> w1532
              tunnel: [w1538] -> w1527
              tunnel: w1532 -> [w1538]
              tunnel: w1527 -> [w1540]
              tunnel: [w1540] -> w1525
              tunnel: w1526 -> [w1539]
              tunnel: w1525 -> [w1542]
              tunnel: [w1542] -> w1524
              tunnel: w1528 -> [w1547]
              tunnel: w1529 -> [w1546]
              tunnel: w1524 -> [w1544]
              tunnel: [w1544] -> w1521
              tunnel: w1521 -> [w1548]
              tunnel: [w1548] -> w1520
              tunnel: [w1551] -> w1531
              tunnel: w1520 -> [w1551]
              tunnel: w1531 -> [w1554]
              tunnel: [w1553] -> w1530
              tunnel: w1530 -> [w1557]
              tunnel: w1529 -> [w1559]
              tunnel: w1528 -> [w1558]
              tunnel: [w1557] -> w1523
              frame #0 {
                n1118 = call <vilib>:"DAQmx Start Task.vi"("task/channels in"=w1535) -> ("task out"=w1534:refnum<k21>)  [unwired: 13 in, 1 out]
                n1119 = call-poly <vilib>:"DAQmx Write.vi"("task/channels in"=w1534, "data"=TRUE) -> ("task out"=w1533:refnum<k21>)  [unwired: 11 in, 2 out]
              }
              frame #1 {
                n1120 = Wait (ms)(milliseconds to wait=u32 5000) -> ()  [unwired: 1 out]
              }
              frame #2 {
                n1121 = call "Trigger2Photon.vi"("Refnum in"=w1539) -> ()  [unwired: 9 in, 2 out]
              }
              frame #3 {
                n1122 = Wait (ms)(milliseconds to wait=u32 5000) -> ()  [unwired: 1 out]
              }
              frame #4 {
                n1123 = call "SMMoveRelative.vi"("Displacement"=90.0, "Acceleration"=w1547, "Speed"=w1546) -> ("Move success"=w1543:bool)  [unwired: 8 in]
                n1124 = local write "Stage Moving?"(w1543) -> ()
              }
              frame #5 {
                n1125 = while {
                  stop <- w1550 continue-if-true
                  n1126 = local read "Stage Moving?"() -> (w1550:bool)
                  n1127 = Wait (ms)(milliseconds to wait=u32 30) -> ()  [unwired: 1 out]
                }
              }
              frame #6 {
                n1128 = Wait (ms)(milliseconds to wait=u32 5000) -> ()  [unwired: 1 out]
              }
              frame #7 {
                n1129 = call-poly <vilib>:"DAQmx Write.vi"("task/channels in"=w1554, "data"=FALSE) -> ("task out"=w1555:refnum<k21>)  [unwired: 11 in, 2 out]
                n1130 = call <vilib>:"DAQmx Stop Task.vi"("task/channels in"=w1555) -> ("task out"=w1553:refnum<k21>)  [unwired: 13 in, 1 out]
              }
              frame #8 {
                n1131 = call "SMMoveRelative.vi"("Displacement"=-90.0, "Acceleration"=w1558, "Speed"=w1559) -> ()  [unwired: 8 in, 1 out]
              }
            }
            n1132 = local read "Stage Speed (deg/s)"() -> (w1529:dbl)
            n1133 = local read "Stage Acceleration (deg2/s)"() -> (w1528:dbl)
            n1134 = local read "SciScan RecordSignal"() -> (w1522:refnum<k21>)
            n1135 = local read "2P TriggerLine"() -> (w1526:refnum<k21>)
            n1136 = local write "SciScan RecordSignal"(w1523) -> ()
          }
          event "Rotate Full": Mouse Down {
            n1137 = event-data() -> ()  [unwired: 1 in, 8 out]
            n1138 = flat-sequence {
              tunnel: w1565 -> [w1576]
              tunnel: [w1574] -> w1573
              tunnel: [w1579] -> w1572
              tunnel: w1573 -> [w1579]
              tunnel: w1572 -> [w1581]
              tunnel: [w1581] -> w1571
              tunnel: w1564 -> [w1580]
              tunnel: w1571 -> [w1583]
              tunnel: [w1583] -> w1570
              tunnel: w1563 -> [w1588]
              tunnel: 25.0 ("Stage Speed (deg/s)") -> [w1587]
              tunnel: w1570 -> [w1585]
              tunnel: [w1585] -> w1569
              tunnel: w1569 -> [w1589]
              tunnel: [w1589] -> w1568
              tunnel: [w1592] -> w1567
              tunnel: w1568 -> [w1592]
              tunnel: w1567 -> [w1595]
              tunnel: [w1594] -> w1566
              tunnel: w1566 -> [w1598]
              tunnel: 50.0 ("Stage Speed (deg/s)") -> [w1600]
              tunnel: w1563 -> [w1599]
              tunnel: [w1598] -> _
              frame #0 {
                n1139 = call <vilib>:"DAQmx Start Task.vi"("task/channels in"=w1576) -> ("task out"=w1575:refnum<k21>)  [unwired: 13 in, 1 out]
                n1140 = call-poly <vilib>:"DAQmx Write.vi"("task/channels in"=w1575, "data"=TRUE) -> ("task out"=w1574:refnum<k21>)  [unwired: 11 in, 2 out]
              }
              frame #1 {
                n1141 = Wait (ms)(milliseconds to wait=u32 5000) -> ()  [unwired: 1 out]
              }
              frame #2 {
                n1142 = call "Trigger2Photon.vi"("Refnum in"=w1580) -> ()  [unwired: 9 in, 2 out]
              }
              frame #3 {
                n1143 = Wait (ms)(milliseconds to wait=u32 1000) -> ()  [unwired: 1 out]
              }
              frame #4 {
                n1144 = call "SMMoveRelative.vi"("Displacement"=360.0, "Acceleration"=w1588, "Speed"=w1587) -> ("Move success"=w1584:bool)  [unwired: 8 in]
                n1145 = local write "Stage Moving?"(w1584) -> ()
              }
              frame #5 {
                n1146 = while {
                  stop <- w1591 continue-if-true
                  n1147 = local read "Stage Moving?"() -> (w1591:bool)
                  n1148 = Wait (ms)(milliseconds to wait=u32 30) -> ()  [unwired: 1 out]
                }
              }
              frame #6 {
                n1149 = Wait (ms)(milliseconds to wait=u32 1000) -> ()  [unwired: 1 out]
              }
              frame #7 {
                n1150 = call-poly <vilib>:"DAQmx Write.vi"("task/channels in"=w1595, "data"=FALSE) -> ("task out"=w1596:refnum<k21>)  [unwired: 11 in, 2 out]
                n1151 = call <vilib>:"DAQmx Stop Task.vi"("task/channels in"=w1596) -> ("task out"=w1594:refnum<k21>)  [unwired: 13 in, 1 out]
              }
              frame #8 {
                n1152 = call "SMMoveRelative.vi"("Displacement"=-360.0, "Acceleration"=w1599, "Speed"=w1600) -> ()  [unwired: 8 in, 1 out]
              }
            }
            n1153 = disable-structure shown="Disabled" {
              frame Disabled {
                n1154 = local read "Stage Speed (deg/s)"() -> ()  [unwired: 1 out]
              }
              frame Enabled {
              }
            }
            n1155 = local read "Stage Acceleration (deg2/s)"() -> (w1563:dbl)
            n1156 = local read "SciScan RecordSignal"() -> (w1565:refnum<k21>)
            n1157 = local read "2P TriggerLine"() -> (w1564:refnum<k21>)
          }
          event "Security Camera Connected": Value Change {
            n1158 = event-data() -> ("NewVal"=w1606:bool)  [unwired: 1 in, 5 out]
            n1159 = Open VI Reference(vi path=path "F:/Development/labview software/SecurityCamera/SecurityCamera.vi") -> (vi reference=w1604:refnum<vi>)  [unwired: 5 in, 1 out]
            n1160 = case shown="True" w1606 {
              tunnel: w1604 -> [w1609 w1614]
              frame False {
                n1161 = property class="VI"(reference=w1609) -> (reference out=w1607:refnum<vi>, "Exec.State"=w1608:T28)  [unwired: 1 in, 1 out]
                n1162 = case shown="\"Run top level\"" w1608 {
                  tunnel: w1607 -> [_ _ w1611 w1612]
                  frame "Bad", Default {
                  }
                  frame "Idle" {
                  }
                  frame "Run top level" {
                    n1163 = invoke class="VI" method="Abort VI"(reference=w1611) -> (reference out=w1610:refnum<vi>)  [unwired: 2 in, 2 out]
                    n1164 = invoke class="VI" method="FP.Close"(reference=w1610) -> ()  [unwired: 2 in, 3 out]
                  }
                  frame "Running" {
                    n1165 = invoke class="VI" method="Abort VI"(reference=w1612) -> ()  [unwired: 2 in, 3 out]
                  }
                }
              }
              frame True {
                n1166 = while {
                  tunnel: w1614 -> [w1618]
                  tunnel: [w1618] -> w1613
                  stop <- w1619 stop-if-true
                  n1167 = property class="VI"(reference=w1618) -> (reference out=w1621:refnum<vi>, "Exec.State"=w1622:T28)  [unwired: 1 in, 1 out]
                  n1168 = Wait (ms)(milliseconds to wait=u32 100) -> ()  [unwired: 1 out]
                  n1169 = case shown="\"Run top level\", \"Running\"" w1622 {
                    tunnel: w1621 -> [_ _ w1624]
                    tunnel: [_ TRUE _] -> w1619
                    frame "Bad", Default {
                    }
                    frame "Idle" {
                    }
                    frame "Run top level", "Running" {
                      n1170 = invoke class="VI" method="Abort VI"(reference=w1624) -> ()  [unwired: 2 in, 3 out]
                    }
                  }
                }
                n1171 = invoke class="VI" method="Run VI"(reference=w1613, "Wait until done"=FALSE ("Wait Until Done"), "Auto Dispose Ref"=TRUE ("Auto Dispose Reference")) -> (reference out=w1617:refnum<vi>)  [unwired: 2 in, 4 out]
                n1172 = invoke on="Mouse Security Camera" class="SubPanel" method="Insert VI"("VI Ref"=w1617) -> ()  [unwired: 3 in, 4 out]
                n1173 = disable-structure shown="Disabled" {
                  disable-tunnel: w1617 -> [w1625 _]
                  frame Disabled {
                    n1174 = invoke class="VI" method="FP.Open"(reference=w1625, "Activate"=TRUE ("Activate?"), "State"=T27."Standard") -> (reference out=w1627:refnum<vi>)  [unwired: 2 in, 4 out]
                    n1175 = property class="VI"(reference=w1627, "Front Panel.IsFrontmost"=FALSE ("Front Panel Window:Is Frontmost")) -> ()  [unwired: 1 in, 2 out]
                  }
                  frame Enabled {
                  }
                }
              }
            }
          }
          event "BtnStageSmallStep": Mouse Down {
            n1176 = event-data() -> ()  [unwired: 1 in, 8 out]
            n1177 = local read "Select Rotation Stage"() -> (w1630:enum16{"PI", "Steinmeyer"})
            n1178 = case shown="\"Steinmeyer\"" w1630 {
              tunnel: w1630 -> [w1637 w1646]
              frame "PI", Default {
                n1179 = local read "PIAxisID"() -> (w1633:string[])
                n1180 = local read "Stage Position"() -> (w1638:dbl)
                n1181 = call "RotateStage.vi"("Enum"=w1637, "Direction"=TRUE, "Stage max rotation"=365.0, "Stage position"=w1638, "Stage step size (deg)"=180.0, "PIAxisID"=w1633) -> ()  [unwired: 6 in]
                n1182 = call "PIEnablePositionDistanceTrigger.vi"("Start position"=360.0, "Displacement"=-720.0, "Trigger status"=TRUE) -> ()  [unwired: 7 in, 1 out]
              }
              frame "Steinmeyer" {
                n1183 = local read "PIAxisID"() -> (w1648:string[])
                n1184 = local read "Stage Position"() -> (w1647:dbl)
                n1185 = local read "Stage Acceleration (deg2/s)"() -> (w1645:dbl)
                n1186 = feedback #2() -> (w1640:bool)  [unwired: 1 in]
                n1187 = call "RotateStage.vi"("Acceleration"=w1645, "Enum"=w1646, "Velocity"=12.0, "Direction"=w1640, "Stage max rotation"=365.0, "Stage position"=w1647, "Stage step size (deg)"=20.0, "PIAxisID"=w1648) -> ()  [unwired: 4 in]
                n1188 = Not(x=w1640) -> (.not. x?=w1641:bool)
                n1189 = feedback-in #2(w1641) -> ()
              }
            }
          }
          event "Compress Avi": Mouse Down {
            n1190 = event-data() -> ()  [unwired: 1 in, 8 out]
            n1191 = Open VI Reference(vi path=path "F:/Development/labview software/CompressAVI/compressToAvi_v2.vi") -> (vi reference=w1656:refnum<vi>)  [unwired: 5 in, 1 out]
            n1192 = invoke class="VI" method="Run VI"(reference=w1656, "Wait until done"=FALSE ("Wait Until Done"), "Auto Dispose Ref"=TRUE ("Auto Dispose Reference")) -> (reference out=w1653:refnum<vi>)  [unwired: 2 in, 4 out]
            n1193 = invoke class="VI" method="FP.Open"(reference=w1653, "Activate"=TRUE ("Activate?"), "State"=T27."Standard") -> (reference out=w1650:refnum<vi>)  [unwired: 2 in, 4 out]
            n1194 = property class="VI"(reference=w1650, "Front Panel.IsFrontmost"=FALSE ("Front Panel Window:Is Frontmost")) -> ()  [unwired: 1 in, 2 out]
          }
          event "Wall connected": Value Change {
            n1195 = event-data() -> ("NewVal"=w1660:bool)  [unwired: 1 in, 5 out]
            n1196 = Open VI Reference(vi path=path "F:/Development/labview software/ActiveRotationExperiments/StepperMotorRotaryEncoderRecorder.vi") -> (vi reference=w1658:refnum<vi>)  [unwired: 5 in, 1 out]
            n1197 = case shown="True" w1660 {
              tunnel: w1658 -> [w1664 w1671]
              frame False {
                # "Stop VI if wall connection is aborted"
                n1198 = property class="VI"(reference=w1664) -> (reference out=w1662:refnum<vi>, "Exec.State"=w1663:T28)  [unwired: 1 in, 1 out]
                n1199 = case shown="\"Run top level\"" w1663 {
                  tunnel: w1662 -> [_ _ w1666 w1667]
                  frame "Bad", Default {
                  }
                  frame "Idle" {
                  }
                  frame "Run top level" {
                    n1200 = invoke class="VI" method="Abort VI"(reference=w1666) -> (reference out=w1665:refnum<vi>)  [unwired: 2 in, 2 out]
                    n1201 = invoke class="VI" method="FP.Close"(reference=w1665) -> ()  [unwired: 2 in, 3 out]
                  }
                  frame "Running" {
                    n1202 = invoke class="VI" method="Abort VI"(reference=w1667) -> ()  [unwired: 2 in, 3 out]
                  }
                }
              }
              frame True {
                # "Start rotary encoder data acquisition vi."
                n1203 = while {
                  tunnel: w1671 -> [w1672]
                  tunnel: [w1672] -> w1668
                  stop <- w1673 stop-if-true
                  n1204 = property class="VI"(reference=w1672) -> (reference out=w1675:refnum<vi>, "Exec.State"=w1676:T28)  [unwired: 1 in, 1 out]
                  n1205 = case shown="\"Idle\"" w1676 {
                    tunnel: w1675 -> [_ _ w1680]
                    tunnel: [FALSE TRUE FALSE] -> w1673
                    frame "Bad", Default {
                    }
                    frame "Idle" {
                    }
                    frame "Run top level", "Running" {
                      n1206 = invoke class="VI" method="Abort VI"(reference=w1680) -> ()  [unwired: 2 in, 3 out]
                    }
                  }
                  n1207 = Wait (ms)(milliseconds to wait=u32 100) -> ()  [unwired: 1 out]
                }
                n1208 = invoke class="VI" method="Run VI"(reference=w1668, "Wait until done"=FALSE ("Wait Until Done"), "Auto Dispose Ref"=TRUE ("Auto Dispose Reference")) -> ()  [unwired: 2 in, 5 out]
              }
            }
          }
          event "Release Air": Mouse Down {
            n1209 = event-data() -> ()  [unwired: 1 in, 8 out]
            n1210 = Unbundle By Name(w1682) -> ("Airpuff"=w1684:refnum<k21>)
            n1211 = call "SendTriggerPulse.vi"("Trigger Duration (ms)"=u32 60000, "Refnum in"=w1684) -> ("Refnum out"=w1683:refnum<k21>)  [unwired: 9 in]
            n1212 = Bundle By Name(cluster=w1682, "Airpuff"=w1683) -> (w1681:T26)
          }
          event "nTrials": Value Change {
            w1700 = 20.0 ("y")
            n1213 = event-data() -> ()  [unwired: 1 in, 6 out]
            n1214 = property on="Trial Performance" class="WFChart (strict)"() -> ("History Data"=w1698:cluster{"D'prime":dbl, "pCorrect":dbl}[])  [unwired: 2 in, 2 out]
            n1215 = local read "Mouse Performance"() -> (w1694:i16[][])
            n1216 = Array Size(array=w1698) -> (size(s)=w1696:i32)
            n1217 = local read "nTrials"() -> (w1697:i32)
            n1218 = Array Size(array=w1694) -> (size(s)=w1693:i32[])
            n1219 = local read "nTrials"() -> (w1690:i32)
            n1220 = Add(x=w1697, y=w1696) -> (x+y=w1695:i32)
            n1221 = Index Array(array=w1693, index=0) -> (element=w1689:i32)
            n1222 = Add(x=w1690, y=w1689) -> (x+y=w1691:i32)
            n1223 = To Double Precision Float(number=w1695) -> (double precision float=w1704:dbl)
            n1224 = Divide(x=w1704, y=w1700) -> (x/y=w1703:dbl)
            n1225 = To Double Precision Float(number=w1691) -> (double precision float=w1705:dbl)
            n1226 = Add(x=w1700, y=w1704) -> (x+y=w1702:dbl)
            n1227 = property on="Trial Performance" class="WFChart (strict)"("XScale.Increment"=w1703, "XScale.Maximum"=w1702, "XScale.Minimum"=20.0 ("X Scale.Range:Minimum")) -> ()  [unwired: 2 in, 2 out]
            n1228 = property on="Trial Outcomes" class="WFGraph (strict)"("XScale.Maximum"=w1705, "XScale.Minimum"=1.0 ("X Scale.Range:Minimum")) -> ()  [unwired: 2 in, 2 out]
            n1229 = property on="Trial Performance" class="WFChart (strict)"("XScale.Multiplier"=1.0 ("X Scale.Offset and Multiplier:Multiplier"), "XScale.Offset"=w1700) -> ()  [unwired: 2 in, 2 out]
          }
          event "Print Screen": Value Change {
            n1230 = event-data() -> ("Source"=→"Source":T4, "NewVal"=w1710:bool)  [unwired: 1 in, 4 out]
            n1231 = case shown="True" w1710 {
              frame False {
              }
              frame True {
                n1232 = flat-sequence {
                  frame #0 {
                    n1233 = property on="Print Screen" class="Bool (strict)"("Visible"=FALSE) -> ()  [unwired: 2 in, 2 out]
                  }
                  frame #1 {
                    n1234 = local read "ImageSummaryPath"() -> (w1712:path)
                    n1235 = Current VI's Path() -> (path=w1713:path)
                    n1236 = call "SaveFrontPanel.vi"("path to PNG file"=w1712, "vi path"=w1713) -> ()  [unwired: 10 in]
                  }
                  frame #2 {
                    n1237 = local write "Print Screen"(FALSE ("Print Screen")) -> ()
                    n1238 = property on="Print Screen" class="Bool (strict)"("Visible"=TRUE) -> ()  [unwired: 2 in, 2 out]
                  }
                }
              }
            }
          }
          event "BtnStageMoveHome", "Home": Mouse Down {
            n1239 = event-data() -> ()  [unwired: 1 in, 8 out]
            n1240 = local read "Select Rotation Stage"() -> (w1718:enum16{"PI", "Steinmeyer"})
            n1241 = case shown="\"Steinmeyer\"" w1718 {
              frame "PI", Default {
                n1242 = local read "PIAxisID"() -> (w1720:string[])
                n1243 = call "PIMoveAbsolute.vi"("To position"=0.0, "AxisID"=w1720) -> ()  [unwired: 9 in, 1 out]
              }
              frame "Steinmeyer" {
                n1244 = call "SMMoveAbsolute.vi"() -> ()  [unwired: 12 in]
              }
            }
          }
          event "Move to ...": Value Change {
            n1245 = event-data() -> ()  [unwired: 1 in, 6 out]
            n1246 = call "SMMoveAbsolute.vi"("Acceleration"=200.0, "Speed"=45.0, "Displacement"="... Position") -> ()  [unwired: 9 in]
          }
          event "BtnStageStepCW", "Step-": Mouse Down {
            n1247 = event-data() -> ()  [unwired: 1 in, 8 out]
            n1248 = local read "Select Rotation Stage"() -> (w1728:enum16{"PI", "Steinmeyer"})
            n1249 = case shown="\"Steinmeyer\"" w1728 {
              tunnel: w1728 -> [w1734 w1741]
              frame "PI", Default {
                n1250 = local read "PIAxisID"() -> (w1730:string[])
                n1251 = local read "Stage step size (deg)"() -> (w1737:dbl)
                n1252 = local read "Stage Position"() -> (w1735:dbl)
                n1253 = call "PIEnablePositionDistanceTrigger.vi"("Start position"=360.0, "Displacement"=-720.0, "Trigger status"=TRUE) -> ()  [unwired: 7 in, 1 out]
                n1254 = call "RotateStage.vi"("Enum"=w1734, "Direction"=FALSE, "Stage max rotation"=365.0, "Stage position"=w1735, "Stage step size (deg)"=w1737, "PIAxisID"=w1730) -> ()  [unwired: 6 in]
              }
              frame "Steinmeyer" {
                n1255 = local read "PIAxisID"() -> (w1745:string[])
                n1256 = local read "Stage step size (deg)"() -> (w1744:dbl)
                n1257 = local read "Stage Position"() -> (w1742:dbl)
                n1258 = local read "Stage Speed (deg/s)"() -> (w1740:dbl)
                n1259 = local read "Stage Acceleration (deg2/s)"() -> (w1739:dbl)
                n1260 = call "RotateStage.vi"("Acceleration"=w1739, "Enum"=w1741, "Velocity"=w1740, "Direction"=FALSE, "Stage max rotation"=365.0, "Stage position"=w1742, "Stage step size (deg)"=w1744, "PIAxisID"=w1745) -> ()  [unwired: 4 in]
              }
            }
          }
          event "BtnStageStepCCW", "Step+": Mouse Down {
            n1261 = event-data() -> ()  [unwired: 1 in, 8 out]
            n1262 = local read "Select Rotation Stage"() -> (w1748:enum16{"PI", "Steinmeyer"})
            n1263 = case shown="\"Steinmeyer\"" w1748 {
              tunnel: w1748 -> [w1754 w1761]
              frame "PI", Default {
                n1264 = local read "PIAxisID"() -> (w1750:string[])
                n1265 = local read "Stage step size (deg)"() -> (w1757:dbl)
                n1266 = local read "Stage Position"() -> (w1755:dbl)
                n1267 = call "RotateStage.vi"("Enum"=w1754, "Direction"=TRUE, "Stage max rotation"=365.0, "Stage position"=w1755, "Stage step size (deg)"=w1757, "PIAxisID"=w1750) -> ()  [unwired: 6 in]
                n1268 = call "PIEnablePositionDistanceTrigger.vi"("Start position"=360.0, "Displacement"=-720.0, "Trigger status"=TRUE) -> ()  [unwired: 7 in, 1 out]
              }
              frame "Steinmeyer" {
                n1269 = local read "PIAxisID"() -> (w1765:string[])
                n1270 = local read "Stage step size (deg)"() -> (w1764:dbl)
                n1271 = local read "Stage Position"() -> (w1762:dbl)
                n1272 = local read "Stage Speed (deg/s)"() -> (w1760:dbl)
                n1273 = local read "Stage Acceleration (deg2/s)"() -> (w1759:dbl)
                n1274 = call "RotateStage.vi"("Acceleration"=w1759, "Enum"=w1761, "Velocity"=w1760, "Direction"=TRUE, "Stage max rotation"=365.0, "Stage position"=w1762, "Stage step size (deg)"=w1764, "PIAxisID"=w1765) -> ()  [unwired: 4 in]
              }
            }
          }
          event "BtnStage180CCW": Mouse Down {
            n1275 = event-data() -> ()  [unwired: 1 in, 8 out]
            n1276 = local read "Select Rotation Stage"() -> (w1768:enum16{"PI", "Steinmeyer"})
            n1277 = case shown="\"Steinmeyer\"" w1768 {
              tunnel: w1768 -> [w1775 w1782]
              frame "PI", Default {
                n1278 = local read "PIAxisID"() -> (w1771:string[])
                n1279 = local read "Stage Position"() -> (w1776:dbl)
                n1280 = call "RotateStage.vi"("Enum"=w1775, "Direction"=TRUE, "Stage max rotation"=365.0, "Stage position"=w1776, "Stage step size (deg)"=180.0, "PIAxisID"=w1771) -> ()  [unwired: 6 in]
                n1281 = call "PIEnablePositionDistanceTrigger.vi"("Start position"=360.0, "Displacement"=-720.0, "Trigger status"=TRUE) -> ()  [unwired: 7 in, 1 out]
              }
              frame "Steinmeyer" {
                n1282 = local read "PIAxisID"() -> (w1785:string[])
                n1283 = local read "Stage Position"() -> (w1783:dbl)
                n1284 = local read "Stage Speed (deg/s)"() -> (w1781:dbl)
                n1285 = local read "Stage Acceleration (deg2/s)"() -> (w1780:dbl)
                n1286 = call "RotateStage.vi"("Acceleration"=w1780, "Enum"=w1782, "Velocity"=w1781, "Direction"=TRUE, "Stage max rotation"=365.0, "Stage position"=w1783, "Stage step size (deg)"=180.0, "PIAxisID"=w1785) -> ()  [unwired: 4 in]
              }
            }
          }
          event "BtnStage180CW": Mouse Down {
            n1287 = event-data() -> ()  [unwired: 1 in, 8 out]
            n1288 = local read "Select Rotation Stage"() -> (w1788:enum16{"PI", "Steinmeyer"})
            n1289 = case shown="\"Steinmeyer\"" w1788 {
              tunnel: w1788 -> [w1795 w1802]
              frame "PI", Default {
                n1290 = local read "PIAxisID"() -> (w1791:string[])
                n1291 = local read "Stage Position"() -> (w1796:dbl)
                n1292 = call "RotateStage.vi"("Enum"=w1795, "Direction"=FALSE, "Stage max rotation"=365.0, "Stage position"=w1796, "Stage step size (deg)"=180.0, "PIAxisID"=w1791) -> ()  [unwired: 6 in]
                n1293 = call "PIEnablePositionDistanceTrigger.vi"("Start position"=360.0, "Displacement"=-720.0, "Trigger status"=TRUE) -> ()  [unwired: 7 in, 1 out]
              }
              frame "Steinmeyer" {
                n1294 = local read "PIAxisID"() -> (w1805:string[])
                n1295 = local read "Stage Position"() -> (w1803:dbl)
                n1296 = local read "Stage Speed (deg/s)"() -> (w1801:dbl)
                n1297 = local read "Stage Acceleration (deg2/s)"() -> (w1800:dbl)
                n1298 = call "RotateStage.vi"("Acceleration"=w1800, "Enum"=w1802, "Velocity"=w1801, "Direction"=FALSE, "Stage max rotation"=365.0, "Stage position"=w1803, "Stage step size (deg)"=180.0, "PIAxisID"=w1805) -> ()  [unwired: 4 in]
              }
            }
          }
          event "Response Timeout": Value Change {
            n1299 = event-data() -> ("NewVal"=w1808:bool)  [unwired: 1 in, 5 out]
            n1300 = case shown="True" w1808 {
              frame False {
                (unwired) FALSE
              }
              frame True {
                w1815 = nan
                n1301 = local read "AllowReward"() -> (w1813:bool)
                n1302 = local read "Response Times"() -> (w1823:dbl[])
                n1303 = Select(t=TRUE, s=w1813, f=FALSE) -> (s? t:f=w1816:bool)
                n1304 = Select(t=FALSE ("f"), s=w1813, f=TRUE) -> (s? t:f=w1819:bool)
                n1305 = local write "Miss"(w1816) -> ()
                n1306 = local write "Correct Rejection"(w1819) -> ()
                n1307 = Select(t=FALSE ("f"), s=w1813, f=FALSE) -> (s? t:f=w1809:bool)
                n1308 = Build Array (concatenate)(w1823, w1815) -> (w1822:dbl[])
                n1309 = local write "AllowReward"(w1809) -> ()
                n1310 = local write "last response time (ms)"(w1815) -> ()
                n1311 = local write "Response Times"(w1822) -> ()
                n1312 = local write "response window is open"(w1809) -> ()
                n1313 = local write "Response Timeout"(FALSE ("Response Timeout")) -> ()
                n1314 = local write "Waiting for lick"(FALSE ("Waiting for response")) -> ()
              }
            }
          }
          event "SS Crash Button": Value Change {
            n1315 = event-data() -> ("NewVal"=w1827:bool)  [unwired: 1 in, 5 out]
            n1316 = case shown="True" w1827 {
              selector: w1827 -> [w1828 _]
              tunnel: [w1828 FALSE] -> w1826
              frame False {
              }
              frame True {
                n1317 = local read "Session Checklist"() -> (w1830:T2)
                n1318 = Bundle By Name(cluster=w1830, "PMT Gain"=FALSE ("Security Camera"), "Laser Power"=FALSE ("Lickport In Place")) -> (w1829:T2)
                n1319 = local write "Session Checklist"(w1829) -> ()
              }
            }
            n1320 = local write "SS Crash Button"(w1826) -> ()
          }
          event "Give Water": Value Change {
            n1321 = event-data() -> ("NewVal"=w1839:bool)  [unwired: 1 in, 5 out]
            n1322 = Unbundle By Name(w1835) -> ("Water Valve"=w1837:refnum<k21>)
            n1323 = case shown="True" w1839 {
              tunnel: [w1840 w1855] -> w1836
              tunnel: w1837 -> [w1840 w1851]
              frame False {
              }
              frame True {
                n1324 = local read "Valve opening time (ms)"() -> (w1845:u32)
                n1325 = local read "NRewards"() -> (w1854:i32)
                n1326 = Increment(x=w1854) -> (x+1=w1852:i32)
                n1327 = local write "NRewards"(w1852) -> ()
                n1328 = Divide(x=w1845, y=u32 2) -> (x/y=w1843:dbl)
                n1329 = Round To Nearest(number=w1843) -> (nearest integer value=w1842:dbl)
                n1330 = local read "mL Per Ms"() -> (w1853:dbl)
                n1331 = call "SendTriggerPulse.vi"("Trigger Duration (ms)"=w1842, "Refnum in"=w1851) -> ("Refnum out"=w1855:refnum<k21>)  [unwired: 9 in]
                n1332 = To Double Precision Float(number=w1842) -> (double precision float=w1848:dbl)
                n1333 = local read "mL given"() -> (w1846:dbl)
                n1334 = Multiply(x=w1853, y=w1848) -> (x*y=w1847:dbl)
                n1335 = local write "AllowReward"(FALSE ("AllowReward")) -> ()
                n1336 = Add(x=w1846, y=w1847) -> (x+y=w1849:dbl)
                n1337 = local write "Give Water"(FALSE ("Give Water")) -> ()
                n1338 = local write "mL given"(w1849) -> ()
              }
            }
            n1339 = Bundle By Name(cluster=w1835, "Water Valve"=w1836) -> (w1834:T26)
          }
          event "BtnBothCCW": Value Change {
            n1340 = event-data() -> ()  [unwired: 1 in, 6 out]
            n1341 = local read "StepperController.lvclass"() -> (w1863:refnum<class "StepperController.lvclass">)
            n1342 = local read "Wall Moving?"() -> (w1864:bool)
            n1343 = case shown="False" w1864 {
              selector: w1864 -> [_ w1904]
              tunnel: w1863 -> [w1901 _]
              tunnel: [w1898 w1904] -> w1862
              tunnel: [w1897 0.0 ("AmountMoved")] -> w1859
              tunnel: [w1896 u32 0 ("millisecond timer value")] -> w1856
              frame False {
                n1344 = Tick Count (ms)() -> (millisecond timer value=w1896:u32)
                n1345 = call "Rotate.vi"("Direction"=FALSE, "StepperController in"=w1901) -> ("NewPosition"=w1899:dbl, "DidMove"=w1898:bool, "StepperController out"=w1895:refnum<class "StepperController.lvclass">, "AmountMoved"=w1897:dbl)  [unwired: 5 in, 1 out]
                n1346 = local write "Wall Position"(w1899) -> ()
                n1347 = local write "StepperController.lvclass"(w1895) -> ()
              }
              frame True {
              }
            }
            n1348 = while {
              tunnel: w1858 -> [w1871]
              tunnel: [w1871] -> w1857
              tunnel: w1856 -> [w1869]
              stop <- w1866 stop-if-true
              n1349 = Tick Count (ms)() -> (millisecond timer value=w1870:u32)
              n1350 = local read "Wall-Stage delay (ms)"() -> (w1867:dbl)
              n1351 = Subtract(x=w1870, y=w1869) -> (x-y=w1868:u32)
              n1352 = Greater?(x=w1868, y=w1867) -> (0:w1866:bool)
              n1353 = Wait (ms)(milliseconds to wait=u32 1) -> ()  [unwired: 1 out]
            }
            n1354 = local read "Select Rotation Stage"() -> (w1861:enum16{"PI", "Steinmeyer"})
            n1355 = flat-sequence {
              tunnel: [w1892] -> w1865
              tunnel: w1862 -> [w1892]
              tunnel: [w1891] -> w1860
              tunnel: w1859 -> [w1891]
              tunnel: w1865 -> [w1894]
              tunnel: w1860 -> [w1893]
              tunnel: [w1893] -> w1858
              frame #0 {
                n1356 = Wait (ms)(milliseconds to wait=u32 10) -> ()  [unwired: 1 out]
              }
              frame #1 {
                n1357 = local write "Wall Moving?"(w1894) -> ()
              }
            }
            n1358 = case shown="\"Steinmeyer\"" w1861 {
              tunnel: w1861 -> [w1878 w1886]
              tunnel: w1857 -> [_ w1882]
              frame "PI", Default {
                n1359 = local read "PIAxisID"() -> (w1874:string[])
                n1360 = local read "Stage step size (deg)"() -> (w1881:dbl)
                n1361 = local read "Stage Position"() -> (w1879:dbl)
                n1362 = call "RotateStage.vi"("Enum"=w1878, "Direction"=FALSE, "Stage max rotation"=365.0, "Stage position"=w1879, "Stage step size (deg)"=w1881, "PIAxisID"=w1874) -> ()  [unwired: 6 in]
                n1363 = call "PIEnablePositionDistanceTrigger.vi"("Start position"=360.0, "Displacement"=-720.0, "Trigger status"=TRUE) -> ()  [unwired: 7 in, 1 out]
              }
              frame "Steinmeyer" {
                n1364 = local read "PIAxisID"() -> (w1889:string[])
                n1365 = local read "Stage Position"() -> (w1887:dbl)
                n1366 = local read "Wall Speed (deg/s)"() -> (w1885:dbl)
                n1367 = local read "Wall Acceleration (deg2/s)"() -> (w1884:dbl)
                n1368 = call "RotateStage.vi"("Acceleration"=w1884, "Enum"=w1886, "Velocity"=w1885, "Direction"=FALSE, "Stage max rotation"=365.0, "Stage position"=w1887, "Stage step size (deg)"=w1882, "PIAxisID"=w1889) -> ()  [unwired: 4 in]
              }
            }
          }
          event "BtnBothCW": Value Change {
            n1369 = event-data() -> ()  [unwired: 1 in, 6 out]
          }
          event "Mouse Entered": Value Change {
            n1370 = event-data() -> ("NewVal"=w1907:bool)  [unwired: 1 in, 5 out]
            n1371 = case shown="True" w1907 {
              frame False {
              }
              frame True {
                w1917 = 1 ("Recording No")
                n1372 = Get Date/Time In Seconds() -> (seconds since 1Jan1904=w1931:timestamp)
                n1373 = Format Into String(format string="-%03d" ("initial string"), w1917) -> (resulting string=w1929:string)  [unwired: 2 in, 1 out]
                n1374 = Format Into String(format string="m%04d-" ("initial string"), "Mouse Number") -> (resulting string=w1923:string)  [unwired: 2 in, 1 out]
                n1375 = Format Date/Time String(time format string (%c)="%Y%m%d-%H%M", seconds (now)=w1931) -> (date/time string=w1920:string)  [unwired: 1 in]
                "RecordingID" <- w1920
                n1376 = Concatenate Strings(w1923, w1920, w1929) -> (w1919:string)
                "SessionID" <- w1919
                n1377 = local write "Mouse entered arena"(w1920) -> ()
                n1378 = local write "Recording No"(w1917) -> ()
                n1379 = global write "GlobalVariables.vi" "SessionID"(w1919) -> ()
                n1380 = invoke on="mL given" class="Slide (strict)" method="Reinit To Default"() -> ()  [unwired: 3 in, 3 out]
                n1381 = local read "Session Checklist"() -> (w1913:T2)
                n1382 = invoke on="Mouse Performance" class="Arr (strict)" method="Reinit To Default"() -> ()  [unwired: 3 in, 3 out]
                n1383 = local write "NRewards"(0 ("NRewards")) -> ()
                n1384 = local write "NGoTrials"(0 ("NGoTrials")) -> ()
                n1385 = Bundle By Name(cluster=w1913, "Security Camera"=FALSE, "Lickport In Place"=FALSE, "Pupil Camera"=FALSE, "Pupil Cropped"=FALSE, "Training Day"=FALSE, "Lickport In Place"=FALSE, "Wall In Place"=FALSE) -> (w1914:T2)
                n1386 = case shown="True" FALSE {
                  frame False {
                  }
                  frame True {
                    n1387 = local write "mL given"(0.0 ("mL given")) -> ()
                  }
                }
                n1388 = invoke on="Trial Outcomes" class="WFGraph (strict)" method="Reinit To Default"() -> ()  [unwired: 3 in, 3 out]
                n1389 = property on="Trial Performance" class="WFChart (strict)"("History Data"=cluster{dbl, dbl}[] []) -> ()  [unwired: 2 in, 2 out]
                n1390 = local write "Session Checklist"(w1914) -> ()
                "nCorrect" <- 0 ("nCorrect")
                "tmpNCorrect" <- 0 ("tmpNCorrect")
              }
            }
          }
          event "Recording No": Value Change {
            n1391 = event-data() -> ("NewVal"=w1934:i32)  [unwired: 1 in, 5 out]
            n1392 = local read "Mouse Number"() -> (w1939:i32)
            n1393 = local read "RecordingID"() -> (w1937:string)
            n1394 = Format Into String(format string="-%03d" ("initial string"), w1934) -> (resulting string=w1935:string)  [unwired: 2 in, 1 out]
            n1395 = Format Into String(format string="m%04d-" ("initial string"), w1939) -> (resulting string=w1940:string)  [unwired: 2 in, 1 out]
            n1396 = Concatenate Strings(w1940, w1937, w1935) -> (w1941:string)
            n1397 = global write "GlobalVariables.vi" "SessionID"(w1941) -> ()
            n1398 = local write "SessionID"(w1941) -> ()
          }
          event "BtnWallSetHome": Mouse Down {
            n1399 = event-data() -> ()  [unwired: 1 in, 8 out]
            n1400 = local read "StepperController.lvclass"() -> (w1945:refnum<class "StepperController.lvclass">)
            n1401 = local write "Wall Position"(0.0 ("Wall Position")) -> ()
            n1402 = call "SetHome.vi"("StepperController in"=w1945) -> ("StepperController out"=w1946:refnum<class "StepperController.lvclass">)  [unwired: 1 in, 1 out]
            n1403 = local write "StepperController.lvclass"(w1946) -> ()
          }
          event "BtnWallMoveHome": Value Change {
            n1404 = event-data() -> ("NewVal"=w1948:bool)  [unwired: 1 in, 5 out]
            n1405 = case shown="True" w1948 {
              frame False {
              }
              frame True {
                n1406 = local read "StepperController.lvclass"() -> (w1956:refnum<class "StepperController.lvclass">)
                n1407 = local read "Wall Position"() -> (w1953:dbl)
                n1408 = Absolute Value(x=w1953) -> (abs(x)=w1954:dbl)
                n1409 = Greater?(x=w1954, y=2.0) -> (0:w1952:bool)
                n1410 = case shown="True" w1952 {
                  tunnel: w1953 -> [_ w1966]
                  tunnel: w1956 -> [w1957 w1965]
                  tunnel: [w1957 w1958] -> w1951
                  frame False {
                  }
                  frame True {
                    n1411 = local read "Wall Speed (deg/s)"() -> (w1968:dbl)
                    n1412 = local read "Wall Acceleration (deg2/s)"() -> (w1967:dbl)
                    n1413 = Greater?(x=w1966, y=0.0) -> (0:w1962:bool)
                    n1414 = Absolute Value(x=w1966) -> (abs(x)=w1960:dbl)
                    n1415 = call-dynamic "PrepareRotation.vi"("Rotate amount"=w1960, "Acceleration (deg2/s)"=w1967, "Speed (deg/s)"=w1968, "StepperController in"=w1965) -> ("error out"=w1959:errorcluster, "StepperController out"=w1961:refnum<class "StepperController.lvclass">)  [unwired: 5 in, 1 out]
                    n1416 = call "Rotate.vi"("error in (no error)"=w1959, "Direction"=w1962, "StepperController in"=w1961) -> ("NewPosition"=w1963:dbl, "DidMove"=w1964:bool, "StepperController out"=w1958:refnum<class "StepperController.lvclass">)  [unwired: 4 in, 2 out]
                    n1417 = local write "Wall Moving?"(w1964) -> ()
                    n1418 = local write "Wall Position"(w1963) -> ()
                  }
                }
                n1419 = local write "StepperController.lvclass"(w1951) -> ()
                n1420 = local write "BtnWallMoveHome"(FALSE ("BtnWallMoveHome")) -> ()
              }
            }
          }
          event "BtnWallStepCCW": Mouse Down {
            n1421 = event-data() -> ()  [unwired: 1 in, 8 out]
            n1422 = local read "StepperController.lvclass"() -> (w1975:refnum<class "StepperController.lvclass">)
            n1423 = local read "Wall Moving?"() -> (w1976:bool)
            n1424 = case shown="False" w1976 {
              selector: w1976 -> [_ w1985]
              tunnel: w1975 -> [w1984 w1986]
              tunnel: [w1981 w1986] -> w1974
              tunnel: [w1980 w1985] -> w1972
              frame False {
                n1425 = call "Rotate.vi"("Direction"=TRUE, "StepperController in"=w1984) -> ("NewPosition"=w1982:dbl, "DidMove"=w1980:bool, "StepperController out"=w1981:refnum<class "StepperController.lvclass">)  [unwired: 5 in, 2 out]
                n1426 = local write "Wall Position"(w1982) -> ()
              }
              frame True {
              }
            }
            n1427 = flat-sequence {
              tunnel: w1974 -> [w1978]
              tunnel: [w1977] -> w1973
              tunnel: w1972 -> [w1977]
              tunnel: w1973 -> [w1979]
              frame #0 {
                n1428 = local write "StepperController.lvclass"(w1978) -> ()
              }
              frame #1 {
                n1429 = local write "Wall Moving?"(w1979) -> ()
              }
            }
          }
          event "Wall Speed (deg/s)", "Wall Acceleration (deg2/s)", "Wall step size (deg)": Value Change {
            n1430 = event-data() -> ()  [unwired: 1 in, 6 out]
            n1431 = local read "Wall step size (deg)"() -> (w1991:dbl)
            n1432 = local read "StepperController.lvclass"() -> (w1993:refnum<class "StepperController.lvclass">)
            n1433 = local read "Wall Speed (deg/s)"() -> (w1990:dbl)
            n1434 = local read "Wall Acceleration (deg2/s)"() -> (w1989:dbl)
            n1435 = call-dynamic "PrepareRotation.vi"("Rotate amount"=w1991, "Acceleration (deg2/s)"=w1989, "Speed (deg/s)"=w1990, "StepperController in"=w1993) -> ("StepperController out"=w1992:refnum<class "StepperController.lvclass">)  [unwired: 5 in, 2 out]
            n1436 = local write "StepperController.lvclass"(w1992) -> ()
          }
          event "Wall physical step size (deg/step)", "Wall max rotation": Value Change {
            n1437 = event-data() -> ()  [unwired: 1 in, 6 out]
            n1438 = local read "StepperController.lvclass"() -> (w1998:refnum<class "StepperController.lvclass">)
            n1439 = local read "Wall physical step size (deg/step)"() -> (w2000:dbl)
            n1440 = local read "Wall max rotation"() -> (w1999:dbl)
            n1441 = call-dynamic "Init.vi"("MaxRotation"=w1999, "PhysicalStepSize"=w2000, "StepperController in"=w1998) -> ("StepperController out"=w1995:refnum<class "StepperController.lvclass">)  [unwired: 7 in, 1 out]
            n1442 = local write "StepperController.lvclass"(w1995) -> ()
            n1443 = local write "Stepper Prepared for Rotation"(FALSE ("Stepper Prepared for Rotation")) -> ()
          }
          event "BtnWallStepCW": Mouse Down {
            n1444 = event-data() -> ()  [unwired: 1 in, 8 out]
            n1445 = local read "StepperController.lvclass"() -> (w2006:refnum<class "StepperController.lvclass">)
            n1446 = local read "Wall Moving?"() -> (w2007:bool)
            n1447 = case shown="False" w2007 {
              selector: w2007 -> [_ w2016]
              tunnel: w2006 -> [w2015 w2017]
              tunnel: [w2012 w2017] -> w2004
              tunnel: [w2011 w2016] -> w2003
              frame False {
                n1448 = call "Rotate.vi"("Direction"=FALSE, "StepperController in"=w2015) -> ("NewPosition"=w2013:dbl, "DidMove"=w2011:bool, "StepperController out"=w2012:refnum<class "StepperController.lvclass">)  [unwired: 5 in, 2 out]
                n1449 = local write "Wall Position"(w2013) -> ()
              }
              frame True {
              }
            }
            n1450 = flat-sequence {
              tunnel: w2004 -> [w2009]
              tunnel: [w2008] -> w2005
              tunnel: w2003 -> [w2008]
              tunnel: w2005 -> [w2010]
              frame #0 {
                n1451 = local write "StepperController.lvclass"(w2009) -> ()
              }
              frame #1 {
                n1452 = local write "Wall Moving?"(w2010) -> ()
              }
            }
          }
          event "Airpuff": Value Change {
            n1453 = event-data() -> ("NewVal"=w2023:bool)  [unwired: 1 in, 5 out]
            n1454 = Unbundle By Name(w2020) -> ("Airpuff"=w2021:refnum<k21>)
            n1455 = case shown="False" w2023 {
              tunnel: [w2024 w2030] -> w2019
              tunnel: w2021 -> [w2024 w2025]
              frame False {
              }
              frame True {
                n1456 = local read "NPunishments"() -> (w2028:i32)
                n1457 = Increment(x=w2028) -> (x+1=w2027:i32)
                n1458 = call "SendTriggerPulse.vi"("Trigger Duration (ms)"="Airpuff (ms)", "Refnum in"=w2025) -> ("Refnum out"=w2030:refnum<k21>)  [unwired: 9 in]
                n1459 = local write "NPunishments"(w2027) -> ()
                n1460 = local write "Airpuff"(FALSE ("Airpuff")) -> ()
              }
            }
            n1461 = Bundle By Name(cluster=w2020, "Airpuff"=w2019) -> (w2018:T26)
          }
          event "Open Valve": Value Change {
            n1462 = event-data() -> ("NewVal"=w2036:bool)  [unwired: 1 in, 5 out]
            n1463 = Unbundle By Name(w2033) -> ("Water Valve"=w2034:refnum<k21>)
            n1464 = call <vilib>:"DAQmx Start Task.vi"("task/channels in"=w2034) -> ("task out"=w2038:refnum<k21>)  [unwired: 13 in, 1 out]
            n1465 = call-poly <vilib>:"DAQmx Write.vi"("task/channels in"=w2038, "data"=w2036) -> ("task out"=w2037:refnum<k21>)  [unwired: 11 in, 2 out]
            n1466 = call <vilib>:"DAQmx Stop Task.vi"("task/channels in"=w2037) -> ("task out"=w2031:refnum<k21>)  [unwired: 13 in, 1 out]
            n1467 = Bundle By Name(cluster=w2033, "Water Valve"=w2031) -> (w2032:T26)
          }
          event "Reward Green Light": Value Change {
            n1468 = event-data() -> ("NewVal"=w2041:bool)  [unwired: 1 in, 5 out]
            n1469 = case shown="True" w2041 {
              frame False {
              }
              frame True {
                n1470 = local write "response window is open"(TRUE ("response window is open")) -> ()
                n1471 = local write "Waiting for lick"(TRUE ("Green Light")) -> ()
                n1472 = local write "Licked"(FALSE) -> ()
                n1473 = Tick Count (ms)() -> (millisecond timer value=w2046:u32)
                n1474 = local write "Reward Green Light"(FALSE ("NoBeep (GreenLight)")) -> ()
                n1475 = local write "cue time"(w2046) -> ()
              }
            }
          }
          event "Reset": Value Change {
            n1476 = event-data() -> ("NewVal"=w2049:bool)  [unwired: 1 in, 5 out]
            n1477 = case shown="True" w2049 {
              frame False {
              }
              frame True {
                n1478 = invoke on="NPunishments" class="DigNum (strict)" method="Reinit To Default"() -> ()  [unwired: 3 in, 3 out]
                n1479 = invoke on="NRewards" class="DigNum (strict)" method="Reinit To Default"() -> ()  [unwired: 3 in, 3 out]
                n1480 = invoke on="NGoTrials" class="DigNum (strict)" method="Reinit To Default"() -> ()  [unwired: 3 in, 3 out]
                n1481 = local write "Last Image number SV"(u32 0 ("Last Image number SV")) -> ()
                n1482 = local write "Reset Lost Frames"(TRUE ("Reset Lost Frames")) -> ()
                n1483 = invoke on="Trial Counter" class="DigNum (strict)" method="Reinit To Default"() -> ()  [unwired: 3 in, 3 out]
                n1484 = invoke on="Mouse Performance" class="Arr (strict)" method="Reinit To Default"() -> ()  [unwired: 3 in, 3 out]
                n1485 = disable-structure shown="Disabled" {
                  frame Disabled {
                    n1486 = invoke on="NLicks" class="Arr (strict)" method="Reinit To Default"() -> ()  [unwired: 3 in, 3 out]
                  }
                  frame Enabled {
                  }
                }
                n1487 = invoke on="Lick Rates" class="WFGraph (strict)" method="Reinit To Default"() -> ()  [unwired: 3 in, 3 out]
                n1488 = invoke on="LickPerMin" class="Arr (strict)" method="Reinit To Default"() -> ()  [unwired: 3 in, 3 out]
                n1489 = local write "NLicks"(i32[] [0, 0, 0] ("NLicks")) -> ()
                n1490 = invoke on="Trial Outcomes" class="WFGraph (strict)" method="Reinit To Default"() -> ()  [unwired: 3 in, 3 out]
                n1491 = invoke on="d'" class="DigNum (strict)" method="Reinit To Default"() -> ()  [unwired: 3 in, 3 out]
                n1492 = invoke on="% correct" class="DigNum (strict)" method="Reinit To Default"() -> ()  [unwired: 3 in, 3 out]
                n1493 = local write "Reset"(FALSE ("Reset")) -> ()
                n1494 = invoke on="Current trial" class="Str" method="Reinit To Default"() -> ()  [unwired: 3 in, 3 out]
                n1495 = invoke on="Trial Performance" class="WFChart (strict)" method="Reinit To Default"() -> ()  [unwired: 3 in, 3 out]
                n1496 = property on="Trial Performance" class="WFChart (strict)"("History Data"=cluster{dbl, dbl}[] []) -> ()  [unwired: 2 in, 2 out]
              }
            }
          }
          event "Lights On": Value Change {
            n1497 = event-data() -> ("NewVal"=w2062:bool)  [unwired: 1 in, 5 out]
            n1498 = Unbundle By Name(w2057) -> ("Light Switch"=w2058:refnum<k21>)
            n1499 = call <vilib>:"DAQmx Start Task.vi"("task/channels in"=w2058) -> ("task out"=w2060:refnum<k21>)  [unwired: 13 in, 1 out]
            n1500 = call-poly <vilib>:"DAQmx Write.vi"("task/channels in"=w2060, "data"=w2062) -> ("task out"=w2061:refnum<k21>)  [unwired: 11 in, 2 out]
            n1501 = call <vilib>:"DAQmx Stop Task.vi"("task/channels in"=w2061) -> ("task out"=w2056:refnum<k21>)  [unwired: 13 in, 1 out]
            n1502 = Bundle By Name(cluster=w2057, "Light Switch"=w2056) -> (w2055:T26)
          }
          event "Licked": Value Change {
            n1503 = event-data() -> ()  [unwired: 1 in, 6 out]
            n1504 = local read "Reward Mode"() -> (w2075:enum16{"Reward on Cue", "Reward on Lick"})
            n1505 = local read "AllowReward"() -> (w2076:bool)
            n1506 = Unbundle By Name(w2065) -> ("Water Valve"=w2066:refnum<k21>)
            n1507 = case shown="True" w2076 {
              tunnel: [w2077 w2097] -> w2063
              tunnel: w2075 -> [_ w2102]
              tunnel: [FALSE FALSE] -> w2068
              tunnel: w2066 -> [w2077 w2098]
              frame False {
                n1508 = local read "NRewards"() -> (w2088:i32)
                n1509 = local read "NPunishments"() -> (w2087:i32)
                n1510 = Divide(x=w2088, y=w2087) -> (x/y=w2086:dbl)
                n1511 = local write "False Alarm"(TRUE ("FalseGo")) -> ()
                n1512 = Random Number (0-1)() -> (number: 0 to 1=w2085:dbl)
                n1513 = Greater?(x=w2085, y=0.5) -> (0:w2082:bool)
                n1514 = Greater Or Equal?(x=w2086, y="Reward Punishment Ratio") -> (x >= y?=w2083:bool)
                n1515 = And(x=w2082, y=w2083) -> (x .and. y?=w2080:bool)
                n1516 = Or(x="Always Puff", y=w2080) -> (x .or. y?=w2079:bool)
                n1517 = property on="Airpuff" class="Bool (strict)"("Val(Sgnl)"=w2079) -> ()  [unwired: 2 in, 2 out]
              }
              frame True {
                n1518 = local read "NRewards"() -> (w2104:i32)
                n1519 = case shown="\"Reward on Cue\", Default" w2102 {
                  tunnel: [w2107 w2110] -> w2097
                  tunnel: w2098 -> [w2106 w2109]
                  tunnel: [w2105 w2108] -> w2091
                  frame "Reward on Cue", Default {
                    n1520 = local read "Valve opening time (ms)"() -> (w2105:u32)
                    n1521 = call "SendTriggerPulse.vi"("Trigger Duration (ms)"=w2105, "Refnum in"=w2106) -> ("Refnum out"=w2107:refnum<k21>)  [unwired: 9 in]
                  }
                  frame "Reward on Lick" {
                    n1522 = local read "Valve opening time (ms)"() -> (w2108:u32)
                    n1523 = call "SendTriggerPulse.vi"("Trigger Duration (ms)"=w2108, "Refnum in"=w2109) -> ("Refnum out"=w2110:refnum<k21>)  [unwired: 9 in]
                  }
                }
                n1524 = Increment(x=w2104) -> (x+1=w2103:i32)
                n1525 = local write "NRewards"(w2103) -> ()
                n1526 = local read "mL Per Ms"() -> (w2096:dbl)
                n1527 = To Double Precision Float(number=w2091) -> (double precision float=w2094:dbl)
                n1528 = local read "mL given"() -> (w2092:dbl)
                n1529 = Multiply(x=w2096, y=w2094) -> (x*y=w2093:dbl)
                n1530 = Add(x=w2092, y=w2093) -> (x+y=w2095:dbl)
                n1531 = local write "mL given"(w2095) -> ()
                n1532 = local write "AllowReward"(FALSE ("AllowReward")) -> ()
                n1533 = local write "Hit"(TRUE ("Hit")) -> ()
              }
            }
            n1534 = local read "response time"() -> (w2070:u32)
            n1535 = local read "cue time"() -> (w2074:u32)
            n1536 = local read "Response Times"() -> (w2073:dbl[])
            n1537 = local write "response window is open"(w2068) -> ()
            n1538 = Subtract(x=w2070, y=w2074) -> (x-y=w2069:u32)
            n1539 = Build Array (concatenate)(w2073, w2069) -> (w2072:dbl[])
            n1540 = To Double Precision Float(number=w2069) -> (double precision float=→"last response time (ms)":dbl)
            n1541 = Bundle By Name(cluster=w2065, "Water Valve"=w2063) -> (w2064:T26)
            n1542 = local write "Response Times"(w2072) -> ()
          }
          event "Abort Protocol": Mouse Down {
            n1543 = event-data() -> ()  [unwired: 1 in, 8 out]
            n1544 = local read "Abort Protocol"() -> (w2113:bool)
            n1545 = case shown="True" w2113 {
              frame False {
              }
              frame True {
                n1546 = property on="Abort Protocol" class="Bool (strict)"("DisabledEnum"=T22."Disabled" ("Disabled")) -> ()  [unwired: 2 in, 2 out]
              }
            }
          }
          event "Quit": Mouse Down {
            n1547 = event-data() -> ()  [unwired: 1 in, 8 out]
            n1548 = local read "Start Protocol"() -> (w2117:bool)
            n1549 = local write "Exit Program"(TRUE ("Exit Program")) -> ()
            n1550 = case shown="True" w2117 {
              frame False {
              }
              frame True {
                n1551 = local write "Abort Protocol"(TRUE ("Abort Protocol")) -> ()
              }
            }
            n1552 = local write "Leave Acquisition Run State"(DataAquisitionStates."Quit Data Acquisition") -> ()
          }
        }
      }
      frame "Quit Event Loop" {
        n1553 = Unbundle By Name(w2121) -> ("Water Valve"=w2124:refnum<k21>, "Airpuff"=w2123:refnum<k21>, "Light Switch"=w2122:refnum<k21>)
        n1554 = call <vilib>:"DAQmx Clear Task.vi"("task in"=w2124) -> ()  [unwired: 14 in, 1 out]
        n1555 = call <vilib>:"DAQmx Clear Task.vi"("task in"=w2123) -> ()  [unwired: 14 in, 1 out]
        n1556 = call <vilib>:"DAQmx Clear Task.vi"("task in"=w2122) -> ()  [unwired: 14 in, 1 out]
      }
    }
    n1557 = local read "Exit Program"() -> (w1434:bool)
  }
  n1558 = while {
    shift-right: [w2133] -> _
    shift-left: _ -> [w2134]
    shift-right: [w2135] -> _
    shift-left: _ -> [w2136]
    shift-right: [w2130] -> _
    shift-left: w14 -> [w2132]
    shift-right: [w2129] -> _
    shift-left: _ -> [w2128]
    shift-right: [w2127] -> _
    shift-left: _ -> [w2126]
    stop <- w2131 stop-if-true
    # "Data Acquisition, Lick Detection and Display Loop"
    n1559 = case shown="\"Start Data Logging\"" w2132 {
      tunnel: w2136 -> [_ w2244 w2316 w2332 w2346]
      tunnel: [w2175 w2243 w2315 w2329 w2346] -> w2135
      tunnel: w2134 -> [_ w2242 w2319 w2336 _]
      tunnel: [w2173 w2239 w2319 w2336 dbl[][] [] ("Graph Buffer")] -> w2133
      tunnel: [FALSE FALSE FALSE FALSE TRUE] -> w2131
      tunnel: [DataAquisitionStates."Run Data Acquisition" w2217 DataAquisitionStates."Run Data Acquisition" DataAquisitionStates."Run Data Acquisition" DataAquisitionStates."Quit Data Acquisition"] -> w2130
      tunnel: [refnum<k34> refnum ("tdms file out") w2224 w2301 refnum<k34> refnum ("tdms file out") w2342] -> w2129
      tunnel: w2128 -> [_ w2214 _ w2334 w2342]
      tunnel: [w2137 _ _ _ w2339] -> w2127
      tunnel: w2126 -> [_ _ _ _ w2340]
      frame "Init Data Acquisition" {
        w2173 = dbl[][] []  # Graph Buffer
        w2178 = 0 items=["one channel for each line", "one channel for all lines"] ("line grouping")
        w2176 = 10123 items=["Finite Samples"=10178, "Continuous Samples"=10123, "Hardware Timed Single Point"=12522] ("sample mode")
        # "Not sampled from DAQ"
        # "Some parameters depending on the sampling rate"
        # "Start Data Acquisition"
        # "Configure Sampling"
        # "Line 0.1 = Lick detect\nLine 0.4 = Beep\nLine 0.0 = Water"
        n1560 = local write "Licked"(FALSE ("Licked")) -> ()
        n1561 = Index Array(array="Sampling - Labels,  Lines In", index (col)=1 ("disabled index (col)")) -> (element=w2145:string[])  [unwired: 1 in]
        n1562 = Index Array(array="Sampling - Labels,  Lines In", index (col)=0 ("disabled index (col)")) -> (element=w2142:string[])  [unwired: 1 in]
        n1563 = property on="PrevLickState" class="DigNum (strict)"("Visible"=FALSE) -> ()  [unwired: 2 in, 2 out]
        n1564 = disable-structure shown="Disabled" {
          disable-tunnel: [w2179 _] -> w2137
          frame Disabled {
            n1565 = call-poly <vilib>:"DAQmx Create Virtual Channel.vi"("counter"=tag "Dev1/ctr3", "name to assign"="stage position", "pulses per revolution"=u32 36000) -> ("task out"=w2179:refnum<k21>)  [unwired: 11 in, 1 out]
          }
          frame Enabled {
          }
        }
        n1566 = call <vilib>:"DAQmx Flatten Channel String.vi"("names in"=w2145) -> ("names out"=w2177:string)  [unwired: 13 in, 1 out]
        n1567 = call <vilib>:"DAQmx Flatten Channel String.vi"("names in"=w2142) -> ("names out"=w2144:string)  [unwired: 13 in, 1 out]
        n1568 = Build Array (concatenate)(w2142, string[] ["Stage Position", "Stage Moving", "Wall Position", "Wall Moving", "Trial Counter", "Trial State", "Pupil Sample No"] ("channel name(s) in (Untitled)")) -> (→"channel names":string[])
        n1569 = property on="channel names" class="Arr (strict)"("Visible"=FALSE) -> ()  [unwired: 2 in, 2 out]
        n1570 = call-poly <vilib>:"DAQmx Create Virtual Channel.vi"("lines"=w2177, "name to assign"=w2144, "line grouping"=w2178) -> ("task out"=w2139:refnum<k21>)  [unwired: 11 in, 1 out]
        n1571 = property on="NLicks" class="Arr (strict)"("Visible"=FALSE) -> ()  [unwired: 2 in, 2 out]
        n1572 = property on="LickPerMin" class="Arr (strict)"("Visible"=FALSE) -> ()  [unwired: 2 in, 2 out]
        n1573 = property on="Leave Acquisition Run State" class="Enum (strict)"("Visible"=FALSE) -> ()  [unwired: 2 in, 2 out]
        n1574 = Divide(x="Sample Rate", y="Graph Update Rate (fps)") -> (x/y=w2172:dbl)
        n1575 = Multiply(x="Graph Length (s)", y="Graph Update Rate (fps)") -> (x*y=w2171:dbl)
        n1576 = To Long Integer(number=w2172) -> (32bit integer=→"Samples to Read":i32)
        n1577 = To Long Integer(number=w2171) -> (32bit integer=→"Buffer Length":i32)
        n1578 = call-poly <vilib>:"DAQmx Timing.vi"("task/channels in"=w2139, "sample mode"=w2176, "rate"="Sample Rate", "source"=tag "OnboardClock") -> ("task out"=w2159:refnum<k21>)  [unwired: 10 in, 1 out]
        n1579 = property on="Logging Data" class="Bool (strict)"("Visible"=FALSE) -> ()  [unwired: 2 in, 2 out]
        n1580 = local write "Start Data Logging"(FALSE ("Start Data Logging")) -> ()
        n1581 = property on="Start Data Logging" class="Bool (strict)"("Visible"=FALSE) -> ()  [unwired: 2 in, 2 out]
        n1582 = property on="Buffer Length" class="DigNum (strict)"("Visible"=FALSE) -> ()  [unwired: 2 in, 2 out]
        n1583 = property on="Samples to Read" class="DigNum (strict)"("Visible"=FALSE) -> ()  [unwired: 2 in, 2 out]
        n1584 = call <vilib>:"DAQmx Start Task.vi"("task/channels in"=w2159) -> ("task out"=w2175:refnum<k21>)  [unwired: 13 in, 1 out]
        n1585 = invoke on="LickPerMin" class="Arr (strict)" method="Reinit To Default"() -> ()  [unwired: 3 in, 3 out]
        n1586 = local write "Stop Data Logging"(FALSE ("Stop Data Logging")) -> ()
        n1587 = property on="Stop Data Logging" class="Bool (strict)"("Visible"=FALSE) -> ()  [unwired: 2 in, 2 out]
        n1588 = flat-sequence {
          frame #0 {
            # "Data Acquisition Start Time"
            n1589 = Tick Count (ms)() -> (millisecond timer value=w2183:u32)
            n1590 = local write "Recording Start Time"(w2183) -> ()
          }
        }
        n1591 = invoke on="Lick Rates" class="WFGraph (strict)" method="Reinit To Default"() -> ()  [unwired: 3 in, 3 out]
        "NLicks" <- i32[] [0, 0, 0] ("NLicks")
        "Logging Data" <- FALSE ("Logging Data")
      }
      frame "Run Data Acquisition", Default {
        # "Naive Filter"
        # "Normalize -->"
        # "Extract columns -->"
        n1592 = local read "Samples to Read"() -> (w2227:i32)
        n1593 = local read "Logging Data"() -> (w2213:bool)
        n1594 = local read "Stage Moving?"() -> (w2215:bool)
        n1595 = call-poly <vilib>:"DAQmx Read.vi"("task/channels in"=w2244, "number of samples per channel"=w2227) -> ("task out"=w2243:refnum<k21>, "data"=w2186:u8[][])  [unwired: 11 in, 1 out]
        n1596 = Index Array(array=w2186, index (row)=5 ("index")) -> (element=w2185:u8[])  [unwired: 1 in]
        n1597 = Array Max & Min(array=w2185) -> (min value=w2184:u8)  [unwired: 3 out]
        n1598 = Index Array(array=w2186, index (row)=4 ("index")) -> (element=w2198:u8[])  [unwired: 1 in]
        n1599 = Array Max & Min(array=w2198) -> (min value=w2197:u8)  [unwired: 3 out]
        n1600 = Index Array(array=w2186, index (row)=0) -> (element=w2233:u8[])  [unwired: 1 in]
        n1601 = Index Array(array=w2186, index (row)=1 ("index")) -> (element=w2232:u8[])  [unwired: 1 in]
        n1602 = Index Array(array=w2186, index (row)=2 ("index")) -> (element=w2205:u8[])  [unwired: 1 in]
        n1603 = Index Array(array=w2186, index (row)=3 ("index")) -> (element=w2211:u8[])  [unwired: 1 in]
        n1604 = To Double Precision Float(number=w2211) -> (double precision float=w2210:dbl[])
        n1605 = Divide(x=w2233, y=8.0) -> (x/y=w2231:dbl[])
        n1606 = Divide(x=w2232, y=16) -> (x/y=w2230:dbl[])
        n1607 = Divide(x=w2205, y=128) -> (x/y=w2204:dbl[])
        n1608 = Array Max & Min(array=w2231) -> (min value=w2223:dbl)  [unwired: 3 out]
        n1609 = Array Max & Min(array=w2230) -> (min value=w2228:dbl)  [unwired: 3 out]
        n1610 = Array Max & Min(array=w2204) -> (min value=w2229:dbl)  [unwired: 3 out]
        n1611 = call <vilib>:"Median.vi"("X"=w2210) -> ("median"=w2195:dbl)  [unwired: 1 out]
        n1612 = disable-structure shown="Disabled" {
          disable-tunnel: w2184 -> [w2246 _]
          frame Disabled {
            n1613 = Greater Than 0?(x=w2246) -> (x > 0?=w2245:bool)
            "wall ref" <- w2245
            n1614 = global write "GlobalVariables.vi" "Wall Position Reset Global"(w2245) -> ()
          }
          frame Enabled {
          }
        }
        n1615 = local read "FrameCount"() -> (w2190:dbl)
        n1616 = Build Array(w2223, w2228, w2229, w2195, w2197, w2184) -> (w2209:dbl[])
        n1617 = case shown="True" w2213 {
          tunnel: w2209 -> [_ w2280]
          tunnel: [w2258 w2279] -> w2224
          tunnel: w2214 -> [w2258 w2270]
          frame False {
          }
          frame True {
            # "See init case:"
            # "Stream acquired data (filtered and downsampled) and other trial variables to tdms file"
            n1618 = local read "Pupil Sample No"() -> (w2260:i32)
            n1619 = local read "channel names"() -> (w2259:string[])
            n1620 = local read "Trial Counter"() -> (w2278:i32)
            n1621 = local read "ArenaState"() -> (w2269:T6)
            n1622 = local read "Trial State"() -> (w2277:i32)
            n1623 = local read "SessionID"() -> (w2271:string)
            n1624 = Unbundle(w2269) -> ("Stage Position"=w2268:dbl, "Stage Moving?"=w2267:bool, "Wall Position"=w2264:dbl, "Wall Moving"=w2263:bool)
            n1625 = Boolean To (0,1)(Boolean=w2267) -> (0, 1=w2282:i16)
            n1626 = Boolean To (0,1)(Boolean=w2263) -> (0, 1=w2262:i16)
            n1627 = To Double Precision Float(number=w2262) -> (double precision float=w2261:dbl)
            n1628 = To Double Precision Float(number=w2282) -> (double precision float=w2281:dbl)
            n1629 = To Double Precision Float(number=w2278) -> (double precision float=w2265:dbl)
            n1630 = To Double Precision Float(number=w2277) -> (double precision float=w2266:dbl)
            n1631 = Build Array (concatenate)(w2280, w2268, w2281, w2264, w2261, w2265, w2266, w2260) -> (w2276:dbl[])
            n1632 = Reshape Array(w2276, 1 ("dimension size"), 12 ("dimension size")) -> (w2273:dbl[][])
            n1633 = TDMS Write(0:w2270, 1:enum16{"decimated", "interleaved"}."interleaved" ("data layout (0:decimated)"), 5:w2271, 7:w2259, 9:w2273) -> (4:w2279:refnum<k34>)  [unwired: 1 in, 3 out]
          }
        }
        n1634 = feedback-in #3(w2195) -> ()
        n1635 = feedback #3(0.0 ("median")) -> (w2194:dbl)
        n1636 = Greater?(x=w2195, y=w2194) -> (0:w2193:bool)
        n1637 = Greater Than 0?(x=w2223) -> (x > 0?=w2226:bool)
        n1638 = Select(t=1.0, s=w2193, f=0.0) -> (s? t:f=w2188:dbl)
        n1639 = Add(x=w2190, y=w2188) -> (x+y=w2189:dbl)
        n1640 = local write "FrameCount"(w2189) -> ()
        n1641 = local read "Session Running"() -> (w2200:bool)
        n1642 = case shown="True" w2226 {
          frame False {
          }
          frame True {
            # "Generate a lick event if mouse licked within response window"
            n1643 = local read "Waiting for lick"() -> (w2285:bool)
            n1644 = case shown="True" w2285 {
              frame False {
              }
              frame True {
                n1645 = Tick Count (ms)() -> (millisecond timer value=w2288:u32)
                n1646 = local write "response time"(w2288) -> ()
                n1647 = local write "Waiting for lick"(FALSE ("Waiting for response")) -> ()
                n1648 = property on="Licked" class="Bool (strict)"("Val(Sgnl)"=TRUE) -> ()  [unwired: 2 in, 2 out]
              }
            }
          }
        }
        n1649 = Array Subset(array=w2209, index=0, length=3) -> (w2203:dbl[])
        n1650 = local read "Response Window"() -> (w2201:dbl)
        n1651 = case shown="True" w2200 {
          tunnel: w2223 -> [_ w2256]
          tunnel: w2215 -> [_ w2247]
          frame False {
          }
          frame True {
            n1652 = local read "Recording Start Time"() -> (w2248:u32)
            n1653 = local read "PrevLickState"() -> (w2255:dbl)
            n1654 = local read "NLicks"() -> (w2254:i32[])
            n1655 = local read "LickPerMin"() -> (w2249:i32[][])
            n1656 = call "CountLicks.vi"("StageMoving?"=w2247, "Start time"=w2248, "LickPerMinIn"=w2249, "NLicks In"=w2254, "Previous Lick State"=w2255, "Current Lick State"=w2256) -> ("LickPerMinOut"=w2250:i32[][], "NLicksOut"=w2253:i32[], "NewVal?"=w2251:bool, "Current Lick State Out"=w2252:dbl)  [unwired: 1 in]
            n1657 = local write "PrevLickState"(w2252) -> ()
            n1658 = local write "LickPerMin"(w2250) -> ()
            n1659 = local write "NLicks"(w2253) -> ()
            n1660 = case shown="True" w2251 {
              tunnel: w2250 -> [_ w2257]
              frame False {
              }
              frame True {
                "Lick Rates" <- w2257
              }
            }
          }
        }
        n1661 = local read "Exit Program"() -> (w2219:bool)
        n1662 = local read "Stop Data Logging"() -> (w2220:bool)
        n1663 = local read "Start Data Logging"() -> (w2221:bool)
        n1664 = Build Array (concatenate)(w2203, w2201) -> (w2202:dbl[])
        n1665 = local read "Recording Start Time"() -> (w2222:u32)
        n1666 = local read "Graph Update Rate (fps)"() -> (w2216:dbl)
        n1667 = local read "Buffer Length"() -> (w2238:i32)
        n1668 = Compound Arithmetic op=OR(w2219, w2220, w2221) -> (w2218:bool)
        n1669 = case shown="True" w2218 {
          tunnel: [DataAquisitionStates."Run Data Acquisition" w2284] -> w2217
          frame False {
          }
          frame True {
            n1670 = local read "Leave Acquisition Run State"() -> (w2284:T12)
          }
        }
        n1671 = call "PrepareDataForPlot.vi"("Sample Rate"=w2216, "Start Time (ms)"=w2222, "Buffer Length"=w2238, "Graph Buffer In"=w2242, "New Samples"=w2202) -> ("Graph Buffer Out"=w2239:dbl[][], "WaveForm Data"=→"Lick detection":cluster{dbl, dbl, dbl[][]})  [unwired: 5 in]
      }
      frame "Start Data Logging" {
        w2311 = 15842 items=["Off"=10231, "Log"=15844, "Log and Read"=15842] ("logging mode")
        w2314 = 15846 items=["Open"=10437, "Open or Create"=15846, "Create or Replace"=15847, "Create"=15848] ("operation")
        # "Configure Data Logging"
        n1672 = local read "RecordingFolder"() -> (w2290:path)
        n1673 = local read "SessionID"() -> (w2297:string)
        n1674 = call <vilib>:"DAQmx Stop Task.vi"("task/channels in"=w2316) -> ("task out"=w2312:refnum<k21>)  [unwired: 13 in, 1 out]
        n1675 = local read "SessionID"() -> (w2291:string)
        n1676 = Concatenate Strings(w2297, "-raw_lickport_data.tdms" ("Data Type")) -> (w2295:string)
        n1677 = Concatenate Strings(w2291, "-processed_setup_data.tdms" ("Data Type")) -> (w2293:string)
        n1678 = Build Path(base path=w2290, name or relative path=w2295) -> (appended path=w2294:path)
        n1679 = Build Path(base path=w2290, name or relative path=w2293) -> (appended path=w2289:path)
        n1680 = local read "SessionID"() -> (w2299:string)
        n1681 = call-poly <vilib>:"DAQmx Configure Logging.vi"("task/channels in"=w2312, "operation"=w2314, "file path"=w2294, "group name"=w2299, "logging mode"=w2311) -> ("task out"=w2313:refnum<k21>, "error out"=w2305:errorcluster)  [unwired: 9 in]
        n1682 = TDMS Open(10:T24."open or create" ("operation (0:open)"), 11:w2289) -> (0:w2304:errorcluster, 3:w2309:refnum<k34>)  [unwired: 5 in]
        n1683 = local read "Graph Update Rate (fps)"() -> (w2307:dbl)
        n1684 = Build Array(w2307) -> (w2306:dbl[])
        n1685 = call <vilib>:"DAQmx Start Task.vi"("task/channels in"=w2313, "error in"=w2305) -> ("task out"=w2315:refnum<k21>, "error out"=w2298:errorcluster)  [unwired: 12 in]
        n1686 = TDMS Set Properties(5:w2306, 7:string[] ["Sampling Rate"] ("property names"), 8:w2304, 10:w2299, 11:w2309) -> (0:w2303:errorcluster, 3:w2301:refnum<k34>)  [unwired: 1 in, 2 out]
        n1687 = Merge Errors(w2298, w2303) -> (w2302:errorcluster)
        n1688 = case shown="No Error" w2302 {
          frame No Error {
            n1689 = local write "Start Data Logging"(FALSE ("Start Data Logging")) -> ()
          }
          frame Error {
          }
        }
        n1690 = disable-structure shown="Disabled" {
          frame Disabled {
            n1691 = local write "Trigger microscope"(TRUE) -> ()
          }
          frame Enabled {
          }
        }
        n1692 = local write "Logging Data"(TRUE ("Logging Data")) -> ()
      }
      frame "End Data Logging" {
        w2333 = 10231 items=["Off"=10231, "Log"=15844, "Log and Read"=15842] ("logging mode")
        n1693 = call <vilib>:"DAQmx Stop Task.vi"("task/channels in"=w2332) -> ("task out"=w2331:refnum<k21>)  [unwired: 13 in, 1 out]
        n1694 = call-poly <vilib>:"DAQmx Configure Logging.vi"("task/channels in"=w2331, "file path"=path "", "logging mode"=w2333) -> ("task out"=w2330:refnum<k21>, "error out"=w2328:errorcluster)  [unwired: 11 in]
        n1695 = TDMS Close(11:w2334) -> (0:w2327:errorcluster)  [unwired: 1 in, 1 out]
        n1696 = call <vilib>:"DAQmx Start Task.vi"("task/channels in"=w2330, "error in"=w2328) -> ("task out"=w2329:refnum<k21>, "error out"=w2326:errorcluster)  [unwired: 12 in]
        n1697 = Merge Errors(w2326, w2327) -> (w2325:errorcluster)
        n1698 = case shown="No Error" w2325 {
          frame No Error {
            n1699 = local write "Stop Data Logging"(FALSE ("Stop Data Logging")) -> ()
          }
          frame Error {
          }
        }
        n1700 = local write "Logging Data"(FALSE ("Logging Data")) -> ()
      }
      frame "Quit Data Acquisition" {
        n1701 = disable-structure shown="Disabled" {
          disable-tunnel: w2340 -> [w2349 _]
          disable-tunnel: [w2348 _] -> w2339
          frame Disabled {
            n1702 = call <vilib>:"DAQmx Stop Task.vi"("task/channels in"=w2349) -> ("task out"=w2348:refnum<k21>)  [unwired: 13 in, 1 out]
            n1703 = call <vilib>:"DAQmx Clear Task.vi"("task in"=w2348) -> ()  [unwired: 14 in, 1 out]
          }
          frame Enabled {
          }
        }
        n1704 = call <vilib>:"DAQmx Stop Task.vi"("task/channels in"=w2346) -> ("task out"=w2347:refnum<k21>)  [unwired: 13 in, 1 out]
        n1705 = TDMS Close(11:w2342) -> (0:w2341:errorcluster)  [unwired: 1 in, 1 out]
        n1706 = call <vilib>:"DAQmx Clear Task.vi"("task in"=w2347) -> ()  [unwired: 14 in, 1 out]
        n1707 = call <vilib>:"Clear Errors.vi"("error in (no error)"=w2341) -> ()  [unwired: 6 in, 1 out]
      }
    }
  }
  n1708 = while {
    shift-right: [w2350] -> _
    shift-left: w2 -> [w2351]
    stop <- w2352 stop-if-true
    # "Rotation Stage Status Loop"
    n1709 = case shown="\"Get Stage Info\"" w2351 {
      tunnel: [FALSE FALSE TRUE] -> w2352
      tunnel: [w2385 w2433 RotationStageStates."Disconnect Stage"] -> w2350
      frame "Connect Stage" {
        w2366 = T20 0 items=["Grayscale (U8)", "Grayscale (I16)", "Grayscale (SGL)", "Complex (CSG)", "RGB (U32)", "HSL (U32)", "RGB (U64)", "Grayscale (U16)"] ("Image Type")
        w2367 = T20 0 items=["Grayscale (U8)", "Grayscale (I16)", "Grayscale (SGL)", "Complex (CSG)", "RGB (U32)", "HSL (U32)", "RGB (U64)", "Grayscale (U16)"] ("Image Type")
        w2368 = T20 0 items=["Grayscale (U8)", "Grayscale (I16)", "Grayscale (SGL)", "Complex (CSG)", "RGB (U32)", "HSL (U32)", "RGB (U64)", "Grayscale (U16)"] ("Image Type")
        w2369 = T20 0 items=["Grayscale (U8)", "Grayscale (I16)", "Grayscale (SGL)", "Complex (CSG)", "RGB (U32)", "HSL (U32)", "RGB (U64)", "Grayscale (U16)"] ("Image Type")
        w2370 = T20 0 items=["Grayscale (U8)", "Grayscale (I16)", "Grayscale (SGL)", "Complex (CSG)", "RGB (U32)", "HSL (U32)", "RGB (U64)", "Grayscale (U16)"] ("Image Type")
        n1710 = case shown="True" "Stage connected" {
          tunnel: [RotationStageStates."Disconnect Stage" RotationStageStates."Get Stage Info"] -> w2385
          frame False {
          }
          frame True {
            # "Start communication driver for steinmeyer motor"
            # "Initialize communication with the connected motor"
            n1711 = call "InitCommunication.vi"() -> ()  [unwired: 3 in]
          }
        }
        n1712 = case shown="True" "Wall connected" {
          tunnel: refnum<class "StepperController.lvclass"> refnum ("StepperController.lvclass") -> [_ w2397]
          tunnel: [FALSE TRUE] -> w2358
          frame False {
          }
          frame True {
            n1713 = call-dynamic "InitDAQmx.vi"("TerminalDirection"="DAQmx step-dir line", "CounterStep"="DAQmx step counter", "TerminalStep"="DAQmx step terminal", "StepperController in"=w2397) -> ("StepperController out"=w2393:refnum<class "StepperController.lvclass">)  [unwired: 6 in, 1 out]
            n1714 = local read "Wall physical step size (deg/step)"() -> (w2392:dbl)
            n1715 = local read "Wall max rotation"() -> (w2391:dbl)
            n1716 = call-dynamic "Init.vi"("MaxRotation"=w2391, "PhysicalStepSize"=w2392, "StepperController in"=w2393) -> ("StepperController out"=w2390:refnum<class "StepperController.lvclass">)  [unwired: 7 in, 1 out]
            n1717 = local write "StepperController.lvclass"(w2390) -> ()
          }
        }
        n1718 = call "IMAQ Create"("Border Size"=0, "Image Name"="mouse", "Image Type"=w2370) -> ("New Image"=w2378:T1)  [unwired: 2 in, 1 out]
        n1719 = call "IMAQ Create"("Border Size"=0, "Image Name"="arena", "Image Type"=w2369) -> ("New Image"=w2376:T1)  [unwired: 2 in, 1 out]
        n1720 = call "IMAQ ReadFile"("File Path"=path "F:/Development/labview software/ActiveRotationExperiments/image_mouse.tif", "Image"=w2378) -> ("Image Out"=→"mouse":T1)  [unwired: 5 in, 4 out]
        n1721 = call "IMAQ ReadFile"("File Path"=path "F:/Development/labview software/ActiveRotationExperiments/image_arena.tif", "Image"=w2376) -> ("Image Out"=→"arena":T1)  [unwired: 5 in, 4 out]
        n1722 = local write "Init Stepper Move"(w2358) -> ()
        n1723 = property on="tmp_mouse" class="IMAQImage (strict)"("Visible"=FALSE) -> ()  [unwired: 2 in, 2 out]
        n1724 = property on="mouse" class="IMAQImage (strict)"("Visible"=FALSE) -> ()  [unwired: 2 in, 2 out]
        n1725 = call "IMAQ Create"("Border Size"=0, "Image Name"="arena_display", "Image Type"=w2366) -> ("New Image"=→"arena_display":T1)  [unwired: 2 in, 1 out]
        n1726 = call "IMAQ Create"("Border Size"=0, "Image Name"="tmp_arena", "Image Type"=w2367) -> ("New Image"=→"tmp_arena":T1)  [unwired: 2 in, 1 out]
        n1727 = call "IMAQ Create"("Border Size"=0, "Image Name"="tmp_mouse", "Image Type"=w2368) -> ("New Image"=→"tmp_mouse":T1)  [unwired: 2 in, 1 out]
        n1728 = property on="arena_display" class="IMAQImage (strict)"("Visible"=FALSE) -> ()  [unwired: 2 in, 2 out]
        n1729 = property on="arena" class="IMAQImage (strict)"("Visible"=FALSE) -> ()  [unwired: 2 in, 2 out]
        n1730 = property on="tmp_arena" class="IMAQImage (strict)"("Visible"=FALSE) -> ()  [unwired: 2 in, 2 out]
      }
      frame "Get Stage Info" {
        w2409 = sgl 255.0 ("Replace Value")
        # "Create rotating mouse animation to indicate stage position"
        n1731 = local read "Wall Moving?"() -> (w2404:bool)
        n1732 = local read "Session Running"() -> (w2401:bool)
        n1733 = local read "StepperController.lvclass"() -> (w2411:refnum<class "StepperController.lvclass">)
        n1734 = case shown="True" w2404 {
          tunnel: [w2436 w2443] -> w2410
          tunnel: w2411 -> [w2437 w2442]
          tunnel: w2401 -> [w2435 _]
          frame False {
            n1735 = case shown="True" w2435 {
              tunnel: w2437 -> [w2438 w2440]
              tunnel: [w2438 w2439] -> w2436
              frame False {
              }
              frame True {
                n1736 = call "SetPos.vi"("StepperController in"=w2440) -> ("StepperController out"=w2439:refnum<class "StepperController.lvclass">)  [unwired: 2 in, 1 out]
              }
            }
          }
          frame True {
            # "Update movement status of stepper"
            n1737 = call "IsMoving.vi"("StepperController in"=w2442) -> ("error out"=w2441:errorcluster, "IsMoving"=w2445:bool, "StepperController out"=w2444:refnum<class "StepperController.lvclass">)  [unwired: 2 in]
            n1738 = case shown="Error" w2441 {
              tunnel: w2445 -> [w2448 _]
              tunnel: w2444 -> [w2447 w2453]
              tunnel: [w2446 w2453] -> w2443
              frame No Error {
                n1739 = case shown="False" w2448 {
                  tunnel: w2447 -> [w2450 w2452]
                  tunnel: [w2449 w2452] -> w2446
                  frame False {
                    n1740 = local write "Wall Moving?"(FALSE ("Moving")) -> ()
                    n1741 = call "StopTask.vi"("StepperController in"=w2450) -> ("StepperController out"=w2449:refnum<class "StepperController.lvclass">)  [unwired: 1 in, 1 out]
                  }
                  frame True {
                  }
                }
              }
              frame Error {
                n1742 = local write "Wall Moving?"(FALSE ("Moving")) -> ()
              }
            }
          }
        }
        n1743 = local read "mouse"() -> (w2424:T1)
        n1744 = local read "tmp_mouse"() -> (w2421:T1)
        n1745 = local read "arena"() -> (w2423:T1)
        n1746 = local read "tmp_arena"() -> (w2420:T1)
        n1747 = call "IMAQ Copy"("Image Dst"=w2421, "Image Src"=w2424) -> ("Image Dst Out"=w2413:T1)  [unwired: 4 in, 1 out]
        n1748 = call "IMAQ Copy"("Image Dst"=w2420, "Image Src"=w2423) -> ("Image Dst Out"=w2414:T1)  [unwired: 4 in, 1 out]
        n1749 = global read "GlobalVariables.vi" "Wall Position Global"() -> (w2400:dbl)
        n1750 = call "SMGetPosition.vi"() -> ("Motor Position"=w2422:dbl)  [unwired: 11 in]
        n1751 = call "IMAQ Rotate"("Maintain Size"=TRUE, "Replace Value"=w2409, "Angle (degrees)"=w2422, "Image Src"=w2413) -> ("Image Dst Out"=w2419:T1)  [unwired: 6 in, 1 out]
        n1752 = call "IMAQ Rotate"("Maintain Size"=TRUE, "Replace Value"=w2409, "Angle (degrees)"=w2400, "Image Src"=w2414) -> ("Image Dst Out"=w2412:T1)  [unwired: 6 in, 1 out]
        n1753 = call <instrlib>:"TS_CheckEvent.vi"() -> ("Event"=w2429:bool)  [unwired: 1 out]
        n1754 = Not(x=w2429) -> (.not. x?=w2425:bool)
        n1755 = local write "StepperController.lvclass"(w2410) -> ()
        n1756 = local read "Wall Position"() -> (w2403:dbl)
        n1757 = local read "Wall Moving?"() -> (w2402:bool)
        n1758 = local write "Stage Position"(w2422) -> ()
        n1759 = local write "Stage Moving?"(w2425) -> ()
        n1760 = local read "ArenaState"() -> (w2427:T6)
        n1761 = call "IMAQ ImageToArray"("Image"=w2419) -> ("Image Pixels (U8)"=w2408:u8[][])  [unwired: 3 in, 4 out]
        n1762 = call "IMAQ ImageToArray"("Image"=w2412) -> ("Image Pixels (U8)"=w2407:u8[][])  [unwired: 3 in, 4 out]
        n1763 = Bundle By Name(cluster=w2427, "Stage Position"=w2422, "Stage Moving?"=w2425, "Wall Position"=w2403, "Wall Moving"=w2402) -> (w2426:T6)
        n1764 = Add(x=w2408, y=w2407) -> (x+y=w2406:fxp<+,8,8>[][])
        n1765 = local read "arena_display"() -> (w2415:T1)
        n1766 = To Unsigned Byte Integer(number=w2406) -> (unsigned 8bit integer=w2405:u8[][])
        n1767 = local write "ArenaState"(w2426) -> ()
        n1768 = local read "Exit Program"() -> (w2430:bool)
        n1769 = call "IMAQ ArrayToImage"("Image Pixels (U8)"=w2405, "Image"=w2415) -> ("Image Out"=→"Stage Position 2":T1)  [unwired: 8 in, 1 out]
        n1770 = Wait (ms)(milliseconds to wait=u32 30) -> ()  [unwired: 1 out]
        n1771 = Select(t=RotationStageStates."Disconnect Stage", s=w2430, f=RotationStageStates."Get Stage Info") -> (s? t:f=w2433:T14)
      }
      frame "Disconnect Stage" {
        n1772 = local read "Wall connected"() -> (w2455:bool)
        n1773 = local read "Stage connected"() -> (w2456:bool)
        n1774 = case shown="True" w2456 {
          frame False {
          }
          frame True {
            n1775 = flat-sequence {
              frame #0 {
                n1776 = call "SMMoveAbsolute.vi"() -> ()  [unwired: 12 in]
              }
              frame #1 {
                n1777 = while {
                  stop <- w2463 stop-if-true
                  n1778 = call <instrlib>:"TS_CheckEvent.vi"() -> ("Event"=w2463:bool)  [unwired: 1 out]
                  n1779 = Not(x=w2463) -> (.not. x?=w2462:bool)
                  n1780 = call "SMGetPosition.vi"() -> ("Motor Position"=w2461:dbl)  [unwired: 11 in]
                  n1781 = local write "Stage Moving?"(w2462) -> ()
                  n1782 = local write "Stage Position"(w2461) -> ()
                  n1783 = Wait (ms)(milliseconds to wait=u32 30) -> ()  [unwired: 1 out]
                }
              }
              frame #2 {
                n1784 = call "CloseCommunication.vi"() -> ()  [unwired: 12 in]
              }
            }
          }
        }
        n1785 = case shown="True" w2455 {
          frame False {
          }
          frame True {
            n1786 = local read "StepperController.lvclass"() -> (w2460:refnum<class "StepperController.lvclass">)
            n1787 = call "Close.vi"("StepperController in"=w2460) -> ("StepperController out"=w2459:refnum<class "StepperController.lvclass">)  [unwired: 9 in, 1 out]
            n1788 = local write "StepperController.lvclass"(w2459) -> ()
          }
        }
      }
    }
  }
  n1789 = while {
    shift-right: [w2468] -> _
    shift-left: _ -> [w2469]
    shift-right: [w2472] -> _
    shift-left: _ -> [w2470]
    shift-right: [w2465] -> _
    shift-left: w6 -> [w2466]
    i -> [w2471]
    stop <- w2467 stop-if-true
    # "Acquire images from Eye camera and track pupil diameter and position"
    n1790 = case shown="\"Run Acquisition\"" w2466 {
      selector: w2466 -> [_ w2536 w2569 w2710 _]
      tunnel: [w2484 w2539 w2591 w2708 w2717] -> w2472
      tunnel: w2471 -> [_ _ w2590 _ _]
      tunnel: w2470 -> [w2485 w2539 w2585 w2708 w2717]
      tunnel: w2469 -> [_ w2540 w2575 w2713 w2718]
      tunnel: [dbl[][] [] w2540 w2574 w2713 w2718] -> w2468
      tunnel: [w2530 w2533 w2568 w2710 PupilTrackerStates."Idle"] -> w2465
      tunnel: [FALSE ("Stopped") FALSE ("Stopped") FALSE ("Stopped") TRUE ("Stopped") FALSE ("Stopped")] -> w2467
      frame "Initialize Eyetracker", Default {
        w2476 = T20 0 items=["Grayscale (U8)", "Grayscale (I16)", "Grayscale (SGL)", "Complex (CSG)", "RGB (U32)", "HSL (U32)", "RGB (U64)", "Grayscale (U16)"] ("Image Type")
        w2478 = T20 0 items=["Grayscale (U8)", "Grayscale (I16)", "Grayscale (SGL)", "Complex (CSG)", "RGB (U32)", "HSL (U32)", "RGB (U64)", "Grayscale (U16)"] ("Image Type")
        w2505 = T20 0 items=["Grayscale (U8)", "Grayscale (I16)", "Grayscale (SGL)", "Complex (CSG)", "RGB (U32)", "HSL (U32)", "RGB (U64)", "Grayscale (U16)"] ("Image Type")
        w2523 = T20 0 items=["Grayscale (U8)", "Grayscale (I16)", "Grayscale (SGL)", "Complex (CSG)", "RGB (U32)", "HSL (U32)", "RGB (U64)", "Grayscale (U16)"] ("Image Type")
        w2526 = T20 0 items=["Grayscale (U8)", "Grayscale (I16)", "Grayscale (SGL)", "Complex (CSG)", "RGB (U32)", "HSL (U32)", "RGB (U64)", "Grayscale (U16)"] ("Image Type")
        w2528 = T20 0 items=["Grayscale (U8)", "Grayscale (I16)", "Grayscale (SGL)", "Complex (CSG)", "RGB (U32)", "HSL (U32)", "RGB (U64)", "Grayscale (U16)"] ("Image Type")
        # "Error Variable"
        # "Internal boolen variables"
        # "Plot settings"
        # "Go to idle if camera is not connected"
        # "Variables for keeping track of lost frames"
        # "Create memory location for images"
        # "Array for storing loop durations"
        n1791 = property on="Cropped Image" class="IMAQImage (strict)"("Visible"=FALSE) -> ()  [unwired: 2 in, 2 out]
        n1792 = local write "Save Pupil Video"(FALSE ("Save Block Video")) -> ()
        n1793 = property on="Processed Image" class="IMAQImage (strict)"("Visible"=FALSE) -> ()  [unwired: 2 in, 2 out]
        n1794 = call "IMAQ Create"("Image Name"="cropped image", "Image Type"=w2528) -> ("New Image"=→"Cropped Image":T1)  [unwired: 3 in, 1 out]
        n1795 = call "IMAQ Create"("Image Name"="processed image", "Image Type"=w2526) -> ("New Image"=→"Processed Image":T1)  [unwired: 3 in, 1 out]
        n1796 = call "IMAQ Create"("Image Name"="fitted pupil image", "Image Type"=w2523) -> ("New Image"=→"Fitted Pupil Image":T1)  [unwired: 3 in, 1 out]
        n1797 = call "IMAQ Create"("Image Name"="processed image display", "Image Type"=w2505) -> ("New Image"=→"Processed Image Display":T1)  [unwired: 3 in, 1 out]
        n1798 = property on="Paused Acquisition" class="Bool (strict)"("Visible"=FALSE) -> ()  [unwired: 2 in, 2 out]
        n1799 = property on="Last Image number" class="DigNum (strict)"("Visible"=TRUE) -> ()  [unwired: 2 in, 2 out]
        n1800 = property on="Fitted Pupil Image" class="IMAQImage (strict)"("Visible"=FALSE) -> ()  [unwired: 2 in, 2 out]
        n1801 = property on="Processed Image Display" class="IMAQImage (strict)"("Visible"=FALSE) -> ()  [unwired: 2 in, 2 out]
        n1802 = control-ref of="Pupil Info"() -> (w2506:refnum<vi>)
        n1803 = local read "Track Every Nth Frame"() -> (w2516:i32)
        n1804 = local read "Acquisition Frame Rate"() -> (w2517:dbl)
        n1805 = property on="Pupil Info" class="WFChart (strict)"("YScale.Maximum"=100.0 ("Y Scale.Range:Increment"), "YScale.Minimum"=0.0 ("Y Scale.Range:Maximum"), "YScale.Increment"=20.0 ("Y Scale.Range:Minimum"), "YScale.MinorInc"=5.0 ("Y Scale.Range:Minor Increment")) -> ()  [unwired: 2 in, 2 out]
        n1806 = local read "Graph Length (s)"() -> (w2481:dbl)
        n1807 = property on="Pupil Sample No" class="DigNum (strict)"("Visible"=FALSE) -> ()  [unwired: 2 in, 2 out]
        n1808 = call "IMAQ Create"("Image Name"="fitted pupil image 2", "Image Type"=w2478) -> ("New Image"=→"Fitted Pupil Image 2":T1)  [unwired: 3 in, 1 out]
        n1809 = call "IMAQ Create"("Image Name"="pupil mask", "Image Type"=w2476) -> ("New Image"=→"Mask":T1)  [unwired: 3 in, 1 out]
        n1810 = To Double Precision Float(number=w2516) -> (double precision float=w2515:dbl)
        n1811 = Divide(x=w2515, y=w2517) -> (x/y=w2509:dbl)
        n1812 = call "InitializeTrackingParameters.vi"("Rectangular selection"=T29 {"Left"=1, "Top"=1, "Right"=600, "Bottom"=800, "Rotation"=0.0} ("Rectangle"), "Circle fit parameters in"=w2485) -> ("Circle fit parameters out"=w2484:T31)  [unwired: 3 in, 1 out]
        n1813 = call "SetWaveformXscale.vi"("Plot Duration"=w2481, "deltaT"=w2509, "WaveformChart in"=w2506) -> ()  [unwired: 9 in]
        n1814 = property on="Fitted Pupil Image 2" class="IMAQImage (strict)"("Visible"=FALSE) -> ()  [unwired: 2 in, 2 out]
        n1815 = local write "Recording Pupil Video"(FALSE ("Saving Pupil Video")) -> ()
        n1816 = local write "Track Pupil"(FALSE ("Track Pupil")) -> ()
        n1817 = local write "Save Tracking Results"(FALSE ("Save Tracking Results")) -> ()
        n1818 = property on="Mask" class="IMAQImage (strict)"("Visible"=FALSE) -> ()  [unwired: 2 in, 2 out]
        n1819 = property on="Stop Acquisition" class="Bool (strict)"("Visible"=FALSE) -> ()  [unwired: 2 in, 2 out]
        n1820 = property on="Save Tracking Results" class="Bool (strict)"("Visible"=FALSE) -> ()  [unwired: 2 in, 2 out]
        n1821 = property on="Save Pupil Video" class="Bool (strict)"("Visible"=FALSE) -> ()  [unwired: 2 in, 2 out]
        n1822 = property on="Vision Acquisition Error" class="Clust (strict)"("Visible"=FALSE) -> ()  [unwired: 2 in, 2 out]
        n1823 = Select(t=PupilTrackerStates."Run Acquisition", s="Pupil Camera Connected", f=PupilTrackerStates."Idle") -> (s? t:f=w2530:T16)
        "Last Image number" <- u32 0 ("Last Image number")
        "LostFrames" <- u32 0 ("LostFrames")
        "Stop Acquisition" <- FALSE ("Stop Acquisition")
        "Pupil marked" <- FALSE ("Pupil marked")
        "Paused Acquisition" <- FALSE ("Paused Acquisition")
      }
      frame "Idle" {
        n1824 = event shown="[0] Timeout" {
          selector: _ -> [_ _]
          dyn-events: _ -> [_ _]
          timeout: 30 -> [_ _]
          tunnel: [w2541 w2546] -> w2534
          tunnel: w2536 -> [w2541 w2545]
          event Timeout {
            n1825 = event-data() -> ()  [unwired: 1 in, 3 out]
          }
          event "Pupil Camera Connected": Value Change {
            n1826 = event-data() -> ()  [unwired: 1 in, 1 out]
            n1827 = local read "Pupil Camera Connected"() -> (w2542:bool)
            n1828 = Not(x=w2542) -> (.not. x?=w2543:bool)
            n1829 = Select(t=PupilTrackerStates."Run Acquisition", s=w2542, f=w2545) -> (s? t:f=w2546:T16)
            n1830 = local write "Stop Acquisition"(w2543) -> ()
          }
        }
        n1831 = local read "Exit Program"() -> (w2535:bool)
        n1832 = Select(t=PupilTrackerStates."Quit Eyetracker", s=w2535, f=w2534) -> (s? t:f=w2533:T16)
      }
      frame "Run Acquisition" {
        # "Save cropped image"
        # "Crop image based on selection of eye location"
        # "Adjustables"
        n1833 = local read "Exit Program"() -> (w2564:bool)
        n1834 = call "TimeLoop.vi"("Loop durations in"=w2575) -> ("Average fps"=→"Avg freq":dbl, "Loop durations out"=w2574:dbl[][])  [unwired: 5 in]
        n1835 = call "Vision Acquisition2"("Analog Control::Gain"="Gain", "Analog Control::Black Level"="Black Level", "Acquisition Control::Exposure Time"="Exposure Time", "Acquisition Control::Acquisition Frame Rate"="Acquisition Frame Rate", "Stop (F)"=w2564) -> ("Image Out"=w2582:T1, "Image Number"=w2578:u32, "Frame Rate"=→"Frame Rate Eyetracker":dbl, "Stopped"=w2567:bool, "error out"=w2563:errorcluster)  [unwired: 17 in, 1 out]
        n1836 = event shown="[1] \"Select Pupil Area\": Mouse Down" {
          selector: _ -> [_ _ _ _ _ _ _ _ _ _]
          dyn-events: _ -> [_ _ _ _ _ _ _ _ _ _]
          timeout: 1 -> [_ _ _ _ _ _ _ _ _ _]
          tunnel: w2582 -> [_ w2640 w2653 _ _ _ _ _ _ _]
          tunnel: w2585 -> [w2634 w2645 w2652 w2665 w2675 w2684 w2688 w2695 w2702 w2707]
          tunnel: [w2634 w2637 w2651 w2664 w2674 w2682 w2686 w2693 w2702 w2707] -> w2573
          tunnel: w2569 -> [w2628 w2643 w2647 w2662 w2673 _ w2685 w2694 w2703 w2706]
          tunnel: [w2629 w2643 w2647 w2662 w2673 _ w2685 w2694 w2703 w2706] -> w2568
          tunnel: w2567 -> [w2626 _ _ _ _ _ _ _ _ _]
          tunnel: w2563 -> [w2631 _ _ _ _ _ _ _ _ _]
          event Timeout {
            # "Go to error case if vision acquisition returns error"
            n1837 = event-data() -> ()  [unwired: 1 in, 1 out]
            n1838 = Select(t=PupilTrackerStates."Idle", s=w2626, f=w2628) -> (s? t:f=w2627:T16)
            n1839 = Unbundle By Name(w2631) -> ("status"=w2633:bool)
            n1840 = Select(t=PupilTrackerStates."Camera Error", s=w2633, f=w2627) -> (s? t:f=w2629:T16)
            n1841 = local write "Vision Acquisition Error"(w2631) -> ()
            n1842 = local write "Paused Acquisition"(w2626) -> ()
          }
          event "Select Pupil Area": Mouse Down {
            n1843 = event-data() -> ()  [unwired: 1 in, 1 out]
            n1844 = call "IMAQ Select Rectangle"("Prompt"="Crop Eye", "Image In"=w2640) -> ("Cancelled"=w2638:bool, "Rectangle"=w2639:T29)  [unwired: 6 in, 2 out]
            n1845 = local write "Paused Acquisition"(TRUE ("Paused Acquisition")) -> ()
            n1846 = call "InitializeTrackingParameters.vi"("Rectangular selection"=w2639, "Cancel"=w2638, "Circle fit parameters in"=w2645) -> ("Pupil Marked"=w2644:bool, "Circle fit parameters out"=w2637:T31)  [unwired: 2 in]
            n1847 = Unbundle By Name(w2637) -> ("Rectangle coordinates"=w2636:i32[])
            n1848 = local write "Pupil marked"(w2644) -> ()
            n1849 = call "RectangleToSizeString.vi"("Rectangle Coordinates"=w2636) -> ("Resolution String"=→"Image Size":string)
          }
          event "Save Pupil Video": Value Change {
            # "Check that video is cropped. If not, crop it now"
            n1850 = event-data() -> ("NewVal"=w2646:bool)  [unwired: 1 in]
            n1851 = local read "Pupil marked"() -> (w2649:bool)
            n1852 = Not(x=w2649) -> (.not. x?=w2650:bool)
            n1853 = And(x=w2646, y=w2650) -> (x .and. y?=w2648:bool)
            n1854 = case shown="True" w2648 {
              tunnel: w2653 -> [_ w2658]
              tunnel: w2652 -> [w2654 w2660]
              tunnel: [w2654 w2659] -> w2651
              frame False {
              }
              frame True {
                n1855 = call "IMAQ Select Rectangle"("Prompt"="Crop Eye", "Image In"=w2658) -> ("Cancelled"=w2656:bool, "Rectangle"=w2655:T29)  [unwired: 6 in, 2 out]
                n1856 = call "InitializeTrackingParameters.vi"("Rectangular selection"=w2655, "Cancel"=w2656, "Circle fit parameters in"=w2660) -> ("Pupil Marked"=w2661:bool, "Circle fit parameters out"=w2659:T31)  [unwired: 2 in]
                n1857 = local write "Pupil marked"(w2661) -> ()
              }
            }
          }
          event "Save Tracking Results": Value Change {
            # "Save results from eyetracking to spreadsheet"
            n1858 = event-data() -> ("NewVal"=w2663:bool)  [unwired: 1 in, 1 out]
            n1859 = case shown="True" w2663 {
              tunnel: w2665 -> [w2666 w2669]
              tunnel: [w2666 w2669] -> w2664
              frame False {
              }
              frame True {
                n1860 = local read "RecordingFolder"() -> (w2672:path)
                n1861 = Unbundle By Name(w2669) -> ("Circle time series"=w2670:dbl[][])
                n1862 = call "SaveArrayToTxt.vi"("Input array"=w2670, "Filename"="-eyetracking_results", "File path"=w2672) -> ("Boolean"=w2668:bool)  [unwired: 1 in]
                n1863 = Not(x=w2668) -> (.not. x?=w2667:bool)
                n1864 = local write "Save Tracking Results"(w2667) -> ()
              }
            }
          }
          event "Track Pupil": Value Change {
            n1865 = event-data() -> ("NewVal"=w2676:bool)  [unwired: 1 in, 1 out]
            n1866 = case shown="True" w2676 {
              tunnel: w2675 -> [w2677 w2681]
              tunnel: [w2677 w2680] -> w2674
              frame False {
              }
              frame True {
                n1867 = local read "Manual Threshold"() -> (w2678:cluster{sgl, sgl})
                n1868 = property on="Pupil Info" class="WFChart (strict)"("History Data"=T30 []) -> ()  [unwired: 2 in, 2 out]
                n1869 = call "ResetTrackingParameters.vi"("tracking parameters in"=w2681, "Manual Threshold"=w2678) -> ("tracking parameters out"=w2680:T31)  [unwired: 9 in]
              }
            }
          }
          event "xFactorStdThresholding": Value Change {
            n1870 = event-data() -> ("NewVal"=w2683:dbl)  [unwired: 1 in]
            n1871 = Bundle By Name(cluster=w2684, "mFactorStd"=w2683) -> (w2682:T31)
          }
          event "Automatic Threshold Update": Value Change {
            n1872 = event-data() -> ("NewVal"=w2687:bool)  [unwired: 1 in]
            n1873 = Bundle By Name(cluster=w2688, "Automatic Threshold Update"=w2687) -> (w2686:T31)
          }
          event "Manual Threshold": Value Change {
            n1874 = event-data() -> ("NewVal"=w2692:cluster{sgl, sgl})  [unwired: 1 in]
            n1875 = Unbundle(w2692) -> (w2691:sgl, w2690:sgl)
            n1876 = Build Array(w2691, w2690) -> (w2689:sgl[])
            n1877 = Bundle By Name(cluster=w2695, "Initial Threshold"=w2689, "Auto Threshold"=w2689) -> (w2693:T31)
          }
          event "Acquisition Frame Rate", "Track Every Nth Frame", "Graph Length (s)": Value Change {
            n1878 = event-data() -> ()  [unwired: 1 in, 6 out]
            n1879 = local read "Track Every Nth Frame"() -> (w2700:i32)
            n1880 = local read "Acquisition Frame Rate"() -> (w2701:dbl)
            n1881 = To Double Precision Float(number=w2700) -> (double precision float=w2699:dbl)
            n1882 = Divide(x=w2699, y=w2701) -> (x/y=w2698:dbl)
            n1883 = control-ref of="Pupil Info"() -> (w2697:refnum<vi>)
            n1884 = local read "Graph Length (s)"() -> (w2696:dbl)
            n1885 = call "SetWaveformXscale.vi"("Plot Duration"=w2696, "deltaT"=w2698, "WaveformChart in"=w2697) -> ()  [unwired: 9 in]
          }
          event "Pupil Camera Connected": Value Change {
            n1886 = event-data() -> ()  [unwired: 1 in, 1 out]
            n1887 = local read "Pupil Camera Connected"() -> (w2705:bool)
            n1888 = Not(x=w2705) -> (.not. x?=w2704:bool)
            n1889 = local write "Stop Acquisition"(w2704) -> ()
          }
        }
        n1890 = Unbundle By Name(w2573) -> ("Rectangle coordinates"=w2587:i32[])
        n1891 = local read "Cropped Image"() -> (w2588:T1)
        n1892 = local read "Last Image number"() -> (w2576:u32)
        n1893 = local read "Paused Acquisition"() -> (w2550:bool)
        n1894 = local read "Reset Lost Frames"() -> (w2548:bool)
        n1895 = local read "LostFrames"() -> (w2577:u32)
        n1896 = call "IMAQ Extract 2"("Optional Rectangle"=w2587, "Image Dst"=w2588, "Image Src"=w2582) -> ("Image Dst Out"=w2562:T1)  [unwired: 7 in, 1 out]
        n1897 = call "CheckLostFrames.vi"("Reset Lost Frames In"=w2548, "Pause Acquisition in"=w2550, "Last Image number"=w2576, "Image Number"=w2578, "LostFrames in"=w2577) -> ("Pause Acquisition out"=w2549:bool, "Last Image Number"=w2572:u32, "LostFrames out"=w2552:u32, "Reset Lost Frames Out"=w2547:bool)  [unwired: 3 in]
        n1898 = local write "LostFrames"(w2552) -> ()
        n1899 = local write "Last Image number"(w2572) -> ()
        n1900 = local write "Paused Acquisition"(w2549) -> ()
        n1901 = local write "Reset Lost Frames"(w2547) -> ()
        n1902 = local read "Save Pupil Video"() -> (w2561:bool)
        n1903 = local read "RecordingFolder"() -> (w2559:path)
        n1904 = Greater Than 0?(x=w2552) -> (x > 0?=w2551:bool)
        n1905 = local write "Frames Lost"(w2551) -> ()
        n1906 = call "SavePupilCameraImage.vi"("Save Format"=enum16{"Png", "Raw"}."Raw", "Save Image?"=w2561, "Block Folder"=w2559, "Subfolder"="pupil_video", "Refnum in"=w2562) -> ("Refnum out (duplicate)"=w2557:T1, "ImageSaved"=w2560:bool)  [unwired: 5 in]
        n1907 = local write "Recording Pupil Video"(w2560) -> ()
        n1908 = Quotient & Remainder(x=w2590, y="Track Every Nth Frame") -> (x-y*floor(x/y)=w2586:i32)  [unwired: 1 out]
        n1909 = local read "Track Pupil"() -> (w2570:bool)
        "Tracking Pupil" <- w2570
        n1910 = Equal To 0?(x=w2586) -> (x = 0?=w2571:bool)
        n1911 = And(x=w2571, y=w2570) -> (x .and. y?=w2555:bool)
        n1912 = And(x=w2555, y=FALSE) -> (x .and. y?=w2554:bool)
        n1913 = case shown="True" w2554 {
          tunnel: w2582 -> [w2595 w2618]
          tunnel: w2573 -> [w2594 w2620]
          tunnel: [w2594 w2611] -> w2591
          tunnel: w2562 -> [_ w2619]
          tunnel: w2571 -> [w2593 _]
          tunnel: w2557 -> [_ w2608]
          frame False {
            n1914 = case shown="True" w2593 {
              tunnel: w2595 -> [_ w2597]
              frame False {
              }
              frame True {
                n1915 = local read "Tab Control"() -> (w2596:T9)
                n1916 = case shown="\"Pupil Tracker\"" w2596 {
                  tunnel: w2597 -> [_ w2598]
                  frame "Training", Default {
                  }
                  frame "Pupil Tracker" {
                    n1917 = local write "PupilCamera"(w2598) -> ()
                  }
                }
                n1918 = local write "Image"(w2597) -> ()
              }
            }
          }
          frame True {
            # "Input image refs"
            # "Display results"
            # "Fit Circle"
            # "Fits a circle to the pupil"
            n1919 = local read "Fitted Pupil Image 2"() -> (w2607:T1)
            n1920 = local read "Processed Image Display"() -> (w2614:T1)
            n1921 = local read "Processed Image"() -> (w2621:T1)
            n1922 = local read "Fitted Pupil Image"() -> (w2616:T1)
            n1923 = local read "Mask"() -> (w2605:T1)
            n1924 = local read "Rescan Image"() -> (w2617:bool)
            n1925 = local read "Tab Control"() -> (w2612:T9)
            n1926 = call "IMAQ Copy"("Image Dst"=w2607, "Image Src"=w2608) -> ("Image Dst Out"=w2606:T1)  [unwired: 4 in, 1 out]
            n1927 = call "TrackPupil.vi"("Processed image display refnum"=w2614, "Processed image"=w2621, "Mask refnum"=w2605, "Fitted image refnum"=w2616, "Circle fit parameters in"=w2620, "Rescan image if pupil is lost"=w2617, "Acquired image refnum"=w2618, "Cropped image refnum"=w2619) -> ("Circle fit parameters out"=w2611:T31, "New Values"=→"Pupil Info":T32, "Processed image display refnum out"=w2613:T1, "Fitted image refnum out"=w2623:T1)
            n1928 = Unbundle By Name(w2611) -> ("Auto Threshold"=w2604:sgl[], "Circle time series"=w2610:dbl[][])
            "Auto Threshold" <- w2604
            n1929 = Unbundle By Name(w2611) -> ("Frame No"=w2622:i32)
            n1930 = call "OverlayFittedCircle.vi"("Circle time series"=w2610, "Image"=w2606) -> ("Image Out"=→"Image":T1)  [unwired: 9 in]
            n1931 = case shown="\"Pupil Tracker\"" w2612 {
              tunnel: w2623 -> [_ w2625 _ _]
              tunnel: w2613 -> [_ w2624 _ _]
              frame "Training", Default {
              }
              frame "Pupil Tracker" {
                "PupilCamera" <- w2625
                "Processed" <- w2624
              }
              frame "Manual Rotation" {
              }
              frame "Settings" {
              }
            }
            n1932 = local write "Pupil Sample No"(w2622) -> ()
            n1933 = Index Array(array=w2604, index #1=0 ("index"), index #2=1 ("index")) -> (element #1=w2601:sgl, element #2=w2600:sgl)
            n1934 = Bundle("Numeric"=w2601, "Numeric"=w2600) -> (w2599:cluster{"Numeric":sgl, "Numeric":sgl})  [unwired: 1 in]
            n1935 = local write "Manual Threshold"(w2599) -> ()
          }
        }
      }
      frame "Quit Eyetracker" {
        n1936 = local read "Processed Image"() -> (w2712:T1)
        n1937 = local read "Cropped Image"() -> (w2711:T1)
        n1938 = call "IMAQ Dispose"("Image"=w2712) -> ()  [unwired: 5 in, 1 out]
        n1939 = call "IMAQ Dispose"("Image"=w2711) -> ()  [unwired: 5 in, 1 out]
      }
      frame "Camera Error" {
        n1940 = local read "Vision Acquisition Error"() -> (w2714:errorcluster)
        n1941 = local write "Pupil Camera Connected"(FALSE ("Eye Tracking Camera")) -> ()
        n1942 = call <vilib>:"General Error Handler.vi"("error in (no error)"=w2714) -> ()  [unwired: 10 in, 5 out]
      }
    }
  }
  n1943 = flat-sequence "Trial Variables" {
    frame #0 {
      n1944 = property on="Mouse Performance" class="Arr (strict)"("Visible"=FALSE) -> ()  [unwired: 2 in, 2 out]
      n1945 = property on="Last trial" class="DigNum (strict)"("Visible"=FALSE) -> ()  [unwired: 2 in, 2 out]
      n1946 = property on="Session Performance" class="Arr (strict)"("Visible"=FALSE) -> ()  [unwired: 2 in, 2 out]
    }
  }
  n1947 = flat-sequence "Training Variables" {
    frame #0 {
      # "This variable is plotted"
      n1948 = property on="AllowReward" class="Bool (strict)"("Visible"=FALSE) -> ()  [unwired: 2 in, 2 out]
      n1949 = property on="cue time" class="DigNum (strict)"("Visible"=FALSE) -> ()  [unwired: 2 in, 2 out]
      n1950 = property on="response time" class="DigNum (strict)"("Visible"=FALSE) -> ()  [unwired: 2 in, 2 out]
      n1951 = property on="Response Times" class="Arr (strict)"("Visible"=FALSE) -> ()  [unwired: 2 in, 2 out]
      n1952 = property on="Response Window" class="DigNum (strict)"("Visible"=FALSE) -> ()  [unwired: 2 in, 2 out]
      n1953 = property on="Reward Mode" class="Enum (strict)"("Visible"=FALSE) -> ()  [unwired: 2 in, 2 out]
      n1954 = property on="response window is open" class="Bool (strict)"("Visible"=FALSE) -> ()  [unwired: 2 in, 2 out]
      n1955 = invoke on="NPunishments" class="DigNum (strict)" method="Reinit To Default"() -> ()  [unwired: 3 in, 3 out]
      n1956 = invoke on="NRewards" class="DigNum (strict)" method="Reinit To Default"() -> ()  [unwired: 3 in, 3 out]
      n1957 = invoke on="NGoTrials" class="DigNum (strict)" method="Reinit To Default"() -> ()  [unwired: 3 in, 3 out]
      n1958 = invoke on="Response Times" class="Arr (strict)" method="Reinit To Default"() -> ()  [unwired: 3 in, 3 out]
      n1959 = invoke on="trialData" class="Clust (strict)" method="Reinit To Default"() -> ()  [unwired: 3 in, 3 out]
      "Response Window" <- 0.0 ("Response Window")
    }
  }
  n1960 = flat-sequence "Connection Variables" {
    frame #0 {
    }
  }
  n1961 = flat-sequence "Wall Move Buttons and Variables" {
    frame #0 {
    }
  }
  n1962 = flat-sequence "Stage Move Buttons and Variables" {
    frame #0 {
    }
  }
  n1963 = flat-sequence "LickPort Variables" {
    frame #0 {
      n1964 = disable-structure shown="Disabled" {
        frame Disabled {
          n1965 = invoke on="mL given" class="Slide (strict)" method="Reinit To Default"() -> ()  [unwired: 3 in, 3 out]
        }
        frame Enabled {
        }
      }
      n1966 = property on="Calibration Progress %" class="Slide (strict)"("Visible"=FALSE) -> ()  [unwired: 2 in, 2 out]
    }
  }
  n1967 = local write "Wall Position"(0.0 ("Wall Position")) -> ()
  n1968 = while {
    shift-right: [w2734] -> _
    shift-left: enum16{"Init", "Acquire", "Quit"}."Init" -> [w2732]
    stop <- w2733 stop-if-true
    # "Demo Video"
    n1969 = case shown="\"Acquire\"" w2732 {
      selector: w2732 -> [_ _ w2752]
      tunnel: [w2736 w2749 w2752] -> w2734
      tunnel: [FALSE FALSE TRUE] -> w2733
      frame "Init", Default {
        n1970 = Select(t=enum16{"Init", "Acquire", "Quit"}."Acquire", s="DemoCamera Connected", f=enum16{"Init", "Acquire", "Quit"}."Quit") -> (s? t:f=w2736:enum16{"Init", "Acquire", "Quit"})
      }
      frame "Acquire" {
        n1971 = local read "Exit Program"() -> (w2747:bool)
        n1972 = local read "SaveDemoVideo"() -> (w2745:bool)
        n1973 = call "Vision Acquisition3"("Stop (F)"=w2747) -> ("Image Out"=w2744:T1, "Stopped"=w2746:bool)  [unwired: 23 in, 2 out]
        n1974 = local read "RecordingFolder"() -> (w2742:path)
        n1975 = call "SaveFrameToPNG.vi"("Save Image?"=w2745, "Block Folder"=w2742, "Subfolder"="DemoVideo", "Refnum in"=w2744) -> ("Refnum out (duplicate)"=→"Refnum out (duplicate)":T1, "ImageSaved"=w2740:bool)  [unwired: 6 in]
        n1976 = local write "Recording Demo Video"(w2740) -> ()
        n1977 = Select(t=enum16{"Init", "Acquire", "Quit"}."Quit", s=w2746, f=enum16{"Init", "Acquire", "Quit"}."Acquire") -> (s? t:f=w2749:enum16{"Init", "Acquire", "Quit"})
      }
      frame "Quit" {
      }
    }
  }
  "Reset Lost Frames" <- FALSE ("Reset Lost Frames")
